vi "VR Controler 9.1.vi"() -> ()   [LabVIEW 2017]
uses:
  Sub VIs/Record enum.ctl
  Sub VIs/Socket enum.ctl
  Sub VIs/Main program enum2.ctl
  <vilib>/vision/Image Controls.llb/IMAQ Image.ctl
  e2139745-3a2d-4eca-8046-712b838de117.vi
  b426bb1a-86ec-4bb9-bfac-d02472307ceb.vi
  58126b9d-de85-4f5f-a9a7-01a9de38026e.vi
  c1239b79-c935-4849-aa75-a73d195e7430.vi
  674a1914-568f-4f25-b0a8-01d8120e0c5f.vi
  5779e0b0-41b7-4506-a67f-138f79383ca8.vi
  75927e18-e53a-4ccd-922e-dca7ab16e00a.vi
  6c211394-beff-4d45-9cac-85fa7b8fa806.vi
  1da1cb31-40b1-4a67-a7e6-56ad72bdf787.vi
  <vilib>/DAQmx/write.llb/DAQmx Write (Digital Bool 1Line 1Point).vi
  eb595f88-4225-414f-83f1-01d5d940fc66.vi
  fb6b5c9d-106e-453b-a883-cc93056fac18.vi
  6235507b-2202-4f21-86ca-b7b41428e472.vi
  835dcb76-40d0-41c5-8fe3-3989c1fd9891.vi
  4796a129-a1f4-4c2b-9c8a-39875efc01cf.vi
  bf4008ee-ae26-4c0a-87de-22156137ce73.vi
  cfabecd4-7210-4e1d-87ea-acbfc879dca4.vi
  ec3ac053-eb45-4274-a63b-aef392164dd0.vi
  b14711bf-09ac-44ea-973e-d3b9cd6138c5.vi
  839eb35e-605d-4d61-b8d1-8b601b76a39a.vi
  4b664865-0372-4337-9de9-faa9f3913aab.vi
  63df5311-9246-4ffc-851f-b70ac2e65be5.vi
  <vilib>/DAQmx/read.llb/DAQmx Read (Analog 2D DBL NChan NSamp).vi
  <vilib>/DAQmx/read.llb/DAQmx Read (Digital 2D U8 NChan NSamp).vi
  <vilib>/DAQmx/read.llb/DAQmx Read (Counter 1D DBL 1Chan NSamp).vi
  <vilib>/DAQmx/create/channels.llb/DAQmx Create Channel (DO-Digital Output).vi
  <vilib>/Utility/file.llb/Read Delimited Spreadsheet (string).vi
  <vilib>/DAQmx/create/channels.llb/DAQmx Create Channel (CO-Pulse Generation-Frequency).vi
  <vilib>/DAQmx/configure/timing.llb/DAQmx Timing (Implicit).vi
  <vilib>/DAQmx/miscellaneous.llb/DAQmx Fill In Error Info.vi
  <vilib>/DAQmx/create/channels.llb/DAQmx Create Channel (AI-Voltage-Basic).vi
  <vilib>/DAQmx/create/channels.llb/DAQmx Create Channel (DI-Digital Input).vi
  <vilib>/DAQmx/configure/timing.llb/DAQmx Timing (Sample Clock).vi
  <vilib>/Utility/file.llb/Write Delimited Spreadsheet (string).vi
  6f1d6b9c-7e66-4bfa-a54a-0bf9111e914d.vi
  <resource>/objmgr/daqmx.rc
  f0a6b648-ccd6-4e98-b62c-d3930b5e7adb.vi
  <vilib>/vision/driver/NI_Vision_Acquisition_Software.lvlib
  fa866b4b-dc6c-4481-bc67-f1512cbbaaf9.vi
  <vilib>/DAQmx/configure/task.llb/DAQmx Configure Logging (TDMS).vi
panel:
  out "Write loop stopped":bool
  out "Read loop stopped":bool
  in  "VR Controller":enum32{"Main panel", "Settings"}(tab)
  out "Frame signal indicator 2":bool
  in  "Timed reward (s)":u32
  in  "Various GUI elements":enum32{"Misc", "Eye tracker", "Security camera"}(tab)
  in  "Stimulus cut off (s)":u32=15
  in  "VR start pos":T1(ring)
  out "Opt stim command":dbl[](graph)
  out "Current stim. protocol":string
  out "Random start pos":bool=TRUE
  out "Next trial stim. protocol":string
  in  "start with ramp":bool
  out "stim loop rate":dbl
  out "Pupille image saved":bool
  in  "Record Button 2":bool
  in  "Black Level":dbl(slide)=0.9896907216494839 min=-32.0 max=31.75 step=1.0 scale=-32.0..32.0
  in  "Gain":dbl(slide)=8.879999999999999 min=0.0 max=24.0 step=1.0 scale=0.0..24.0
  in  "Exposure Time (ms)":dbl(slide)=15144.329896907217 min=1.0 max=15.0 scale=0.0..15.0
  in  "Target frame rate":dbl=60.0 min=1.0 max=144.0 step=1.0
  out "Pupille image":T2(plugin-control)
  out "Frame rate":dbl
  in  "Image Format Control::Offset X":i64(slide) min=0 max=450 step=2 scale=0.0..450.0
  in  "Image Format Control::Offset Y":i64(slide) min=0 max=350 step=2 scale=0.0..350.0
  out "Lost Image Count":u32
  out "Total Images Transferred":u32
  out "Security cam image":T2(plugin-control)
  in  "Cam ON /OFF":bool
  out "Stim. count":i32
  in  "Random reward":bool
  out "Frame signal indicator":bool
  in  "Hybrid licking":bool
  in  "Boolean":bool
  in  "SciScan":bool
  in  "Comment":string
  out "Photodiode":bool
  out "Trial type ettings":enum32{"Page 1", "Page 2"}(tab)
  in  "Auto stop recording":bool
  in  "Shuffle stim trials":bool
  out "Session length":u16 max=100
  in  "Block num. 5":u16
  in  "Block 5":u16(ring) items=["Context A", "Context B", "Context C", "Context D", "Context E", "Context F"]
  in  "Block num. 4":u16
  in  "Block 4":u16(ring) items=["Context A", "Context B", "Context C", "Context D", "Context E", "Context F"]
  in  "Block num. 3":u16
  in  "Block 3":u16(ring) items=["Context A", "Context B", "Context C", "Context D", "Context E", "Context F"]
  in  "Block num. 2":u16
  in  "Block 2":u16(ring) items=["Context A", "Context B", "Context C", "Context D", "Context E", "Context F"]
  in  "Block num. 1":u16=1 min=1
  in  "Block 1":u16(ring) items=["Context A", "Context B", "Context C", "Context D", "Context E", "Context F"]
  in  "stim. num. 5":u16
  in  "Stim. prot 5":u16(ring) items=["none", "none", "continuous from 6 to 180 int. 100 % duty cycle 0 %", "continuous from 10 to 200 int. 100 % duty cycle 0 %", "20 Hz sinus from 10 to 20 int. 100 % duty cycle 0 %", "20 Hz sinus from 10 to 70 int. 100 % duty cycle 0 %", "20 Hz sinus from 10 to 0 int. 100 % duty cycle 0 %", "20 Hz sinus from 0 to 70 int. 100 % duty cycle 0 %", "20 Hz sinus from 0 to 70 int. 50 % duty cycle 0 %", "continuous from 10 to 70 int. 100 % duty cycle 0 %"]
  in  "stim. num. 4":u16
  in  "Stim. prot 4":u16(ring) items=["none", "none", "continuous from 6 to 180 int. 100 % duty cycle 0 %", "continuous from 10 to 200 int. 100 % duty cycle 0 %", "20 Hz sinus from 10 to 20 int. 100 % duty cycle 0 %", "20 Hz sinus from 10 to 70 int. 100 % duty cycle 0 %", "20 Hz sinus from 10 to 0 int. 100 % duty cycle 0 %", "20 Hz sinus from 0 to 70 int. 100 % duty cycle 0 %", "20 Hz sinus from 0 to 70 int. 50 % duty cycle 0 %", "continuous from 10 to 70 int. 100 % duty cycle 0 %"]
  in  "stim. num. 3":u16
  in  "Stim. prot 3":u16(ring) items=["none", "none", "continuous from 6 to 180 int. 100 % duty cycle 0 %", "continuous from 10 to 200 int. 100 % duty cycle 0 %", "20 Hz sinus from 10 to 20 int. 100 % duty cycle 0 %", "20 Hz sinus from 10 to 70 int. 100 % duty cycle 0 %", "20 Hz sinus from 10 to 0 int. 100 % duty cycle 0 %", "20 Hz sinus from 0 to 70 int. 100 % duty cycle 0 %", "20 Hz sinus from 0 to 70 int. 50 % duty cycle 0 %", "continuous from 10 to 70 int. 100 % duty cycle 0 %"]
  in  "stim. num. 2":u16
  in  "Stim. prot 2":u16(ring) items=["none", "none", "continuous from 6 to 180 int. 100 % duty cycle 0 %", "continuous from 10 to 200 int. 100 % duty cycle 0 %", "20 Hz sinus from 10 to 20 int. 100 % duty cycle 0 %", "20 Hz sinus from 10 to 70 int. 100 % duty cycle 0 %", "20 Hz sinus from 10 to 0 int. 100 % duty cycle 0 %", "20 Hz sinus from 0 to 70 int. 100 % duty cycle 0 %", "20 Hz sinus from 0 to 70 int. 50 % duty cycle 0 %", "continuous from 10 to 70 int. 100 % duty cycle 0 %"]
  out "stim. num. 1":u16
  out "Stim. prot 1":u16(ring) items=["none", "none", "continuous from 6 to 180 int. 100 % duty cycle 0 %", "continuous from 10 to 200 int. 100 % duty cycle 0 %", "20 Hz sinus from 10 to 20 int. 100 % duty cycle 0 %", "20 Hz sinus from 10 to 70 int. 100 % duty cycle 0 %", "20 Hz sinus from 10 to 0 int. 100 % duty cycle 0 %", "20 Hz sinus from 0 to 70 int. 100 % duty cycle 0 %", "20 Hz sinus from 0 to 70 int. 50 % duty cycle 0 %", "continuous from 10 to 70 int. 100 % duty cycle 0 %"]
  in  "Trial block":u16 max=100
  in  "Primary masking light":T3(ring)
  in  "Enable stim.":bool
  out "GUI version":enum32{"Page 1", "Page 2"}(tab)
  in  "plot selector 1":u16(ring) items=["Context A", "Context B", "Context C", "Context D", "Context E", "Context F"]
  out "?":dbl(slide) scale=0.0..250.0
  in  "Reset top plot":bool=TRUE caption="Reset"
  in  "Reset bottom plot":bool=TRUE caption="Reset"
  out "P stim. Hit":dbl(slide) scale=0.0..1.0
  out "P ctrl. Hit":dbl(slide) scale=0.0..1.0
  out "Control hit trials %":dbl
  out "Stim. hit trials %":dbl
  out "Next":bool
  out "Top Graph":cluster{"Y":dbl[], "Y":dbl[]}[](graph) caption="XY Graph"
  out "Bottom Graph":cluster{"Y":dbl[], "Y":dbl[]}[](graph) caption="XY Graph"
  in  "plot selector bool 1":bool
  in  "plot selector 2":u16(ring) items=["Context A", "Context B", "Context C", "Context D", "Context E", "Context F"]
  in  "plot selector bool 2":bool
  out "Hit trials %":dbl format="%#.1g"
  out "Hit trials":i32
  out "Wheel position graph":cluster{"Y":dbl[], "Y":dbl[]}[](graph) caption="XY Graph"
  in  "Reset wheel pos. graph":bool=TRUE caption="Reset"
  out "P hit trials":dbl(slide) scale=0.0..1.0
  out "Lick and reward chart 2":cluster{dbl, i16}(graph)
  out "%":dbl format="%#_3g"
  in  "Weight":dbl
  in  "Lab book notes":string
  in  "Open valve":bool
  in  "Reward freq. (cm)":u32
  in  "Reward zone":bool
  out "Distance (m)":dbl format="%#.2g"
  in  "Record Button":bool
  in  "Reset water count":bool
  out "Water received (ul)":dbl
  out "All trials":i32
  out "Ctrl. count":i32
  out "Unique ID":i8 format="%2d"
  in  "Stop recording":bool
  in  "Start recording":bool
  out "Laps":i32
  in  "Exit program":bool
  in  "counter reset (F)":bool caption="stop (F)"
  out "Position on the wheel":dbl(knob) scale=0.0..157.0
  in  "Give reward":bool
  in  "Repetition":i32
  out "Date":string
  out "Run experiment":bool
  out "Velocity chart":dbl(graph)
  out "Lick and reward chart":cluster{dbl, i16}(graph)
  out "Record":bool
  out "Time (min)":dbl format="%#.2g"
  in  "Active licking":bool
  out "Mouse name":string
  in  "Scrollbar":i32(c297)
  out "Velocity chart 2":dbl(graph)
  out "Laser ON":bool
  in  "Extra stop triggers":bool
  out "Tab Control hidden Variables":enum32{"Test charts", "Variables"}(tab)
  in  "Gain  2":dbl
  out "Frame signal 2":i8[](array[numeric])
  out "corridor lengths":i32[](array[numeric])
  out "zeward zones":i16[][](array[numeric])
  out "teleports":i16[](array[numeric])
  out "Stim prot command":u16
  out "Context command":u16
  out "ML signal":sgl[](array[numeric])
  out "Pupil Exp day folder":path
  out "settings folder":path
  out "Eyecam states":T4(ring)
  in  "Eable security cam":bool
  out "Eye cam frame signal":i8[](array[numeric])
  out "prev. max stim. V":dbl
  out "prev. stim. type":string
  out "protocol array":string[][](array[string])
  out "analog lick":sgl[](array[numeric])
  out "Encoder signal":sgl[](array[numeric])
  out "Photo stimulus signal":sgl[](array[numeric])
  out "SciScan start":refnum<k21>
  out "Valve signal":i8[](array[numeric])
  out "Trials in session array":u16[][](array[numeric])
  out "Photodiode signal":sgl[](array[numeric])
  out "Frame signal":i8[](array[numeric])
  out "Filename":string
  out "Lab book file":path
  out "Lick indicator":dbl
  out "Encoder count":dbl
  out "Last saved reward size":dbl
  out "Stim types":u16[](array[numeric])
  out "shuffled array":i16[](array[numeric])
  out "Record loop state":T5
  in  "Record enum":T5
  out "Wheel circumference":dbl
  in  "Recording folder":path
  in  "command line":string
  in  "working directory":path=path ""
  out "Start time":u32
  out "Experiment time (ms)":u32
  out "delta time (s)":dbl format="%#.8g"
  out "reward zone end":dbl
  out "Sample rate":dbl
  out "Loop rate":dbl
  out "No. of smpl. per ch.":i32
  out "Original weight":dbl
  out "Laser stimulus calibration":string
  out "Stimulus protocol":string
  out "prev. diode position":dbl
  out "encoder ticks per rev":dbl
  out "Prev. rew. pos.":dbl
  out "Distance (cm)":dbl
  out "miss trial":bool
  out "Session start:":string
  out "hit trial":bool
  out "2P imaging":string
  out "Security camera":string
  out "velocity (cm/s)":dbl
  out "Masking light prot":string
  out "offset tag":string
  out "random rew":dbl
  out "Track position":sgl
  out "start of stim":bool
  in  "Eable eye cam":bool
  out "stim started":bool
  out "Context types":u16[](array[numeric])
  out "Reward given":u32
  out "current VR context":u16
  out "RZ available":bool
  out "User profile":string
  out "Stop Unity":bool
  out "Exit":bool
  out "Stim trial":bool
  out "Trial counted":bool
  in  "select trial":bool
  in  "VR Mode":bool
  out "delta distance cm":dbl[](array[numeric])
  in  "index":i32
  out "lick signal":i8[](array[numeric])
  out "msg tag":string
  out "Header":string
  out "Unity connected":bool
  out "Masking light":bool
  out "Lick":bool
  out "Valve open":bool
  in  "sound cue presented":bool
  out "read":bool
  out "Write":bool
  out "My tdms file":refnum<k34>
  out "Water cnt. reset":i32
  out "Store prev encoder count":dbl
  out "Start mask stim":bool
  out "Start light stim":bool
  out "Stop light stim":bool
  out "Light ON":bool
  out "Stop mask stim":bool
  out "Hit trials stim.":i32
  out "Hit trials ctrl.":i32
  in  "Software version":string
  out "total distance cm":sgl[](array[numeric])
  out "Experiment time (s)":dbl
  out "Analog 3":sgl[](array[numeric])
  out "Waveform Graph":dynamicdata(graph)
  in  "Duty cycle (%)":u8=50 max=100 step=1
  out "Last calibration":string
  in  "Edit mouse list":bool
  out "Socket read loop rate":u32(graph)
  out "Delta time (ms)":u32(graph)
  in  "Sound duration (ms)":u32=25
  in  "Valve open dur. (ms)":u32=25
  in  "Reward size (ul)":dbl min=0.0 step=inf format="%#.2g"
  in  "working directory 2":path=path ""
  out "Reward read loop rate":u32(graph)
  in  "Current mice":string[][](array[string])
  out "Water count":i32
  in  "Stim protocols":u16(ring) items=["none", "none", "continuous from 6 to 180 int. 100 % duty cycle 0 %", "continuous from 10 to 200 int. 100 % duty cycle 0 %", "20 Hz sinus from 10 to 20 int. 100 % duty cycle 0 %", "20 Hz sinus from 10 to 70 int. 100 % duty cycle 0 %", "20 Hz sinus from 10 to 0 int. 100 % duty cycle 0 %", "20 Hz sinus from 0 to 70 int. 100 % duty cycle 0 %", "20 Hz sinus from 0 to 70 int. 50 % duty cycle 0 %", "continuous from 10 to 70 int. 100 % duty cycle 0 %"]
  in  "Stim type":u16(ring) items=["none", "10 Hz sinus", "20 Hz sinus", "40 Hz sinus", "continuous", "10 Hz square", "20 Hz square", "40 Hz square"]
  in  "Intensity (%)":u8=100 max=100 step=1
  in  "stop (cm)":i32
  in  "start (cm)":i32
  out "Waveform Chart":dbl(graph)
  # "All"
  # "This session"
  # "Reward conditions"
  # "Trial type settings"
  # "Hit trials:"
  # "%"
  # "Hit trials:"
  # "%"
  # "%"
  # "Edit stimulus protocols for photo stimulation and/or \na secondary masking light. Chose a protocol from the \nlist and define parameters."
  # "Reward settings"
  # "Mouse name               Headbar           Original weight"
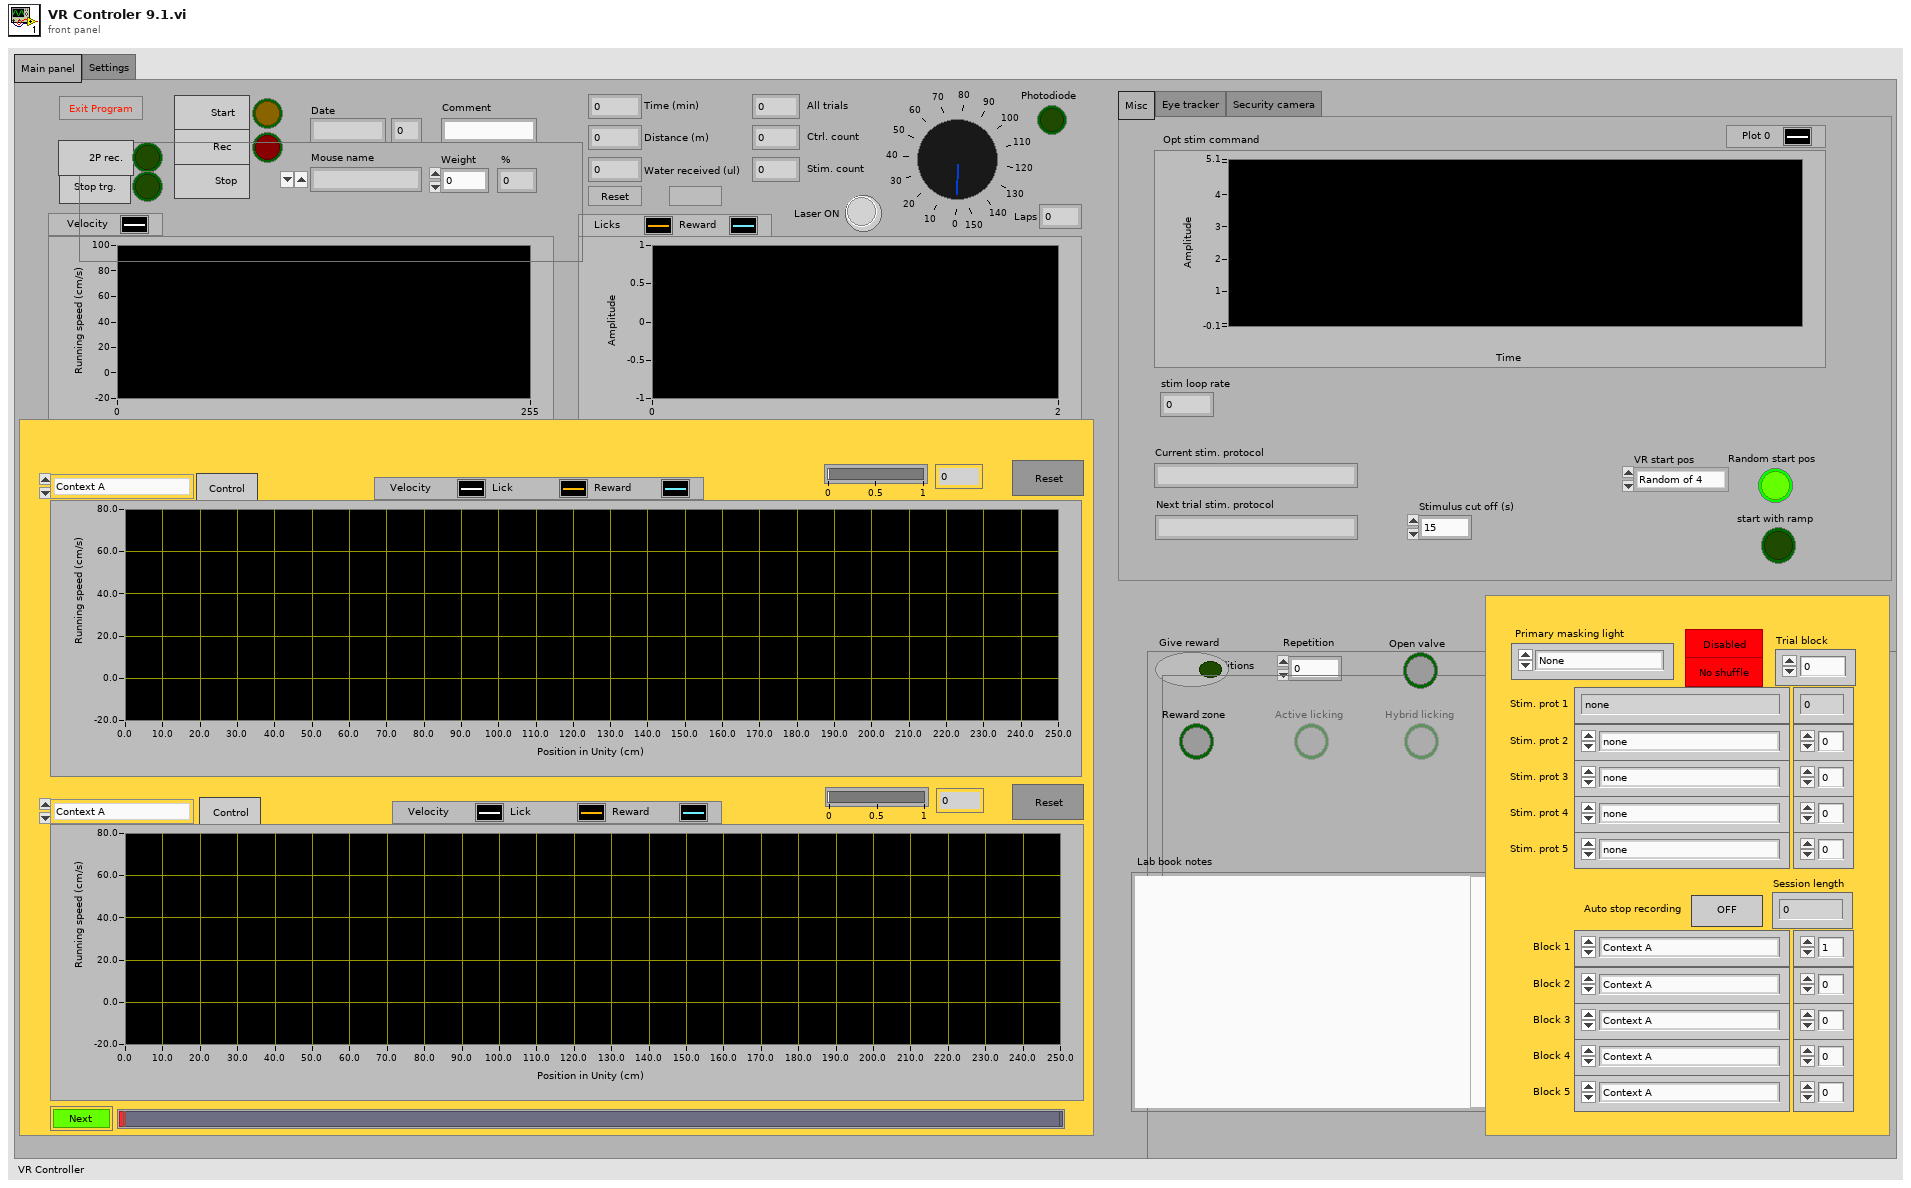
[diagram p1: front panel]
types:
  T1 = enum16{"Random of 4", "Random of 2", "Non-random"}
  T2 = typedef "IMAQ Image.ctl" = refnum<image>
  T3 = enum16{"None", "20 Hz until reward ", "Continuous specified light off trials", "Continuous specified all trials", "20 Hz specified light off trials", "20 Hz specified all trials", "20 Hz full trial", "Continuous full trial"}
  T4 = enum16{"Idle", "Set params", "Start recording", "Record pupille", "Stop recording"}
  T5 = typedef "Record enum.ctl" = enum16{"Idle", "Init recording", "Init data acquisition", "Record VR", "Record", "Stop data acquision"}
  T6 = enum8{"Enabled", "Disabled", "Disabled and Grayed Out"}
  T7 = typedef "Main program enum2.ctl" = enum16{"Init program", "Idle", "Init recording ", "Record", "Record VR", "Stop Recording", "Exit program"}
  T8 = typedef "Socket enum.ctl" = enum16{"Socket not connected", "Init socket", "Socket connected", "Close socket"}
  T9 = cluster{"Type":u32, "Version":u32, "Flags":u32, "SerialNumberHigh":u32, "SerialNumberLow":u32, "BusType":u32, "InterfaceName":string, "VendorName":string, "ModelName":string, "CameraFileName":string, "CameraAttributeURL":string}[]
  T10 = enum16{"open", "replace", "create", "open or create", "replace or create", "replace or create with confirmation"}
  T11 = enum16{"Init program", "Idle", "Init recording ", "Record", "Record VR", "Stop Recording", "Exit program"}
  T12 = enum16{"None", "Full trial 40 Hz sinus ", "Full trial 20 Hz sinus", "Continuous light ON", "Until reward 40 Hz sinus"}
  T13 = enum16{"None", "20 Hz until reward ", "Continuous specified light off trials", "Continuous specified all trials", "20 Hz specified light off trials", "20 Hz specified all trials"}
  T14 = typedef "LVStringsAndValuesArrayTypeDef_U16.ctl" = cluster{"String":string, "Value":u16}[]
  T15 = enum16{"open", "open or create", "create or replace", "create", "open (read-only)"}
  T16 = enum16{"Standard", "Buffered", "CRLF", "Immediate"}
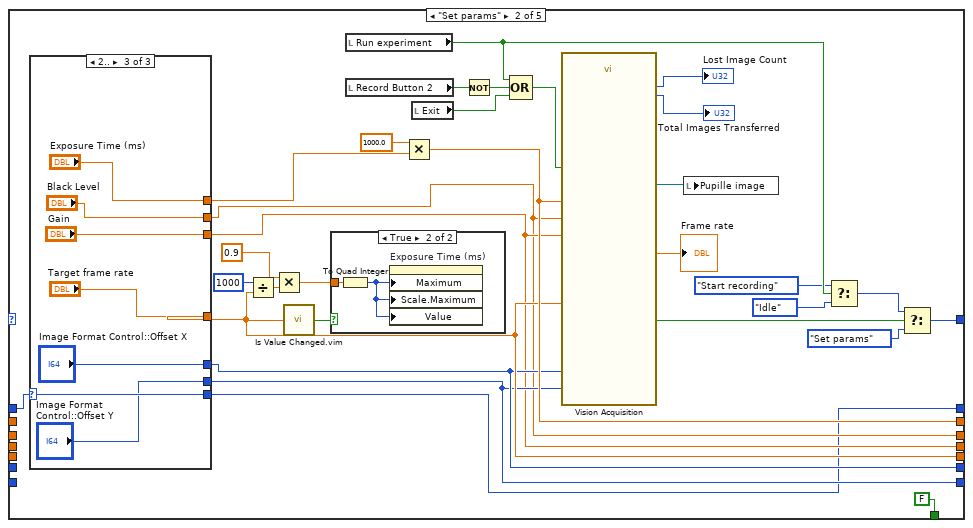
[diagram p3: hidden frame]
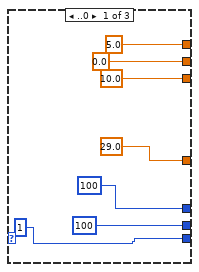
[diagram p4: hidden frame]
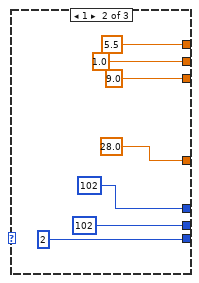
[diagram p5: hidden frame]
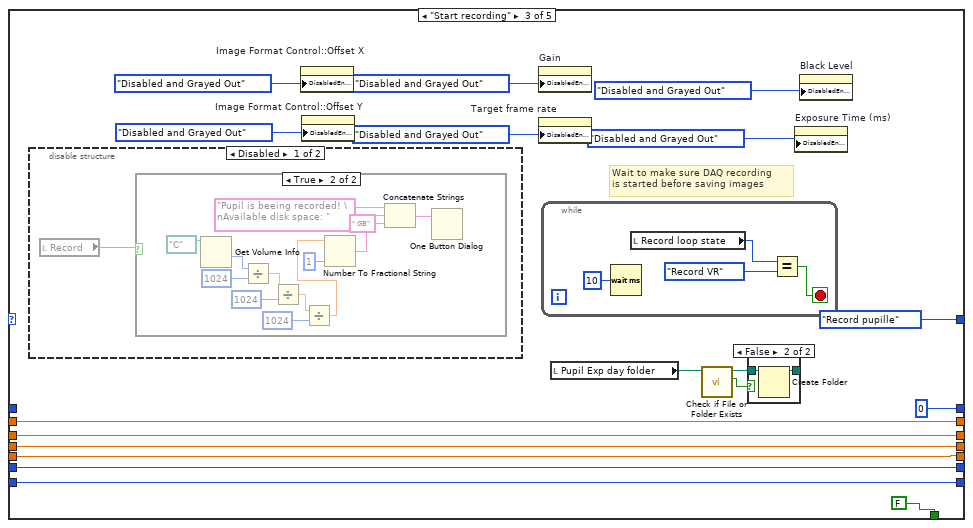
[diagram p7: hidden frame]
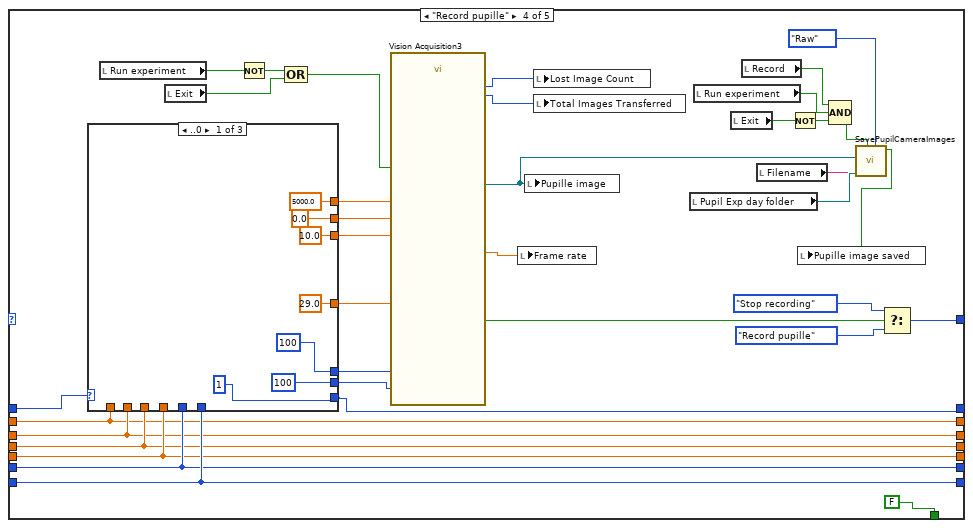
[diagram p11: hidden frame]
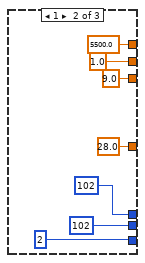
[diagram p12: hidden frame]
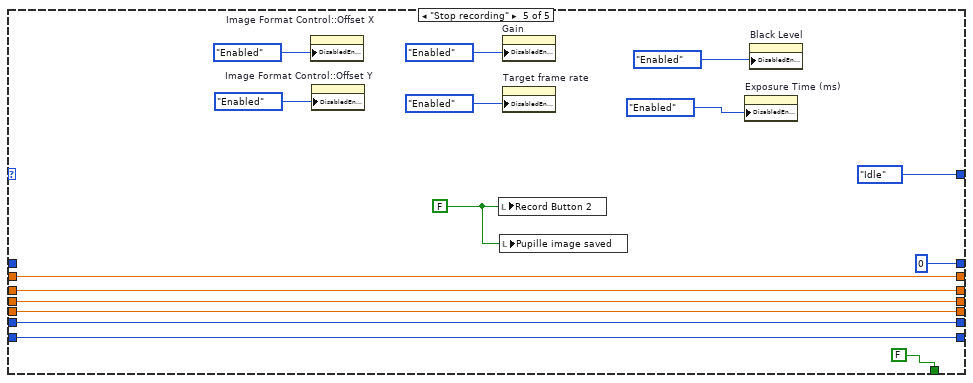
[diagram p14: hidden frame]
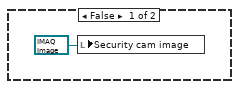
[diagram p15: hidden frame]
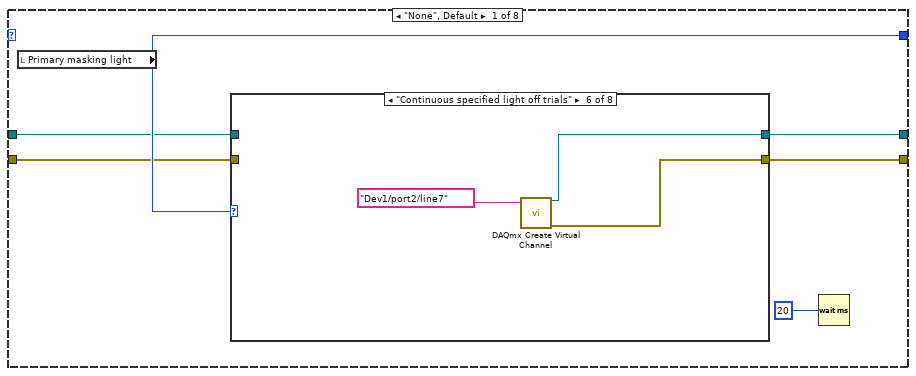
[diagram p19: hidden frame]
diagram:
  w5 = T6."Enabled" ("Disabled")
  w15 = FALSE ("Eable eye cam")
  w16 = FALSE ("Record Button 2")
  w17 = 60 ("y")
  w43 = "rew" ("regular expression")
  w41 = "rew" ("regular expression")
  w35 = "continuous" ("regular expression")
  w37 = "none" ("regular expression")
  w55 = "rew" ("regular expression")
  w57 = "rew" ("regular expression")
  w63 = "continuous" ("regular expression")
  w61 = "none" ("regular expression")
  (unwired) string[] ["Photo-diode", "Time (s)", "Delta Time (ms)", "Distance (cm)", "Valve open", "Frame signal", "Lick signal", "Photo stimulus signal", "Laser ON", "Position in Unity", "Corridor indicator"] ("channel name(s) in (Untitled)")
  w80 = FALSE ("Reset")
  # "Defaults"
  # "Keep order of default variables:\nUser:\tMate\nLoop rate:\t100\nSampling rate:\t3000\nEncoder tisks:\t4000\nRecording folder:\tC:\\Users\\vrsetup\\Desktop\nEnable VR more(Y/N):\tY\n..."
  # "File versions:\n-8.5 User profile selector\n\n-8.3 Camera control added> Pupil imaging and security camera\nTimed reward\n\n-8.2 with 8.4 unity version: \nNew task without cue\nImportant bugfixes in photo-stimulation, start stimulus with ramp option is added\nSafety switch shuts off stimulus after 10s \n\n-8.0 - 8.2\nNew task wersionm new optogenetic prorocol solutions\n\n-7.5 - 2019.07.10\nRandom reward option\n\n-7.5\nNew Unity version: coupling error is corrected! (interpolation factor discarded), randomizeable starting point.\nTiki-taka task for Nora\nNew masking light functions : 20Hz specified in light off or all trials\n\n\n-7.3\nMasking light options are added\nMasking light protocol is saved now in labbook\n\n-7.2\nmade GitHub compatible: folder path and some default variables are red from txt file and txt data files are now in separate folder\ndate is formated with different method\n\n-7.1\nsaves Encoder signal and imaging/security camera YES NO indication is added to lab book\nsaves Analog lick signal\n\n-7.0 \nMasking light\n\n-6.9\nData typed are changed back to DBL\n\n-6.8\nDifferent data saving settings to reduce file size by specifying data types\nCorrect trial % corrected after 2018.12.05\nHybrid licking\nPhoto stimulus trials and counting of \"Hit trials \"for Nora\n\n-6.7 \nfor Mate Loop rate from 200 -> 100 Hz  (should not affect VR that is 60 Hz) \nrecorded sampling rate increased 200 -> 3000 Hz\nswitch to show water consumption in current session is added\n\n\n\n..."
  n1 = flat-sequence {
    tunnel: [w118] -> w11
    tunnel: w11 -> [w154]
    tunnel: [Socket_enum."Socket not connected" ("Enum")] -> w112
    tunnel: [Main_program_enum2."Init program" ("main program")] -> w111
    tunnel: [Record_enum."Idle" ("Record enum")] -> w108
    tunnel: [TRUE ("VR Mode")] -> w79
    frame #0 {
      # "Select user profile"
      n2 = call <vilib>:"Recursive File List.vi"("Folder Path"=path "C:/VR Controller/data" ("path")) -> ("All Folders"=w127:path[])  [unwired: 6 in, 4 out]
      n3 = Array Size(array=w127) -> (size(s)=w132:i32)
      n4 = for {
        N: w132 -> [_]
        tunnel: w127 -> [w143] mode=indexing
        shift-right: [w140] -> w129
        shift-left: string[] [] -> [w139]
        i -> [w141]
        n5 = Strip Path(path=w143) -> (name=w142:string)  [unwired: 1 out]
        n6 = Insert Into Array(array=w139, index=w141, new element=w142) -> (w140:string[])
      }
      n7 = Array Size(array=w129) -> (size(s)=w121:i32)
      n8 = Greater?(x=w121, y=1) -> (0:w119:bool)
      n9 = Array Subset(array=w129, index=1, length=w121) -> (w128:string[])
      n10 = case shown="True" w119 {
        tunnel: w128 -> [_ w138]
        tunnel: w127 -> [_ w137]
        tunnel: [path "" ("path") w134] -> w123
        frame False {
        }
        frame True {
          n11 = call "Get User Input.vi"("Strings []"=w138) -> ("user"=w136:u16)  [unwired: 1 in, 9 out]
          n12 = Increment(x=w136) -> (x+1=w135:u16)
          n13 = Index Array(array=w137, index=w135) -> (element=w134:path)
        }
      }
      n14 = Equal?(x=w123, y=path "" ("path")) -> (x = y?=w125:bool)
      n15 = Select(t=path "C:/VR Controller/data", s=w125, f=w123) -> (s? t:f=w118:path)
      "settings folder" <- w118
      n16 = Path To String(path=w118) -> (string=w117:string)
      n17 = Match Pattern(string=w117, regular expression="data\\") -> (after substring=→"User profile":string)  [unwired: 1 in, 3 out]
    }
    frame #1 {
      w159 = 1 ("length")
      w164 = 1 ("length")
      w177 = 1 ("length")
      w180 = 1 ("length")
      w183 = 1 ("length")
      w186 = 1 ("length")
      # "VI version"
      # "Enable VR mode"
      n18 = Build Path(base path=w154, name or relative path="Default variables.txt") -> (appended path=w152:path)
      n19 = call-poly <vilib>:"Read Delimited Spreadsheet.vi"("file path (dialog if empty)"=w152) -> ("all rows"=w155:string[][])  [unwired: 9 in, 5 out]
      n20 = Array Subset(array=w155, index (row)=0 ("index"), length (row)=w186, index (col)=w186, length (col)=w186) -> (w185:string[][])
      n21 = Array Subset(array=w155, index (row)=1 ("index"), length (row)=w183, index (col)=w183, length (col)=w183) -> (w184:string[][])
      n22 = Array Subset(array=w155, index (row)=2 ("index"), length (row)=w164, index (col)=w164, length (col)=w164) -> (w161:string[][])
      n23 = Array Subset(array=w155, index (row)=3 ("index"), length (row)=w180, index (col)=w180, length (col)=w180) -> (w179:string[][])
      n24 = Array Subset(array=w155, index (row)=4 ("index"), length (row)=w177, index (col)=w177, length (col)=w177) -> (w178:string[][])
      n25 = Array Subset(array=w155, index (row)=5 ("index"), length (row)=w159, index (col)=w159, length (col)=w159) -> (w158:string[][])
      n26 = Concatenate Strings(w185) -> (w171:string)
      n27 = Concatenate Strings(w184) -> (w173:string)
      n28 = Concatenate Strings(w161) -> (w165:string)
      n29 = Concatenate Strings(w179) -> (w174:string)
      n30 = Concatenate Strings(w178) -> (w175:string)
      n31 = Concatenate Strings(w158) -> (w157:string)
      n32 = String To Path(string=w175) -> (path=w148:path)
      n33 = Fract/Exp String To Number(string=w165) -> (number=w162:dbl)  [unwired: 3 in, 1 out]
      n34 = Fract/Exp String To Number(string=w174) -> (number=w169:dbl)  [unwired: 3 in, 1 out]
      n35 = Fract/Exp String To Number(string=w173) -> (number=w170:dbl)  [unwired: 3 in, 1 out]
      n36 = Equal?(x=w171, y=" ") -> (x = y?=w146:bool)
      n37 = Equal?(x=w157, y="Y") -> (x = y?=w145:bool)
      n38 = case shown="True" w145 {
        tunnel: w155 -> [_ w195]
        tunnel: [path "" w198] -> w147
        frame False {
          (unwired) FALSE ("T button?")
        }
        frame True {
          w196 = 1 ("length")
          w202 = 1 ("length")
          # "Default context"
          n39 = Array Subset(array=w195, index (row)=6 ("index"), length (row)=w202, index (col)=w202, length (col)=w202) -> (w200:string[][])
          n40 = Array Subset(array=w195, index (row)=7 ("index"), length (row)=w196, index (col)=w196, length (col)=w196) -> (w194:string[][])
          n41 = Concatenate Strings(w200) -> (w199:string)
          n42 = Concatenate Strings(w194) -> (w193:string)
          n43 = local write "command line"(w199) -> ()
          n44 = String To Path(string=w199) -> (path=w198:path)
          n45 = Decimal String To Number(string=w193) -> (number=w192:i32)  [unwired: 2 in, 1 out]
          n46 = local write "Block 1"(w192) -> ()
          n47 = local write "plot selector 1"(w192) -> ()
        }
      }
      n48 = local write "Loop rate"(w170) -> ()
      n49 = local write "Sample rate"(w162) -> ()
      n50 = local write "encoder ticks per rev"(w169) -> ()
      n51 = local write "Recording folder"(w148) -> ()
      n52 = case shown="True" w146 {
        frame False {
          n53 = local write "Sound duration (ms)"(u32 0 ("Sound duration (ms)")) -> ()
        }
        frame True {
          n54 = local write "Sound duration (ms)"(u32 0 ("Sound duration (ms)")) -> ()
        }
      }
      n55 = local write "VR Mode"(w145) -> ()
      n56 = Current VI's Path() -> (path=w151:path)
      n57 = case shown="True" TRUE {
        tunnel: [enum32{"Page 1", "Page 2"}."Page 2" ("GUI version") w233] -> w189
        tunnel: [enum32{"Page 1", "Page 2"}."Page 1" ("GUI version") w233] -> w188
        frame False {
          n58 = property on="Top Graph" class="XYGraph (strict)"("DisabledEnum"=T6."Disabled" ("Disabled")) -> ()  [unwired: 2 in, 2 out]
          n59 = property on="Bottom Graph" class="XYGraph (strict)"("DisabledEnum"=T6."Disabled" ("Disabled")) -> ()  [unwired: 2 in, 2 out]
          n60 = property on="Wheel position graph" class="XYGraph (strict)"("DisabledEnum"=T6."Enabled" ("Disabled")) -> ()  [unwired: 2 in, 2 out]
          n61 = property on="Lick and reward chart" class="WFChart (strict)"("Visible"=FALSE, "DisabledEnum"=T6."Disabled" ("Disabled")) -> ()  [unwired: 2 in, 2 out]
          n62 = property on="Velocity chart" class="WFChart (strict)"("Visible"=FALSE, "DisabledEnum"=T6."Disabled" ("Disabled")) -> ()  [unwired: 2 in, 2 out]
          n63 = property on="Reset top plot" class="Bool (strict)"("DisabledEnum"=T6."Disabled" ("Disabled")) -> ()  [unwired: 2 in, 2 out]
          n64 = property on="Reset wheel pos. graph" class="Bool (strict)"("DisabledEnum"=T6."Enabled" ("Disabled")) -> ()  [unwired: 2 in, 2 out]
          n65 = property on="Reset bottom plot" class="Bool (strict)"("DisabledEnum"=T6."Disabled" ("Disabled")) -> ()  [unwired: 2 in, 2 out]
          n66 = property on="Lick and reward chart 2" class="WFChart (strict)"("Visible"=TRUE, "DisabledEnum"=T6."Enabled" ("Disabled")) -> ()  [unwired: 2 in, 2 out]
          n67 = property on="Velocity chart 2" class="WFChart (strict)"("Visible"=TRUE, "DisabledEnum"=T6."Enabled" ("Disabled")) -> ()  [unwired: 2 in, 2 out]
        }
        frame True {
          w233 = enum32{"Page 1", "Page 2"}."Page 1" ("GUI version")
          n68 = property on="Lick and reward chart" class="WFChart (strict)"("Visible"=TRUE, "DisabledEnum"=T6."Enabled" ("Disabled")) -> ()  [unwired: 2 in, 2 out]
          n69 = property on="Velocity chart" class="WFChart (strict)"("Visible"=TRUE, "DisabledEnum"=T6."Enabled" ("Disabled")) -> ()  [unwired: 2 in, 2 out]
          n70 = property on="Top Graph" class="XYGraph (strict)"("DisabledEnum"=T6."Enabled" ("Disabled")) -> ()  [unwired: 2 in, 2 out]
          n71 = property on="Bottom Graph" class="XYGraph (strict)"("DisabledEnum"=T6."Enabled" ("Disabled")) -> ()  [unwired: 2 in, 2 out]
          n72 = property on="Wheel position graph" class="XYGraph (strict)"("DisabledEnum"=T6."Disabled" ("Disabled")) -> ()  [unwired: 2 in, 2 out]
          n73 = property on="Reset top plot" class="Bool (strict)"("DisabledEnum"=T6."Enabled" ("Disabled")) -> ()  [unwired: 2 in, 2 out]
          n74 = property on="Reset wheel pos. graph" class="Bool (strict)"("DisabledEnum"=T6."Disabled" ("Disabled")) -> ()  [unwired: 2 in, 2 out]
          n75 = property on="Reset bottom plot" class="Bool (strict)"("DisabledEnum"=T6."Enabled" ("Disabled")) -> ()  [unwired: 2 in, 2 out]
          n76 = property on="Lick and reward chart 2" class="WFChart (strict)"("Visible"=FALSE, "DisabledEnum"=T6."Disabled" ("Disabled")) -> ()  [unwired: 2 in, 2 out]
          n77 = property on="Velocity chart 2" class="WFChart (strict)"("Visible"=FALSE, "DisabledEnum"=T6."Disabled" ("Disabled")) -> ()  [unwired: 2 in, 2 out]
        }
      }
      "GUI version" <- w189
      "Trial type ettings" <- w188
      n78 = Strip Path(path=w147) -> (name=w149:string)  [unwired: 1 out]
      n79 = Strip Path(path=w151) -> (name=w150:string)  [unwired: 1 out]
      n80 = disable-structure shown="Disabled" {
        frame Disabled {
          n81 = local write "command line"("C:\\VR Controller\\corridor1\\LVcontrol_6.exe" ("command line")) -> ()
        }
        frame Enabled {
        }
      }
      n82 = case shown="True" w145 {
        tunnel: ["" ("string") w205] -> w167
        tunnel: w149 -> [_ w204]
        frame False {
        }
        frame True {
          n83 = Concatenate Strings(";    Unity VR version: " ("string"), w204) -> (w205:string)
        }
      }
      n84 = Concatenate Strings(w150, w167, "" ("string")) -> (w168:string)
      n85 = local write "Software version"(w168) -> ()
    }
    frame #2 {
      # "Has to be integer!"
      n86 = call <vilib>:"IMAQdx Enumerate Cameras.vi"() -> ("Camera Information Array"=w243:T9)  [unwired: 10 in, 1 out]
      n87 = local read "Sample rate"() -> (w242:dbl)
      n88 = for {
        tunnel: w243 -> [w255] mode=indexing
        # "Eye camera available"
        # "Security camera available"
        n89 = Unbundle By Name(w255) -> ("VendorName"=w252:string)
        n90 = Equal?(x="Microsoft® LifeCam Studio(TM)", y=w252) -> (x = y?=w250:bool)
        n91 = Equal?(x=w252, y="Basler") -> (x = y?=w251:bool)
        n92 = case shown="True" w250 {
          selector: w250 -> [_ w256]
          frame False {
          }
          frame True {
            n93 = local write "Eable security cam"(w256) -> ()
            n94 = property on="Cam ON /OFF" class="Bool (strict)"("DisabledEnum"=T6."Enabled" ("Disabled")) -> ()  [unwired: 2 in, 2 out]
          }
        }
        n95 = case shown="True" w251 {
          selector: w251 -> [_ w258]
          frame False {
          }
          frame True {
            n96 = local write "Eable eye cam"(w258) -> ()
            n97 = property on="Record Button 2" class="Bool (strict)"("DisabledEnum"=T6."Enabled" ("Disabled")) -> ()  [unwired: 2 in, 2 out]
          }
        }
      }
      n98 = local read "Loop rate"() -> (w246:dbl)
      n99 = Divide(x=w242, y=w246) -> (x/y=w247:dbl)
      n100 = Divide(x=1.0, y=w242) -> (x/y=w240:dbl)
      n101 = local write "No. of smpl. per ch."(w247) -> ()
      n102 = property on="Opt stim command" class="WFChart (strict)"("XScale.Multiplier"=w240) -> ()  [unwired: 2 in, 2 out]
    }
  }
  n103 = property on="Software version" class="Str"("Visible"=TRUE) -> ()  [unwired: 2 in, 2 out]
  n104 = disable-structure shown="Disabled" {
    frame Disabled {
      n105 = call-poly <vilib>:"DAQmx Configure Logging.vi"() -> ()  [unwired: 14 in, 2 out]
    }
    frame Enabled {
    }
  }
  n106 = disable-structure shown="Disabled" {
    frame Disabled {
      n107 = local read "Unity connected"() -> (w260:bool)
      n108 = case shown="False" w260 {
        frame False {
          n109 = case shown="True" {
            selector: _ -> [_ _]
            frame False {
            }
            frame True {
              n110 = call <vilib>:"System Exec.vi"("wait until completion? (T)"=FALSE, "working directory"="working directory", "command line"="command line") -> ()  [unwired: 5 in, 4 out]
              n111 = Wait (ms)(milliseconds to wait=u32 1000) -> ()  [unwired: 1 out]
            }
          }
        }
        frame True {
        }
      }
    }
    frame Enabled {
    }
  }
  n112 = local write "Eable security cam"(w15) -> ()
  n113 = local write "Eable eye cam"(w15) -> ()
  n114 = property on="Cam ON /OFF" class="Bool (strict)"("DisabledEnum"=T6."Disabled and Grayed Out" ("Disabled")) -> ()  [unwired: 2 in, 2 out]
  n115 = property on="Record Button 2" class="Bool (strict)"("DisabledEnum"=T6."Disabled and Grayed Out" ("Disabled")) -> ()  [unwired: 2 in, 2 out]
  n116 = local write "msg tag"("str," ("msg tag")) -> ()
  n117 = local write "Security camera"("Security camera: NO" ("Security camera")) -> ()
  n118 = Multiply(x=50.0, y=3.141592653589793) -> (x*y=→"Wheel circumference":dbl)
  n119 = Divide(x=1000, y=w17) -> (x/y=w19:dbl)
  n120 = property on="lick signal" class="Arr (strict)"("Visible"=TRUE) -> ()  [unwired: 2 in, 2 out]
  n121 = property on="Header" class="Str"("Visible"=TRUE) -> ()  [unwired: 2 in, 2 out]
  n122 = disable-structure shown="Disabled" {
    frame Disabled {
      n123 = Add Array Elements() -> (numeric array=w267:dbl[], sum=w266:dbl)
      n124 = Array Size(array=w267) -> (size(s)=w265:i32)
      n125 = Divide(x=w266, y=w265) -> ()  [unwired: 1 out]
    }
    frame Enabled {
    }
  }
  n126 = local write "Target frame rate"(w17) -> ()
  n127 = local write "Write loop stopped"(TRUE ("Read loop stopped")) -> ()
  n128 = local write "Read loop stopped"(TRUE ("Read loop stopped")) -> ()
  n129 = property on="Read loop stopped" class="Bool (strict)"("Visible"=FALSE) -> ()  [unwired: 2 in, 2 out]
  n130 = property on="Write loop stopped" class="Bool (strict)"("Visible"=FALSE) -> ()  [unwired: 2 in, 2 out]
  n131 = Multiply(x=0.9, y=w19) -> (x*y=w21:dbl)
  n132 = local write "Recording folder"("Recording folder") -> ()
  n133 = To Quad Integer(1:w21) -> (0:w22:i64)
  n134 = Get Date/Time String(date format (0)=enum16{"short", "long", "abbreviated"}."short") -> ()  [unwired: 2 in, 2 out]
  n135 = property on="delta distance cm" class="DigNum (strict)"("Visible"=TRUE) -> ()  [unwired: 2 in, 2 out]
  n136 = local write "Encoder count"(0.0 ("Encoder count")) -> ()
  n137 = property on="Lab book file" class="Path"("Visible"=TRUE) -> ()  [unwired: 2 in, 2 out]
  n138 = local write "Record Button 2"(w16) -> ()
  n139 = local write "Pupille image saved"(w16) -> ()
  n140 = property on="index" class="DigNum (strict)"("Visible"=TRUE) -> ()  [unwired: 2 in, 2 out]
  n141 = property on="Exposure Time (ms)" class="Slide (strict)"("Maximum"=w22, "Scale.Maximum"=w22, "Value"=w22) -> ()  [unwired: 2 in, 2 out]
  n142 = while {
    shift-right: [w268] -> _
    shift-left: w111 -> [w270]
    stop <- w271 stop-if-true
    n143 = case shown="\"Init recording \"" w270 {
      tunnel: [T11."Idle" ("main program") w475 w766 T11."Idle" ("main program") T11."Idle" ("main program") w878 w973] -> w268
      frame "Init program", Default {
        w273 = 1 ("y")
        (unwired) path "C:/Users/Mate Neubrandt/Desktop/test/Task config" ("path")
        w319 = u16 0 items=["none"] ("Stim. prot 1")
        w320 = u16 0 ("stim. num. 2")
        n144 = local read "settings folder"() -> (w316:path)
        n145 = local write "Unique ID"(i8 0 ("Unique ID")) -> ()
        n146 = local write "Run experiment"(FALSE ("Record")) -> ()
        n147 = local write "SciScan"(FALSE ("SciScan")) -> ()
        n148 = local write "Edit mouse list"(FALSE ("Edit mouse list")) -> ()
        n149 = local write "Trial block"(u16 10 ("Denominator")) -> ()
        n150 = Build Path(base path=w316, name or relative path="List of mice.txt") -> (appended path=w315:path)
        n151 = property on="Stop recording" class="Bool (strict)"("DisabledEnum"=T6."Disabled" ("Disabled")) -> ()  [unwired: 2 in, 2 out]
        n152 = call-poly <vilib>:"DAQmx Create Virtual Channel.vi"("lines"=tag "Dev1/port0/line0") -> ("task out"=→"SciScan start":refnum<k21>)  [unwired: 13 in, 1 out]
        n153 = call-poly <vilib>:"Read Delimited Spreadsheet.vi"("file path (dialog if empty)"=w315) -> ("all rows"=w341:string[][])  [unwired: 9 in, 5 out]
        n154 = local write "stim. num. 2"(w320) -> ()
        n155 = local write "stim. num. 3"(w320) -> ()
        n156 = local write "stim. num. 4"(w320) -> ()
        n157 = local write "stim. num. 5"(w320) -> ()
        n158 = local write "Block num. 2"(w320) -> ()
        n159 = local write "Block num. 3"(w320) -> ()
        n160 = local write "Block num. 4"(w320) -> ()
        n161 = local write "Block num. 5"(w320) -> ()
        n162 = local write "Current mice"(w341) -> ()
        n163 = flat-sequence {
          frame #0 {
            n164 = property on="Stim protocols" class="Ring (strict)"("Strings []"=string[] []) -> ()  [unwired: 2 in, 2 out]
          }
          frame #1 {
            n165 = local read "settings folder"() -> (w346:path)
            n166 = Build Path(base path=w346, name or relative path="Stimprotocols.txt") -> (appended path=w344:path)
            n167 = call-poly <vilib>:"Read Delimited Spreadsheet.vi"("file path (dialog if empty)"=w344) -> ("all rows"=w349:string[][])  [unwired: 9 in, 5 out]
            "protocol array" <- w349
            n168 = Array Size(array=w349) -> (size(s)=w352:i32[])
            n169 = Index Array(array=w352, index=0) -> (element=w350:i32)
            n170 = for {
              N: w350 -> [_]
              tunnel: w349 -> [w363] mode=indexing
              shift-right: [w361] -> w347
              shift-left: string[] [] -> [w360]
              i -> [w362]
              n171 = Concatenate Strings(w363) -> (w357:string)
              n172 = Match Pattern(string=w357, regular expression="none") -> (before substring=w355:string, match substring=w354:string)  [unwired: 1 in, 2 out]
              n173 = Not Equal?(x=w354, y="none") -> (x != y?=w356:bool)
              n174 = Select(t=w355, s=w356, f=w354) -> (s? t:f=w353:string)
              n175 = Insert Into Array(array=w360, index=w362, new element=w353) -> (w361:string[])
            }
            n176 = property on="Stim protocols" class="Ring (strict)"("Strings []"=w347) -> ()  [unwired: 2 in, 2 out]
          }
        }
        n177 = local write "Enable stim."(TRUE ("Enable stim.")) -> ()
        n178 = local write "Stim. prot 2"(w319) -> ()
        n179 = local write "Stim. prot 3"(w319) -> ()
        n180 = local write "Stim. prot 4"(w319) -> ()
        n181 = local write "Stim. prot 5"(w319) -> ()
        n182 = local write "Block 2"(w319) -> ()
        n183 = local write "Block 3"(w319) -> ()
        n184 = local write "Block 4"(w319) -> ()
        n185 = local write "Block 5"(w319) -> ()
        n186 = local read "command line"() -> (w303:string)
        n187 = local read "settings folder"() -> (w279:path)
        n188 = local read "settings folder"() -> (w314:path)
        n189 = Build Path(base path=w279, name or relative path="Task configuration.txt") -> (appended path=w278:path)
        n190 = Match Pattern(string=w303, regular expression=".exe") -> (before substring=w301:string)  [unwired: 1 in, 3 out]
        n191 = call-poly <vilib>:"Read Delimited Spreadsheet.vi"("file path (dialog if empty)"=w278) -> ("all rows"=w310:string[][])  [unwired: 9 in, 5 out]
        n192 = Concatenate Strings(w301, "_config" ("string")) -> (w299:string)
        n193 = Build Path(base path=w314, name or relative path="Last calibration.txt") -> (appended path=w312:path)
        n194 = Build Path(name or relative path=w299) -> ()  [unwired: 1 in, 1 out]
        n195 = Delete From Array(array=w310, length=1, index (col)=0 ("disabled index (col)")) -> (deleted portion=w307:string[][], array with subset deleted=w296:string[][])  [unwired: 1 in]
        n196 = Decimal String To Number(string=w296) -> (number=w293:i32[][])  [unwired: 2 in, 1 out]
        n197 = Array Size(array=w307) -> (size(s)=w306:i32[])
        n198 = Open/Create/Replace File(file path (use dialog)=w312, operation (0:open)=T10."open", access (0:read/write)=enum16{"read/write", "read-only", "write-only"}."read-only") -> (refnum out=w331:refnum<file>)  [unwired: 3 in, 2 out]
        n199 = Index Array(array=w306, index=0) -> (element=w304:i32)
        n200 = Delete From Array(array=w293, length=1, index (col)=0 ("disabled index (col)")) -> (deleted portion=w288:i32[][], array with subset deleted=w292:i32[][])  [unwired: 1 in]
        n201 = Read from Text File(file (use dialog)=w331) -> (refnum out=w332:refnum<file>, text=w333:string)  [unwired: 3 in, 2 out]
        n202 = Reshape Array(w307, w304) -> (w277:string[])
        n203 = local write "Last calibration"(w333) -> ()
        n204 = Match Pattern(string=w333, regular expression=" ul") -> (before substring=w335:string)  [unwired: 1 in, 3 out]
        n205 = Match Pattern(string=w333, regular expression="ul / ") -> (after substring=w334:string)  [unwired: 1 in, 3 out]
        n206 = property on="Block 1" class="Ring (strict)"("Strings []"=w277) -> ()  [unwired: 2 in, 2 out]
        n207 = property on="Block 2" class="Ring (strict)"("Strings []"=w277) -> ()  [unwired: 2 in, 2 out]
        n208 = property on="Block 3" class="Ring (strict)"("Strings []"=w277) -> ()  [unwired: 2 in, 2 out]
        n209 = property on="Block 4" class="Ring (strict)"("Strings []"=w277) -> ()  [unwired: 2 in, 2 out]
        n210 = property on="Block 5" class="Ring (strict)"("Strings []"=w277) -> ()  [unwired: 2 in, 2 out]
        n211 = Delete From Array(array=w292, length=1, index (col)=0 ("disabled index (col)")) -> (deleted portion=w282:i32[][], array with subset deleted=→"zeward zones":i32[][])  [unwired: 1 in]
        n212 = Close File(refnum=w332) -> ()  [unwired: 1 in, 2 out]
        n213 = Fract/Exp String To Number(string=w335) -> (number=w336:dbl)  [unwired: 3 in, 1 out]
        "Last saved reward size" <- w336
        n214 = Match Pattern(string=w334, regular expression=" ms ") -> (before substring=w337:string)  [unwired: 1 in, 3 out]
        n215 = Array Size(array=w288) -> (size(s)=w289:i32[])
        n216 = Array Size(array=w282) -> (size(s)=w284:i32[])
        n217 = local write "Reward size (ul)"(w336) -> ()
        n218 = property on="plot selector 1" class="Ring (strict)"("Strings []"=w277) -> ()  [unwired: 2 in, 2 out]
        n219 = Decimal String To Number(string=w337) -> (number=w338:i32)  [unwired: 2 in, 1 out]
        n220 = property on="plot selector 2" class="Ring (strict)"("Strings []"=w277) -> ()  [unwired: 2 in, 2 out]
        n221 = Index Array(array=w289, index=0) -> (element=w287:i32)
        n222 = Index Array(array=w284, index=0) -> (element=w285:i32)
        n223 = local write "Valve open dur. (ms)"(w338) -> ()
        n224 = Reshape Array(w288, w287) -> (→"corridor lengths":i32[])
        n225 = Reshape Array(w282, w285) -> (→"teleports":i32[])
        n226 = Array Size(array=w277) -> (size(s)=w276:i32)
        n227 = Greater?(x=w276, y=w273) -> (0:w274:bool)
        n228 = Select(t=w273, s=w274, f=2) -> (s? t:f=w275:i32)
        n229 = property on="plot selector 2" class="Ring (strict)"("Value"=w275) -> ()  [unwired: 2 in, 2 out]
      }
      frame "Idle" {
        w397 = string[] []
        w422 = u16[] []
        w403 = u16 0 items=["none"] ("Stim. prot 1")
        w423 = u16[] []
        w461 = 1 ("length")
        # "Save reward calibration data"
        # "Select mouse from the current list of mice"
        n230 = local read "stim. num. 2"() -> (w429:u16)
        n231 = local read "stim. num. 3"() -> (w428:u16)
        n232 = local read "stim. num. 4"() -> (w427:u16)
        n233 = local read "stim. num. 5"() -> (w426:u16)
        n234 = stacked-sequence {
          seq-local: ["Stim protocols" _] -> [_ w533]
          seq-local: [w480 _] -> [_ w555]
          tunnel: [_ w531] -> w439
          frame #0 {
            n235 = call "Is Value Changed.vim"("value"="Stim protocols") -> ("changed or first call?"=w482:bool)
            n236 = local read "protocol array"() -> (w480:string[][])
            n237 = case shown="True" w482 {
              tunnel: w480 -> [_ w488]
              tunnel: "Stim protocols" -> [_ w486]
              frame False {
              }
              frame True {
                n238 = Index Array(array=w488, index (row)=w486, index (col)=2 ("disabled index (col)")) -> (element=w494:string)
                n239 = property on="Stim type" class="Ring (strict)"() -> ("StringsAndValues[]"=w497:T14)  [unwired: 2 in, 2 out]
                n240 = Index Array(array=w488, index (row)=w486, index (col)=0 ("disabled index (col)")) -> (element=w499:string)
                n241 = Index Array(array=w488, index (row)=w486, index (col)=1 ("disabled index (col)")) -> (element=w496:string)
                n242 = Index Array(array=w488, index (row)=w486, index (col)=4 ("disabled index (col)")) -> (element=w487:string)
                n243 = Index Array(array=w488, index (row)=w486, index (col)=3 ("disabled index (col)")) -> (element=w503:string)
                n244 = Match Pattern(string=w494, regular expression="to ") -> (after substring=w495:string)  [unwired: 1 in, 3 out]
                n245 = Match Pattern(string=w496, regular expression="from ") -> (after substring=w508:string)  [unwired: 1 in, 3 out]
                n246 = Not Equal?(x=w495, y="rew") -> ()  [unwired: 1 out]
                n247 = Match Pattern(string=w503, regular expression=" int. ") -> (after substring=w502:string)  [unwired: 1 in, 3 out]
                n248 = Not Equal?(x=w508, y="rew") -> ()  [unwired: 1 out]
                n249 = Match Pattern(string=w487, regular expression=" duty cycle. ") -> (after substring=w492:string)  [unwired: 1 in, 3 out]
                n250 = Match Pattern(string=w502, regular expression=" %  ") -> (before substring=w501:string)  [unwired: 1 in, 3 out]
                n251 = Match Pattern(string=w492, regular expression=" %  ") -> (before substring=w493:string)  [unwired: 1 in, 3 out]
                n252 = Decimal String To Number(string=w508) -> (number=w484:i32)  [unwired: 2 in, 1 out]
                n253 = Decimal String To Number(string=w495) -> (number=w483:i32)  [unwired: 2 in, 1 out]
                n254 = Array Size(array=w497) -> (size(s)=w500:i32)
                n255 = for {
                  N: w500 -> [_]
                  tunnel: w499 -> [w517]
                  tunnel: w497 -> [w516] mode=indexing
                  n256 = Unbundle(w516) -> ("String"=w515:string, "Value"=w519:u16)
                  n257 = Equal?(x=w517, y=w515) -> (x = y?=w518:bool)
                  n258 = case shown="True" w518 {
                    tunnel: w519 -> [_ w520]
                    frame False {
                    }
                    frame True {
                      n259 = local write "Stim type"(w520) -> ()
                    }
                  }
                }
                n260 = Decimal String To Number(string=w493) -> (number=w485:i32)  [unwired: 2 in, 1 out]
                n261 = Decimal String To Number(string=w501) -> (number=w498:i32)  [unwired: 2 in, 1 out]
                n262 = local write "Intensity (%)"(w498) -> ()
                n263 = local write "Duty cycle (%)"(w485) -> ()
                n264 = local write "start (cm)"(w484) -> ()
                n265 = local write "stop (cm)"(w483) -> ()
              }
            }
          }
          frame #1 {
            w528 = "" ("new element/subarray")
            w530 = 0 ("index (row)")
            n266 = Number To Decimal String(number="stop (cm)") -> (decimal integer string=w526:string)  [unwired: 1 in]
            n267 = Number To Decimal String(number="Duty cycle (%)") -> (decimal integer string=w539:string)  [unwired: 1 in]
            n268 = Number To Decimal String(number="Intensity (%)") -> (decimal integer string=w560:string)  [unwired: 1 in]
            n269 = Concatenate Strings(" to " ("string"), w526) -> (w569:string)
            n270 = property on="Stim type" class="Ring (strict)"() -> ("RingText.Text"=w542:string)  [unwired: 2 in, 2 out]
            n271 = Number To Decimal String(number="start (cm)") -> (decimal integer string=w522:string)  [unwired: 1 in]
            n272 = property on="stop (cm)" class="DigNum (strict)"("DisabledEnum"=T6."Enabled" ("Disabled")) -> ()  [unwired: 2 in, 2 out]
            n273 = property on="start (cm)" class="DigNum (strict)"("DisabledEnum"=T6."Enabled" ("Disabled")) -> ()  [unwired: 2 in, 2 out]
            n274 = Concatenate Strings(" from " ("string"), w522) -> (w568:string)
            n275 = Concatenate Strings(" int. " ("string"), w560, " %" ("string")) -> (w570:string)
            n276 = Concatenate Strings(" duty cycle " ("string"), w539, " %" ("string")) -> (w535:string)
            n277 = Not Equal?(x=w542, y="none") -> (x != y?=w543:bool)
            n278 = case shown="True" w543 {
              tunnel: w570 -> [w576 _]
              tunnel: w569 -> [w575 _]
              tunnel: w568 -> [w574 _]
              tunnel: [w573 w579] -> w564
              tunnel: w542 -> [w572 w578]
              tunnel: w535 -> [w571 _]
              frame True {
                n279 = Build Array(w572, w574, w575, w576, w571) -> (w573:string[])
              }
              frame False {
                w577 = "" ("element")
                n280 = Build Array(w578, w577, w577, w577, w577) -> (w579:string[])
              }
            }
            n281 = Replace Array Subset(array=w555, new element=w542, index (row)=w533, index (col)=0 ("disabled index (col)")) -> (w565:string[][])
            n282 = Replace Array Subset(array=w565, new element=w568, index (row)=w533, index (col)=1 ("disabled index (col)")) -> (w566:string[][])
            n283 = Replace Array Subset(array=w566, new element=w569, index (row)=w533, index (col)=2 ("disabled index (col)")) -> (w567:string[][])
            n284 = Replace Array Subset(array=w567, new element=w570, index (row)=w533, index (col)=3 ("disabled index (col)")) -> (w534:string[][])
            n285 = Replace Array Subset(array=w534, new element=w535, index (row)=w533, index (col)=4 ("disabled index (col)")) -> (w536:string[][])
            n286 = Replace Array Subset(array=w536, new element="none" ("new element/subarray"), index (row)=w530, index (col)=0 ("disabled index (col)")) -> (w549:string[][])
            n287 = Replace Array Subset(array=w549, new element=w528, index (row)=w530, index (col)=1 ("disabled index (col)")) -> (w548:string[][])
            n288 = Replace Array Subset(array=w548, new element=w528, index (row)=w530, index (col)=2 ("disabled index (col)")) -> (w547:string[][])
            n289 = Replace Array Subset(array=w547, new element=w528, index (row)=w530, index (col)=3 ("disabled index (col)")) -> (w532:string[][])
            n290 = Replace Array Subset(array=w532, new element=w528, index (row)=w530, index (col)=4 ("disabled index (col)")) -> (w531:string[][])
            n291 = local write "protocol array"(w531) -> ()
            n292 = Concatenate Strings(w564) -> (w563:string)
            n293 = property on="Stim protocols" class="Ring (strict)"("RingText.Text"=w563) -> ()  [unwired: 2 in, 2 out]
          }
        }
        n294 = for {
          N: "Trial block" -> [_]
          shift-right: [w676] -> w441
          shift-left: i32[] [] -> [w675]
          i -> [w677]
          n295 = Insert Into Array(array=w675, index=w677, new element=w677) -> (w676:i32[])
        }
        n296 = Compound Arithmetic op=ADD(w429, w428, w427, w426) -> (w425:u16)
        n297 = Build Array(w403, "Stim. prot 2", "Stim. prot 3", "Stim. prot 4", "Stim. prot 5") -> (w398:u16[])
        n298 = for {
          N: "stim. num. 2" -> [_]
          tunnel: "Stim. prot 2" -> [w665]
          shift-right: [w664] -> w437
          shift-left: w423 -> [w663]
          i -> [w666]
          n299 = Insert Into Array(array=w663, index=w666, new element=w665) -> (w664:u16[])
        }
        n300 = for {
          N: "stim. num. 3" -> [_]
          tunnel: "Stim. prot 3" -> [w661]
          shift-right: [w660] -> w438
          shift-left: w423 -> [w659]
          i -> [w662]
          n301 = Insert Into Array(array=w659, index=w662, new element=w661) -> (w660:u16[])
        }
        n302 = for {
          N: "stim. num. 4" -> [_]
          tunnel: "Stim. prot 4" -> [w657]
          shift-right: [w656] -> w435
          shift-left: w423 -> [w655]
          i -> [w658]
          n303 = Insert Into Array(array=w655, index=w658, new element=w657) -> (w656:u16[])
        }
        n304 = for {
          N: "stim. num. 5" -> [_]
          tunnel: "Stim. prot 5" -> [w653]
          shift-right: [w652] -> w434
          shift-left: w423 -> [w651]
          i -> [w654]
          n305 = Insert Into Array(array=w651, index=w654, new element=w653) -> (w652:u16[])
        }
        n306 = Subtract(x="Trial block", y=w425) -> (x-y=w424:u16)
        "stim. num. 1" <- w424
        n307 = for {
          N: w424 -> [_]
          tunnel: w403 -> [w669]
          shift-right: [w668] -> w436
          shift-left: w423 -> [w667]
          i -> [w670]
          n308 = Insert Into Array(array=w667, index=w670, new element=w669) -> (w668:u16[])
        }
        n309 = local write "shuffled array"(w441) -> ()
        n310 = Build Array (concatenate)(w436, w437, w438, w435, w434) -> (→"Stim types":u16[])
        n311 = Build Array("Block 1", "Block 2", "Block 3", "Block 4", "Block 5") -> (w385:u16[])
        n312 = local read "Block num. 1"() -> (w370:u16)
        n313 = local read "Block num. 2"() -> (w371:u16)
        n314 = local read "Block num. 3"() -> (w372:u16)
        n315 = local read "Block num. 4"() -> (w373:u16)
        n316 = local read "Block num. 5"() -> (w369:u16)
        n317 = for {
          N: "Block num. 1" -> [_]
          tunnel: "Block 1" -> [w649]
          shift-right: [w648] -> w416
          shift-left: w422 -> [w647]
          i -> [w650]
          n318 = Insert Into Array(array=w647, index=w650, new element=w649) -> (w648:u16[])
        }
        n319 = for {
          N: "Block num. 2" -> [_]
          tunnel: "Block 2" -> [w645]
          shift-right: [w644] -> w415
          shift-left: w422 -> [w643]
          i -> [w646]
          n320 = Insert Into Array(array=w643, index=w646, new element=w645) -> (w644:u16[])
        }
        n321 = for {
          N: "Block num. 3" -> [_]
          tunnel: "Block 3" -> [w641]
          shift-right: [w640] -> w414
          shift-left: w422 -> [w639]
          i -> [w642]
          n322 = Insert Into Array(array=w639, index=w642, new element=w641) -> (w640:u16[])
        }
        n323 = for {
          N: "Block num. 4" -> [_]
          tunnel: "Block 4" -> [w637]
          shift-right: [w636] -> w413
          shift-left: w422 -> [w635]
          i -> [w638]
          n324 = Insert Into Array(array=w635, index=w638, new element=w637) -> (w636:u16[])
        }
        n325 = for {
          N: "Block num. 5" -> [_]
          tunnel: "Block 5" -> [w633]
          shift-right: [w632] -> w412
          shift-left: w422 -> [w631]
          i -> [w634]
          n326 = Insert Into Array(array=w631, index=w634, new element=w633) -> (w632:u16[])
        }
        n327 = call "Is Value Changed.vim"("value"=w439) -> ("changed or first call?"=w440:bool)
        n328 = case shown="True" w440 {
          tunnel: w439 -> [_ w674]
          frame False {
          }
          frame True {
            n329 = local read "settings folder"() -> (w673:path)
            n330 = Build Path(base path=w673, name or relative path="Stimprotocols.txt") -> (appended path=w671:path)
            n331 = call-poly <vilib>:"Write Delimited Spreadsheet.vi"("file path (dialog if empty)"=w671, "2D data"=w674) -> ()  [unwired: 12 in, 2 out]
          }
        }
        n332 = Compound Arithmetic op=ADD(w370, w371, w372, w373, w369) -> (→"Session length":u16)
        n333 = Build Array (concatenate)(w416, w415, w414, w413, w412) -> (→"Context types":u16[])
        n334 = property on="Stim protocols" class="Ring (strict)"() -> ("Strings []"=w411:string[])  [unwired: 2 in, 2 out]
        n335 = property on="Stim. prot 1" class="Ring (strict)"("Strings []"=w411) -> ()  [unwired: 2 in, 2 out]
        n336 = property on="Stim. prot 2" class="Ring (strict)"("Strings []"=w411) -> ()  [unwired: 2 in, 2 out]
        n337 = property on="Stim. prot 3" class="Ring (strict)"("Strings []"=w411) -> ()  [unwired: 2 in, 2 out]
        n338 = property on="Stim. prot 4" class="Ring (strict)"("Strings []"=w411) -> ()  [unwired: 2 in, 2 out]
        n339 = property on="Stim. prot 5" class="Ring (strict)"("Strings []"=w411) -> ()  [unwired: 2 in, 2 out]
        n340 = local read "stim. num. 1"() -> (w408:u16)
        n341 = local read "stim. num. 2"() -> (w407:u16)
        n342 = local read "stim. num. 3"() -> (w406:u16)
        n343 = local read "stim. num. 4"() -> (w405:u16)
        n344 = local read "stim. num. 5"() -> (w404:u16)
        n345 = local read "Block num. 1"() -> (w395:u16)
        n346 = local read "Block num. 2"() -> (w394:u16)
        n347 = local read "Block num. 3"() -> (w393:u16)
        n348 = local read "Block num. 4"() -> (w392:u16)
        n349 = local read "Block num. 5"() -> (w391:u16)
        n350 = local read "Last saved reward size"() -> (w450:dbl)
        n351 = Build Array(w408, w407, w406, w405, w404) -> (w396:u16[])
        n352 = Build Array(w395, w394, w393, w392, w391) -> (w390:u16[])
        n353 = Array Size(array=w396) -> (size(s)=w410:i32)
        n354 = Not Equal?(x="Reward size (ul)", y=w450) -> (x != y?=w466:bool)
        n355 = for {
          N: w410 -> [_]
          tunnel: w385 -> [w594] mode=indexing
          shift-right: [w590] -> w382
          shift-left: w397 -> [w589]
          tunnel: w390 -> [w588] mode=indexing
          tunnel: w398 -> [w582] mode=indexing
          shift-right: [w586] -> w384
          shift-left: w397 -> [w581]
          tunnel: w396 -> [w587] mode=indexing
          i -> [w580]
          n356 = Greater?(x=w588, y=u16 0) -> (0:w593:bool)
          n357 = Greater?(x=w587, y=u16 0) -> (0:w583:bool)
          n358 = case shown="True" w593 {
            tunnel: w594 -> [_ w630]
            tunnel: w588 -> [_ w629]
            tunnel: ["" w618] -> w591
            frame False {
            }
            frame True {
              n359 = property on="Block 1" class="Ring (strict)"() -> ("StringsAndValues[]"=w613:T14)  [unwired: 2 in, 2 out]
              n360 = local read "Session length"() -> (w614:u16)
              n361 = Number To Decimal String(number=w629) -> (decimal integer string=w624:string)  [unwired: 1 in]
              n362 = Index Array(array=w613, index=w630) -> (element=w628:cluster{"String":string, "Value":u16})
              n363 = Number To Decimal String(number=w614) -> (decimal integer string=w622:string)  [unwired: 1 in]
              n364 = Concatenate Strings(w624, "/" ("string"), w622) -> (w621:string)
              n365 = Unbundle(w628) -> ("String"=w617:string, "Value"=w627:u16)
              n366 = Number To Decimal String(number=w627) -> (decimal integer string=w626:string)  [unwired: 1 in]
              n367 = Match Pattern(string=w617, regular expression="int. ") -> (before substring=w615:string)  [unwired: 1 in, 3 out]
              n368 = Concatenate Strings(w626, ": " ("string"), w621, " " ("string"), w615, "\n" ("string")) -> (w618:string)
            }
          }
          n369 = case shown="True" w583 {
            tunnel: w582 -> [_ w610]
            tunnel: w587 -> [_ w609]
            tunnel: ["" w596] -> w585
            frame False {
            }
            frame True {
              n370 = property on="Stim protocols" class="Ring (strict)"() -> ("StringsAndValues[]"=w611:T14)  [unwired: 2 in, 2 out]
              n371 = local read "Trial block"() -> (w602:u16)
              n372 = Number To Decimal String(number=w609) -> (decimal integer string=w604:string)  [unwired: 1 in]
              n373 = Index Array(array=w611, index=w610) -> (element=w608:cluster{"String":string, "Value":u16})
              n374 = Number To Decimal String(number=w602) -> (decimal integer string=w601:string)  [unwired: 1 in]
              n375 = Unbundle(w608) -> ("String"=w598:string, "Value"=w607:u16)
              n376 = Concatenate Strings(w604, "/" ("string"), w601) -> (w600:string)
              n377 = Number To Decimal String(number=w607) -> (decimal integer string=w606:string)  [unwired: 1 in]
              n378 = Concatenate Strings(w606, ": " ("string"), w600, " " ("string"), w598, "\n" ("string")) -> (w596:string)
            }
          }
          n379 = Insert Into Array(array=w589, index=w580, new element=w591) -> (w590:string[])
          n380 = Insert Into Array(array=w581, index=w580, new element=w585) -> (w586:string[])
        }
        n381 = case shown="True" w466 {
          tunnel: "Reward size (ul)" -> [_ w685]
          frame False {
          }
          frame True {
            n382 = local write "Last saved reward size"(w685) -> ()
            n383 = local read "settings folder"() -> (w684:path)
            n384 = local read "Valve open dur. (ms)"() -> (w693:u32)
            n385 = local read "Date"() -> (w688:string)
            n386 = Build Path(base path=w684, name or relative path="Last calibration.txt") -> (appended path=w682:path)
            n387 = Number To Decimal String(number=w693) -> (decimal integer string=w694:string)  [unwired: 1 in]
            n388 = Number To Fractional String(number=w685, precision (6)=i16 2) -> (F-format string=w696:string)  [unwired: 2 in]
            n389 = Concatenate Strings(w696, " ul / " ("string"), w694, " ms " ("string"), " (" ("string"), w688, ")" ("string")) -> (w690:string)
            "Last calibration" <- w690
            n390 = Open/Create/Replace File(file path (use dialog)=w682, operation (0:open)=T10."open") -> (refnum out=w697:refnum<file>)  [unwired: 4 in, 2 out]
            n391 = Write to Text File(file (use dialog)=w697, text=w690) -> (refnum out=w698:refnum<file>)  [unwired: 2 in, 2 out]
            n392 = Close File(refnum=w698) -> ()  [unwired: 1 in, 2 out]
          }
        }
        n393 = local write "Primary masking light"("Primary masking light") -> ()
        n394 = local read "Current mice"() -> (w464:string[][])
        n395 = local write "Run experiment"(FALSE ("Record")) -> ()
        n396 = Array Subset(array=w464, index (row)="Scrollbar", length (row)=w461, index (col)=0 ("index 2"), length (col)=w461) -> (w471:string[][])
        n397 = Array Subset(array=w464, index (row)="Scrollbar", length (row)=w461, index (col)=1 ("index 2"), length (col)=w461) -> (w468:string[][])
        n398 = Array Subset(array=w464, index (row)="Scrollbar", length (row)=w461, index (col)=2 ("index"), length (col)=w461) -> (w460:string[][])
        n399 = Concatenate Strings(w460) -> (w458:string)
        n400 = Format Date/Time String(time format string (%c)="%Y.%m.%d") -> (date/time string=→"Date":string)  [unwired: 2 in]
        n401 = Fract/Exp String To Number(string=w458) -> (number=w457:dbl)  [unwired: 3 in, 1 out]
        "Original weight" <- w457
        n402 = local read "Stim types"() -> (w367:u16[])
        n403 = Concatenate Strings(w471, string[][] [["-"]] ("string"), w468) -> (w448:string)
        "Mouse name" <- w448
        n404 = Divide(x="Weight", y=w457) -> (x/y=w455:dbl)
        n405 = case shown="True" "Edit mouse list" {
          frame False {
            n406 = property on="Current mice" class="Arr (strict)"("DisabledEnum"=T6."Disabled and Grayed Out" ("Disabled")) -> ()  [unwired: 2 in, 2 out]
          }
          frame True {
            n407 = local read "settings folder"() -> (w702:path)
            n408 = property on="Current mice" class="Arr (strict)"("DisabledEnum"=T6."Enabled" ("Disabled")) -> ()  [unwired: 2 in, 2 out]
            n409 = Build Path(base path=w702, name or relative path="List of mice.txt") -> (appended path=w700:path)
            n410 = call-poly <vilib>:"Write Delimited Spreadsheet.vi"("file path (dialog if empty)"=w700, "2D data"="Current mice") -> ()  [unwired: 12 in, 2 out]
          }
        }
        n411 = Add Array Elements(numeric array=w367) -> (sum=w366:u16)
        n412 = Concatenate Strings("\nOptical stimulation protocol:\n", w384, "\nVR context:\n", w382) -> (→"Stimulus protocol":string)
        n413 = Multiply(x=100.0, y=w455) -> (x*y=→"%":dbl)
        n414 = local read "Exit program"() -> (w478:bool)
        n415 = property on="Primary masking light" class="Enum (strict)"() -> ("RingText.Text"=w378:string)  [unwired: 2 in, 2 out]
        n416 = Greater?(x=w366, y=u16 0) -> (0:w364:bool)
        n417 = call "Is Value Changed.vim"("value"=w448) -> ("changed or first call?"=w447:bool)
        n418 = property on="plot selector bool 2" class="Bool (strict)"("Value"=w364) -> ()  [unwired: 2 in, 2 out]
        n419 = local write "Record"("Record Button") -> ()
        n420 = case shown="True" "Record Button" {
          frame False {
          }
          frame True {
            n421 = local read "Unique ID"() -> (w678:i8)
            n422 = Increment(x=w678) -> (x+1=w679:i8)
            n423 = local write "Unique ID"(w679) -> ()
          }
        }
        n424 = Or(x="Start recording", y="Record Button") -> (x .or. y?=w476:bool)
        n425 = case shown="True" w447 {
          frame False {
          }
          frame True {
            n426 = local write "Reset water count"(TRUE ("Reset water count")) -> ()
            n427 = local write "Unique ID"(i8 0 ("Unique ID")) -> ()
          }
        }
        n428 = case shown="False" w478 {
          frame False {
            n429 = flat-sequence {
              frame #0 {
                n430 = Wait (ms)(milliseconds to wait=u32 50) -> ()  [unwired: 1 out]
              }
              frame #1 {
                n431 = local write "Write"(TRUE ("Write")) -> ()
              }
            }
            n432 = local write "read"(FALSE ("read")) -> ()
          }
          frame True {
            n433 = stacked-sequence {
              frame #0 {
                n434 = local write "Encoder count"(100.0 ("Encoder count")) -> ()
                n435 = Wait (ms)(milliseconds to wait=u32 10) -> ()  [unwired: 1 out]
              }
              frame #1 {
                n436 = local write "Encoder count"(110.0 ("Encoder count")) -> ()
                n437 = Wait (ms)(milliseconds to wait=u32 10) -> ()  [unwired: 1 out]
              }
              frame #2 {
                n438 = local write "read"(FALSE ("read")) -> ()
                n439 = local write "Stop Unity"(TRUE ("Exit")) -> ()
              }
            }
            n440 = local read "Write loop stopped"() -> (w708:bool)
            n441 = case shown="True" w708 {
              frame False {
              }
              frame True {
                n442 = local write "Exit program"(FALSE ("Exit program")) -> ()
                n443 = local write "Exit"(TRUE ("Exit")) -> ()
              }
            }
          }
        }
        n444 = local write "Valve open dur. (ms)"("Valve open dur. (ms)") -> ()
        n445 = Concatenate Strings("Primary masking light: ", w378) -> (→"Masking light prot":string)
        n446 = local write "Comment"("Comment") -> ()
        n447 = local write "2P imaging"("2P imaging: NO" ("2P imaging")) -> ()
        n448 = local write "msg tag"("str," ("msg tag")) -> ()
        n449 = Select(t=T11."Init recording " ("main program"), s=w476, f=T11."Idle" ("main program")) -> (s? t:f=w475:T11)
        "Stim. prot 1" <- w403
      }
      frame "Init recording " {
        w749 = T6."Disabled" ("Disabled")
        w751 = 0 ("All trials")
        # "Reward zone available?"
        n450 = local read "teleports"() -> (w746:i16[])
        n451 = Index Array(array=w746, index=0) -> (element=w744:i16)
        n452 = local write "Edit mouse list"(FALSE ("Edit mouse list")) -> ()
        n453 = Decrement(x=w744) -> (x-1=w743:i16)
        n454 = local write "Run experiment"(TRUE ("record")) -> ()
        n455 = local write "Write"(TRUE ("Write")) -> ()
        n456 = local write "read"(TRUE ("read")) -> ()
        n457 = local write "Random reward"(FALSE ("Random reward")) -> ()
        n458 = local write "select trial"(FALSE ("Randomize")) -> ()
        n459 = local read "current VR context"() -> (w726:u16)
        n460 = local read "zeward zones"() -> (w727:i16[][])
        n461 = local write "Track position"(w743) -> ()
        n462 = Delete From Array(array=w727, index (row)=w726) -> (deleted portion=w728:i16[])  [unwired: 2 in, 1 out]
        n463 = Decimate 1D Array(w728) -> (w725:i16[], w724:i16[])
        n464 = disable-structure shown="Enabled" {
          disable-tunnel: [w775 -1 ("All trials")] -> w747
          frame Disabled {
            n465 = local read "VR Mode"() -> (w776:bool)
            n466 = Select(t=-1 ("All trials"), s=w776, f=0 ("All trials")) -> (s? t:f=w775:i32)
          }
          frame Enabled {
          }
        }
        n467 = Add Array Elements(numeric array=w725) -> (sum=w723:i16)
        n468 = Add Array Elements(numeric array=w724) -> (sum=w722:i16)
        n469 = Less?(x=w723, y=w722) -> (x < y?=w718:bool)
        n470 = local read "Context types"() -> (w741:u16[])
        n471 = Select(t=TRUE ("Hybrid licking"), s=w718, f=FALSE ("Active licking")) -> (s? t:f=w719:bool)
        n472 = local write "Stim prot command"(u16 0 ("Mask prot command")) -> ()
        n473 = local write "Trials in session array"(u16[][] [] ("Trials in session array")) -> ()
        n474 = local write "Prev. rew. pos."(0.0 ("Prev. rew. pos.")) -> ()
        n475 = local write "miss trial"(FALSE ("miss trial")) -> ()
        n476 = local write "Water count"(0 ("Water count")) -> ()
        n477 = local write "Active licking"(w719) -> ()
        n478 = local write "Start light stim"(FALSE ("Start light stim")) -> ()
        n479 = local write "Reward given"(u32 10 ("Reward given")) -> ()
        n480 = local write "Hybrid licking"(w719) -> ()
        n481 = local write "Reward zone"(TRUE ("Reward zone")) -> ()
        n482 = local write "Hit trials ctrl."(w751) -> ()
        n483 = local write "Hit trials"(w751) -> ()
        n484 = local write "Hit trials stim."(w751) -> ()
        n485 = local write "Ctrl. count"(w751) -> ()
        n486 = local write "Stim. count"(w751) -> ()
        n487 = Index Array(array=w741, index=0) -> (element=w735:u16)
        n488 = local write "All trials"(w747) -> ()
        n489 = local write "Context command"(w735) -> ()
        n490 = Increment(x=w735) -> (x+1=w740:u16)
        n491 = local read "corridor lengths"() -> (w733:i32[])
        n492 = Number To Decimal String(number=w740) -> (decimal integer string=w738:string)  [unwired: 1 in]
        n493 = local read "teleports"() -> (w734:i16[])
        n494 = Concatenate Strings("c" ("string"), w738) -> (w739:string)
        n495 = local write "Trial counted"(FALSE ("Trial counted")) -> ()
        n496 = local write "msg tag"(w739) -> ()
        n497 = disable-structure shown="Disabled" {
          frame Disabled {
            n498 = local read "Stim types"() -> (w786:u16[])
            n499 = local read item#-1() -> ()  [unwired: 1 out]
            n500 = Index Array(array=w786, index=1 ("index (row)")) -> (element=w788:u16)
            n501 = Add Array Elements(numeric array=w788) -> (sum=w787:dbl)
            n502 = Greater?(x=w787, y=i16 0) -> (0:w780:bool)
            n503 = Equal?(y=T12."None" ("Stimulus protocol")) -> (x = y?=w781:bool)  [unwired: 1 in]
            n504 = And(x=w780, y=w781) -> (x .and. y?=w782:bool)
            n505 = case shown="True" w782 {
              frame False {
              }
              frame True {
                n506 = One Button Dialog(message="No stimulus protocol has been selected!") -> ()  [unwired: 1 in, 1 out]
              }
            }
          }
          frame Enabled {
          }
        }
        n507 = Index Array(array=w734, index=w735) -> (element=w732:i16)
        n508 = Index Array(array=w733, index=w735) -> (element=w731:i32)
        n509 = Subtract(x=w732, y=w731) -> (x-y=w730:i32)
        n510 = local read "SciScan start"() -> (w760:refnum<k21>)
        n511 = property on="Top Graph" class="XYGraph (strict)"("XScale.Maximum"=w732, "XScale.Minimum"=w730) -> ()  [unwired: 2 in, 2 out]
        n512 = property on="Bottom Graph" class="XYGraph (strict)"("XScale.Maximum"=w732, "XScale.Minimum"=w730) -> ()  [unwired: 2 in, 2 out]
        n513 = property on="Position bar" class="Slide (strict)"("Scale.Maximum"=w732, "Scale.Minimum"=w730) -> ()  [unwired: 2 in, 2 out]
        n514 = call <vilib>:"DAQmx Start Task.vi"("task/channels in"=w760) -> ("task out"=w761:refnum<k21>, "error out"=w758:errorcluster)  [unwired: 13 in]
        n515 = local write "offset tag"("0," ("offset tag")) -> ()
        n516 = call-poly <vilib>:"DAQmx Write.vi"("task/channels in"=w761, "data"=FALSE, "error in"=w758) -> ("task out"=w757:refnum<k21>)  [unwired: 10 in, 2 out]
        n517 = disable-structure shown="Disabled" {
          frame Disabled {
            n518 = call <vilib>:"DAQmx Stop Task.vi"() -> ()  [unwired: 14 in, 2 out]
          }
          frame Enabled {
          }
        }
        n519 = property on="Record Button" class="Bool (strict)"("DisabledEnum"=w749) -> ()  [unwired: 2 in, 2 out]
        n520 = property on="Stop recording" class="Bool (strict)"("DisabledEnum"=T6."Enabled" ("Disabled")) -> ()  [unwired: 2 in, 2 out]
        n521 = local write "SciScan start"(w757) -> ()
        n522 = property on="Start recording" class="Bool (strict)"("DisabledEnum"=w749) -> ()  [unwired: 2 in, 2 out]
        n523 = disable-structure shown="Enabled" {
          disable-tunnel: [w778 TRUE ("VR Mode")] -> w764
          frame Disabled {
            n524 = local read "VR Mode"() -> (w778:bool)
          }
          frame Enabled {
          }
        }
        n525 = Select(t=T11."Record VR" ("main program"), s=w764, f=T11."Record" ("main program")) -> (s? t:f=w766:T11)
      }
      frame "Stop Recording" {
        w796 = T6."Enabled" ("Disabled")
        n526 = local read "VR Mode"() -> (w801:bool)
        n527 = local write "Run experiment"(FALSE ("Record")) -> ()
        n528 = local write "Start light stim"(FALSE ("Start light stim")) -> ()
        n529 = local write "Timed reward (s)"(u32 0 ("Timed reward (s)")) -> ()
        n530 = local write "Start recording"(FALSE ("Start recording")) -> ()
        n531 = local write "Record Button"(FALSE ("Record Button")) -> ()
        n532 = local write "Repetition"(1 ("Repetition")) -> ()
        n533 = case shown="True" w801 {
          frame False {
          }
          frame True {
            # "Wait for writing stimulus protocol, etc. to in lab book file"
            n534 = flat-sequence {
              frame #0 {
                n535 = Wait (ms)(milliseconds to wait=u32 100) -> ()  [unwired: 1 out]
              }
              frame #1 {
                n536 = local write "Primary masking light"(T13."None" ("Masking light")) -> ()
              }
            }
          }
        }
        n537 = local read "Extra stop triggers"() -> (w790:bool)
        n538 = local read "SciScan start"() -> (w792:refnum<k21>)
        n539 = case shown="True" w790 {
          tunnel: w792 -> [w808 w815]
          tunnel: [w807 w810] -> w793
          frame False {
            n540 = call-poly <vilib>:"DAQmx Write.vi"("task/channels in"=w808, "data"=FALSE) -> ("task out"=w807:refnum<k21>)  [unwired: 11 in, 2 out]
          }
          frame True {
            n541 = flat-sequence {
              tunnel: w815 -> [w817]
              tunnel: [w816] -> w814
              tunnel: w814 -> [w821]
              tunnel: [w820] -> w813
              tunnel: w813 -> [w825]
              tunnel: [w824] -> w812
              tunnel: w812 -> [w829]
              tunnel: [w828] -> w811
              tunnel: w811 -> [w834]
              tunnel: [w833] -> w810
              frame #0 {
                n542 = call-poly <vilib>:"DAQmx Write.vi"("task/channels in"=w817, "data"=FALSE) -> ("task out"=w816:refnum<k21>)  [unwired: 11 in, 2 out]
                n543 = Wait (ms)(milliseconds to wait=u32 20) -> ()  [unwired: 1 out]
              }
              frame #1 {
                n544 = call-poly <vilib>:"DAQmx Write.vi"("task/channels in"=w821, "data"=TRUE) -> ("task out"=w820:refnum<k21>)  [unwired: 11 in, 2 out]
                n545 = Wait (ms)(milliseconds to wait=u32 20) -> ()  [unwired: 1 out]
              }
              frame #2 {
                n546 = call-poly <vilib>:"DAQmx Write.vi"("task/channels in"=w825, "data"=FALSE) -> ("task out"=w824:refnum<k21>)  [unwired: 11 in, 2 out]
                n547 = Wait (ms)(milliseconds to wait=u32 50) -> ()  [unwired: 1 out]
              }
              frame #3 {
                n548 = call-poly <vilib>:"DAQmx Write.vi"("task/channels in"=w829, "data"=TRUE) -> ("task out"=w828:refnum<k21>)  [unwired: 11 in, 2 out]
                n549 = Wait (ms)(milliseconds to wait=u32 50) -> ()  [unwired: 1 out]
              }
              frame #4 {
                n550 = call-poly <vilib>:"DAQmx Write.vi"("task/channels in"=w834, "data"=FALSE) -> ("task out"=w833:refnum<k21>)  [unwired: 11 in, 2 out]
                n551 = Wait (ms)(milliseconds to wait=u32 10) -> ()  [unwired: 1 out]
              }
            }
          }
        }
        n552 = local write "Frame signal indicator"(FALSE ("Frame signal")) -> ()
        n553 = local write "SciScan"(FALSE ("SciScan")) -> ()
        n554 = Wait (ms)(milliseconds to wait=u32 100) -> ()  [unwired: 1 out]
        n555 = call <vilib>:"DAQmx Stop Task.vi"("task/channels in"=w793) -> ("task out"=w791:refnum<k21>)  [unwired: 13 in, 1 out]
        n556 = local write "SciScan start"(w791) -> ()
        n557 = property on="Stop recording" class="Bool (strict)"("DisabledEnum"=T6."Disabled" ("Disabled")) -> ()  [unwired: 2 in, 2 out]
        n558 = property on="Record Button" class="Bool (strict)"("DisabledEnum"=w796) -> ()  [unwired: 2 in, 2 out]
        n559 = property on="Start recording" class="Bool (strict)"("DisabledEnum"=w796) -> ()  [unwired: 2 in, 2 out]
      }
      frame "Exit program" {
      }
      frame "Record" {
        # "only true if prev. diode pos. <15 cm and reward given changes"
        # "These events happen only once in a trial at the beginning: 10 cm after the diode signal \nand  min ~ 5cm after revard given"
        # "Calculate \"Hit trials\""
        # "These events happen only once in a trial at the second half: 100 cm after diode signal"
        n560 = local read "Reward given"() -> (w840:u32)
        n561 = local read "VR Mode"() -> (w853:bool)
        n562 = local read "prev. diode position"() -> (w845:dbl)
        n563 = case shown="False" w853 {
          tunnel: [w883 w884] -> w852
          frame True {
            n564 = local read "Prev. rew. pos."() -> (w883:dbl)
          }
          frame False {
            n565 = local read "prev. diode position"() -> (w884:dbl)
          }
        }
        n566 = local read "prev. diode position"() -> (w860:dbl)
        n567 = Not Equal?(x=w840, y=u32 0) -> (x != y?=w839:bool)
        n568 = local read "total distance cm"() -> (w863:sgl[])
        n569 = local read "Trial counted"() -> (w851:bool)
        n570 = First Call?() -> (First Call?: T/F=w846:bool)
        n571 = local read "hit trial"() -> (w850:bool)
        n572 = Not(x=w846) -> (.not. x?=w843:bool)
        n573 = Greater?(x=w845, y=0.0) -> (0:w842:bool)
        n574 = Not(x=w851) -> (.not. x?=w848:bool)
        n575 = Array Max & Min(array=w863) -> (max value=w864:sgl)  [unwired: 3 out]
        n576 = call "Is Value Changed.vim"("value"=w852) -> ("changed or first call?"=w847:bool)
        n577 = call "Is Value Changed.vim"("value"=w839) -> ("changed or first call?"=w858:bool)
        n578 = Subtract(x=w864, y=w860) -> (x-y=w861:dbl)
        n579 = Compound Arithmetic op=AND(w847, w848, w843, w842) -> (w849:bool)
        n580 = Less?(x=w861, y=15.0) -> (x < y?=w859:bool)
        n581 = case shown="True" w849 {
          frame False {
          }
          frame True {
            n582 = stacked-sequence {
              frame #0 {
                n583 = local read "Reward given"() -> (w887:u32)
                n584 = Not Equal?(x=w887, y=u32 0) -> (x != y?=w885:bool)
                n585 = local read "Stim trial"() -> (w888:bool)
                n586 = local read "Stim trial"() -> (w890:bool)
                n587 = local read "Stim trial"() -> (w893:bool)
                n588 = local read "hit trial"() -> (w895:bool)
                n589 = local read "hit trial"() -> (w891:bool)
                n590 = case shown="True" w888 {
                  frame False {
                    n591 = local read "Ctrl. count"() -> (w898:i32)
                    n592 = Increment(x=w898) -> (x+1=w899:i32)
                    n593 = local write "Ctrl. count"(w899) -> ()
                  }
                  frame True {
                    n594 = local read "Stim. count"() -> (w901:i32)
                    n595 = Increment(x=w901) -> (x+1=w900:i32)
                    n596 = local write "Stim. count"(w900) -> ()
                  }
                }
                n597 = local read "All trials"() -> (w897:i32)
                n598 = Not(x=w890) -> (.not. x?=w889:bool)
                n599 = Compound Arithmetic op=AND(w885, w895, w889) -> (w894:bool)
                n600 = Compound Arithmetic op=AND(w885, w891, w893) -> (w892:bool)
                n601 = Increment(x=w897) -> (x+1=w896:i32)
                n602 = case shown="True" w894 {
                  frame False {
                  }
                  frame True {
                    n603 = local read "Hit trials ctrl."() -> (w904:i32)
                    n604 = Increment(x=w904) -> (x+1=w905:i32)
                    n605 = local write "Hit trials ctrl."(w905) -> ()
                  }
                }
                n606 = case shown="True" w892 {
                  frame False {
                  }
                  frame True {
                    n607 = local read "Hit trials stim."() -> (w902:i32)
                    n608 = Increment(x=w902) -> (x+1=w903:i32)
                    n609 = local write "Hit trials stim."(w903) -> ()
                  }
                }
                n610 = local write "All trials"(w896) -> ()
              }
              frame #1 {
                w936 = TRUE ("Trial counted")
                # "Build trial type array counting trials \nat the beginning"
                n611 = local read "Trial block"() -> (w906:u16)
                n612 = local read "All trials"() -> (w910:i32)
                n613 = local read "shuffled array"() -> (w913:i16[])
                n614 = local read "Trial block"() -> (w918:u16)
                n615 = local read "Stim types"() -> (w926:u16[])
                n616 = local read "All trials"() -> (w907:i32)
                n617 = local write "Trial counted"(w936) -> ()
                n618 = local write "select trial"(w936) -> ()
                n619 = Quotient & Remainder(x=w910, y=w918) -> (x-y*floor(x/y)=w915:i32)  [unwired: 1 out]
                n620 = Decrement(x=w918) -> (x-1=w914:u16)
                n621 = Increment(x=w907) -> (x+1=w911:i32)
                n622 = Quotient & Remainder(x=w907, y=w906) -> (x-y*floor(x/y)=w909:i32)  [unwired: 1 out]
                n623 = Quotient & Remainder(x=w911, y=w906) -> (x-y*floor(x/y)=w908:i32)  [unwired: 1 out]
                n624 = Equal?(x=w915, y=w914) -> (x = y?=w916:bool)
                n625 = Index Array(array=w913, index=w909) -> (element=w921:i16)
                n626 = call "Shuffle 1D Array.vim"("array"=w913) -> ("shuffled array"=w917:i16[])  [unwired: 4 in]
                n627 = Select(t=w917, s=w916, f=w913) -> (s? t:f=w912:i16[])
                n628 = Index Array(array=w912, index=w908) -> (element=w920:i16)
                n629 = Index Array(array=w926, index=w921) -> (element=w919:u16)
                n630 = Index Array(array=w926, index=w920) -> (element=w925:u16)
                n631 = local write "shuffled array"(w912) -> ()
                n632 = local write "Stim prot command"(w919) -> ()
                n633 = Build Array(w919, w919) -> (w933:u16[])
                n634 = property on="Stim protocols" class="Ring (strict)"() -> ("Strings []"=w932:string[])  [unwired: 2 in, 2 out]
                n635 = local read "Trials in session array"() -> (w934:u16[][])
                n636 = Greater?(x=w919, y=i8 0) -> (0:w929:bool)
                n637 = Select(t=TRUE, s=w929, f=FALSE) -> (s? t:f=w928:bool)
                n638 = local read "All trials"() -> (w927:i32)
                n639 = Index Array(array=w932, index=w919) -> (element=w931:string)
                n640 = Index Array(array=w932, index=w925) -> (element=w930:string)
                n641 = local write "Stim trial"(w928) -> ()
                n642 = local write "Current stim. protocol"(w931) -> ()
                n643 = local write "Next trial stim. protocol"(w930) -> ()
                n644 = Insert Into Array(array=w934, index (row)=w927, new element=w933) -> (w935:u16[][])  [unwired: 1 in]
                n645 = local write "Trials in session array"(w935) -> ()
              }
            }
          }
        }
        n646 = Compound Arithmetic op=AND(w858, w850, w859) -> (w857:bool)
        n647 = case shown="True" w857 {
          frame False {
          }
          frame True {
            n648 = local read "Hit trials"() -> (w944:i32)
            n649 = Increment(x=w944) -> (x+1=w943:i32)
            n650 = local write "Hit trials"(w943) -> ()
          }
        }
        n651 = local read "VR Mode"() -> (w856:bool)
        n652 = local read "total distance cm"() -> (w866:sgl[])
        n653 = case shown="False" w856 {
          tunnel: [140.0 ("y") w940] -> w855
          tunnel: [w937 w939] -> w854
          frame False {
            n654 = local read "prev. diode position"() -> (w937:dbl)
          }
          frame True {
            n655 = local read "Prev. rew. pos."() -> (w939:dbl)
            n656 = local read "Reward freq. (cm)"() -> (w942:u32)
            n657 = Subtract(x=w942, y=15.0) -> (x-y=w940:dbl)
          }
        }
        n658 = local read "Trial counted"() -> (w874:bool)
        n659 = Array Max & Min(array=w866) -> (max value=w865:sgl)  [unwired: 3 out]
        n660 = Subtract(x=w865, y=w854) -> (x-y=w875:dbl)
        n661 = Greater?(x=w875, y=w855) -> (0:w873:bool)
        n662 = And(x=w873, y=w874) -> (x .and. y?=w872:bool)
        n663 = case shown="True" w872 {
          frame False {
          }
          frame True {
            n664 = local write "Trial counted"(FALSE ("Trial counted")) -> ()
          }
        }
        n665 = local read "SciScan"() -> (w876:bool)
        n666 = local read "Stop recording"() -> (w879:bool)
        n667 = case shown="True" w876 {
          frame False {
          }
          frame True {
            n668 = local read "SciScan start"() -> (w947:refnum<k21>)
            n669 = local write "2P imaging"("2P imaging: YES" ("2P imaging")) -> ()
            n670 = call-poly <vilib>:"DAQmx Write.vi"("task/channels in"=w947, "data"=TRUE) -> ()  [unwired: 11 in, 3 out]
          }
        }
        n671 = local read "Exit program"() -> (w880:bool)
        n672 = local read "Hit trials"() -> (w871:i32)
        n673 = local read "All trials"() -> (w870:i32)
        n674 = Divide(x=w871, y=w870) -> (x/y=w868:dbl)
        "P hit trials" <- w868
        n675 = Or(x=w879, y=w880) -> (x .or. y?=w877:bool)
        n676 = Multiply(x=w868, y=100.0) -> (x*y=→"Hit trials %":dbl)
        n677 = Select(t=T11."Stop Recording" ("main program"), s=w877, f=T11."Record" ("main program")) -> (s? t:f=w878:T11)
      }
      frame "Record VR" {
        # "These computations run only once in a trial at the very beginning"
        n678 = disable-structure shown="Disabled" {
          frame Disabled {
            n679 = local read "Trial block"() -> (w1030:u16)
            n680 = local read "All trials"() -> (w1032:i32)
            n681 = local read item#-1() -> (w1037)
            n682 = Quotient & Remainder(x=w1032, y=w1030) -> (x-y*floor(x/y)=w1033:i32)  [unwired: 1 out]
            n683 = Decrement(x=w1030) -> (x-1=w1031:u16)
            n684 = Equal?(x=w1033, y=w1031) -> (x = y?=w1034:bool)
            n685 = Equal?(x=w1033, y=0.0) -> (x = y?=w1036:bool)
            n686 = Compound Arithmetic op=AND(w1036, w1037) -> (w1035:bool)
            n687 = case shown="True" w1034 {
              frame False {
              }
              frame True {
              }
            }
            n688 = case shown="True" w1035 {
              frame False {
              }
              frame True {
                n689 = local read "shuffled array"() -> (w1040:i16[])
                n690 = call "Shuffle 1D Array.vim"("array"=w1040) -> ("shuffled array"=w1039:i16[])  [unwired: 4 in]
                n691 = local write "shuffled array"(w1039) -> ()
                n692 = local write item#-1(FALSE ("Shuffle")) -> ()
              }
            }
          }
          frame Enabled {
          }
        }
        n693 = local read "Context command"() -> (w963:u16)
        n694 = local read "corridor lengths"() -> (w965:i32[])
        n695 = local read "teleports"() -> (w966:i16[])
        n696 = Index Array(array=w966, index=w963) -> (element=w964:i16)
        n697 = Index Array(array=w965, index=w963) -> (element=w962:i32)
        n698 = Divide(x=w962, y=2) -> (x/y=w960:dbl)
        n699 = Subtract(x=w964, y=w960) -> (x-y=w959:dbl)
        n700 = disable-structure shown="Enabled" {
          disable-tunnel: [w979 w982] -> w967
          disable-tunnel: w959 -> [w975 _]
          frame Disabled {
            n701 = local read "Track position"() -> (w974:sgl)
            n702 = local read "Trial counted"() -> (w980:bool)
            n703 = Equal?(x=w980, y=FALSE) -> (x = y?=w977:bool)
            n704 = Less?(x=w974, y=w975) -> (x < y?=w978:bool)
            n705 = Compound Arithmetic op=AND(w977, w978) -> (w979:bool)
          }
          frame Enabled {
            n706 = local read "Track position"() -> (w981:sgl)
            n707 = call "Is New Trial - trial counting.vi"("Position data"=w981) -> ("Boolean"=w982:bool)  [unwired: 1 in]
          }
        }
        n708 = case shown="True" w967 {
          frame False {
          }
          frame True {
            n709 = stacked-sequence {
              frame #0 {
                # "Build Trials in session array counting trials \nat the beginning"
                n710 = local read "All trials"() -> (w1060:i32)
                n711 = local read "shuffled array"() -> (w1045:i16[])
                n712 = local read "Trial block"() -> (w1048:u16)
                n713 = local read "Stim types"() -> (w1071:u16[])
                n714 = local read "Trial block"() -> (w1051:u16)
                n715 = local read "Context types"() -> (w1058:u16[])
                n716 = local read "Session length"() -> (w1057:u16)
                n717 = local read "Shuffle stim trials"() -> (w1043:bool)
                n718 = Increment(x=w1060) -> (x+1=w1047:i32)
                n719 = Quotient & Remainder(x=w1047, y=w1048) -> (x-y*floor(x/y)=w1050:i32)  [unwired: 1 out]
                n720 = local write "All trials"(w1047) -> ()
                n721 = Decrement(x=w1048) -> (x-1=w1049:u16)
                n722 = Increment(x=w1047) -> (x+1=w1052:i32)
                n723 = Quotient & Remainder(x=w1047, y=w1051) -> (x-y*floor(x/y)=w1073:i32)  [unwired: 1 out]
                n724 = Increment(x=w1047) -> (x+1=w1059:i32)
                n725 = Quotient & Remainder(x=w1052, y=w1051) -> (x-y*floor(x/y)=w1053:i32)  [unwired: 1 out]
                n726 = Equal?(x=w1050, y=w1049) -> (x = y?=w1044:bool)
                n727 = Quotient & Remainder(x=w1059, y=w1057) -> (x-y*floor(x/y)=w1066:i32)  [unwired: 1 out]
                n728 = Quotient & Remainder(x=w1047, y=w1057) -> (x-y*floor(x/y)=w1056:i32)  [unwired: 1 out]
                n729 = And(x=w1044, y=w1043) -> (x .and. y?=w1042:bool)
                n730 = Index Array(array=w1045, index=w1073) -> (element=w1070:i16)
                n731 = case shown="True" w1042 {
                  tunnel: [w1083 w1085] -> w1046
                  tunnel: w1045 -> [w1083 w1084]
                  frame False {
                  }
                  frame True {
                    n732 = call "Shuffle 1D Array.vim"("array"=w1084) -> ("shuffled array"=w1085:i16[])  [unwired: 4 in]
                  }
                }
                n733 = Index Array(array=w1046, index=w1053) -> (element=w1069:i16)
                n734 = Index Array(array=w1071, index=w1070) -> (element=w1067:u16)
                n735 = Index Array(array=w1071, index=w1069) -> (element=w1072:u16)
                n736 = Index Array(array=w1058, index=w1066) -> (element=w1055:u16)
                n737 = Index Array(array=w1058, index=w1056) -> (element=w1054:u16)
                n738 = local read "Trials in session array"() -> (w1082:u16[][])
                n739 = Build Array(w1067, w1054) -> (w1068:u16[])
                n740 = local write "current VR context"(w1054) -> ()
                n741 = local write "shuffled array"(w1046) -> ()
                n742 = property on="Stim protocols" class="Ring (strict)"() -> ("Strings []"=w1081:string[])  [unwired: 2 in, 2 out]
                n743 = Increment(x=w1055) -> (x+1=w1062:u16)
                n744 = Greater?(x=w1067, y=u16 0) -> (0:w1078:bool)
                n745 = local write "Context command"(w1055) -> ()
                n746 = Number To Decimal String(number=w1062) -> (decimal integer string=w1065:string)  [unwired: 1 in]
                n747 = Index Array(array=w1081, index=w1067) -> (element=w1080:string)
                n748 = Index Array(array=w1081, index=w1072) -> (element=w1079:string)
                n749 = Select(t=TRUE, s=w1078, f=FALSE) -> (s? t:f=w1077:bool)
                n750 = local write "Stim prot command"(w1067) -> ()
                n751 = local write "Current stim. protocol"(w1080) -> ()
                n752 = local write "Next trial stim. protocol"(w1079) -> ()
                n753 = local write "Stim trial"(w1077) -> ()
                n754 = Concatenate Strings("c" ("string"), w1065) -> (w1064:string)
                n755 = Insert Into Array(array=w1082, index (row)=w1047, new element=w1068) -> (w1061:u16[][])  [unwired: 1 in]
                n756 = local write "msg tag"(w1064) -> ()
                n757 = local write "Trials in session array"(w1061) -> ()
              }
              frame #1 {
                w1089 = TRUE ("Trial counted")
                n758 = local read "Reward given"() -> (w1088:u32)
                n759 = local write "Trial counted"(w1089) -> ()
                n760 = local write "select trial"(w1089) -> ()
                n761 = Not Equal?(x=w1088, y=u32 0) -> (x != y?=w1086:bool)
                n762 = local read "Stim trial"() -> (w1090:bool)
                n763 = local read "Stim trial"() -> (w1092:bool)
                n764 = local read "Stim trial"() -> (w1095:bool)
                n765 = local read "hit trial"() -> (w1097:bool)
                n766 = local read "hit trial"() -> (w1093:bool)
                n767 = case shown="True" w1090 {
                  frame False {
                    n768 = local read "Ctrl. count"() -> (w1098:i32)
                    n769 = Increment(x=w1098) -> (x+1=w1099:i32)
                    n770 = local write "Ctrl. count"(w1099) -> ()
                  }
                  frame True {
                    n771 = local read "Stim. count"() -> (w1101:i32)
                    n772 = Increment(x=w1101) -> (x+1=w1100:i32)
                    n773 = local write "Stim. count"(w1100) -> ()
                  }
                }
                n774 = Not(x=w1092) -> (.not. x?=w1091:bool)
                n775 = Compound Arithmetic op=AND(w1086, w1097, w1091) -> (w1096:bool)
                n776 = Compound Arithmetic op=AND(w1086, w1093, w1095) -> (w1094:bool)
                n777 = case shown="True" w1096 {
                  frame False {
                  }
                  frame True {
                    n778 = local read "Hit trials ctrl."() -> (w1104:i32)
                    n779 = Increment(x=w1104) -> (x+1=w1105:i32)
                    n780 = local write "Hit trials ctrl."(w1105) -> ()
                  }
                }
                n781 = case shown="True" w1094 {
                  frame False {
                  }
                  frame True {
                    n782 = local read "Hit trials stim."() -> (w1102:i32)
                    n783 = Increment(x=w1102) -> (x+1=w1103:i32)
                    n784 = local write "Hit trials stim."(w1103) -> ()
                  }
                }
              }
            }
          }
        }
        n785 = disable-structure shown="Disabled" {
          disable-tunnel: w959 -> [w984 _]
          frame Disabled {
            # "These computations run only once in a trial when the mouse enters to the RZ"
            n786 = local read "Track position"() -> (w983:sgl)
            n787 = local read "select trial"() -> (w985:bool)
            n788 = Greater?(x=w983, y=w984) -> (0:w986:bool)
            n789 = Compound Arithmetic op=AND(w986, w985) -> (w987:bool)
            n790 = case shown="True" w987 {
              frame True {
                w988 = FALSE ("Randomize")
                n791 = disable-structure shown="Disabled" {
                  frame Disabled {
                    n792 = local read "shuffled array"() -> (w1024:i16[])
                    n793 = local read "Trial block"() -> (w1018:u16)
                    n794 = local read "Stim types"() -> (w1020:u16[])
                    n795 = local read "All trials"() -> (w1025:i32)
                    n796 = Quotient & Remainder(x=w1025, y=w1018) -> (x-y*floor(x/y)=w1023:i32)  [unwired: 1 out]
                    n797 = Index Array(array=w1024, index=w1023) -> (element=w1019:i16)
                    n798 = Index Array(array=w1020, index (row)=1, index (col)=w1019) -> (element=w1017:u16)
                    n799 = Index Array(array=w1020, index (row)=0, index (col)=w1019) -> (element=w1015:u16)
                    n800 = Greater?(x=w1015, y=u16 0) -> (0:w1016:bool)
                    n801 = local write "Stim prot command"(w1015) -> ()
                    n802 = Select(t=TRUE ("Beaconed"), s=w1016, f=FALSE) -> (s? t:f=w1011:bool)
                    n803 = local write item#-1(w1017) -> ()
                    n804 = local write "Stim trial"(w1011) -> ()
                  }
                  frame Enabled {
                  }
                }
                n805 = disable-structure shown="Disabled" {
                  frame Disabled {
                    n806 = local read "VR start pos"() -> (w989:T1)
                    n807 = case shown="\"Random of 2\"" w989 {
                      tunnel: [w992 "0," w1003] -> w990
                      frame "Random of 4", Default {
                        n808 = local write "Random start pos"(TRUE ("Random start pos")) -> ()
                        n809 = Build Array("0,", "2,", "4,", "6,") -> (w998:string[])
                        n810 = call "Shuffle 1D Array.vim"("array"=w998) -> ("shuffled array"=w999:string[])  [unwired: 4 in]
                        n811 = Index Array(array=w999, index=0) -> (element=w992:string)
                      }
                      frame "Non-random" {
                        n812 = local write "Random start pos"(TRUE ("Random start pos")) -> ()
                      }
                      frame "Random of 2" {
                        n813 = local write "Random start pos"(TRUE ("Random start pos")) -> ()
                        n814 = Build Array("0,", "6,", "0,", "6,") -> (w1006:string[])
                        n815 = call "Shuffle 1D Array.vim"("array"=w1006) -> ("shuffled array"=w1004:string[])  [unwired: 4 in]
                        n816 = Index Array(array=w1004, index=0) -> (element=w1003:string)
                      }
                    }
                    n817 = local write "offset tag"(w990) -> ()
                  }
                  frame Enabled {
                  }
                }
                n818 = local write "Trial counted"(w988) -> ()
                n819 = local write "select trial"(w988) -> ()
              }
              frame False {
              }
            }
          }
          frame Enabled {
          }
        }
        n820 = disable-structure shown="Disabled" {
          frame Disabled {
            # "Wait to make sure DAQ recording \nis started before saving images"
            n821 = while {
              stop <- w1027 stop-if-true
              n822 = Wait (ms)(milliseconds to wait=u32 10) -> ()  [unwired: 1 out]
              n823 = local read "Record loop state"() -> (w1029:T5)
              n824 = Equal?(x=w1029, y=Record_enum."Record VR" ("Record loop state")) -> (x = y?=w1027:bool)
            }
          }
          frame Enabled {
          }
        }
        n825 = local read "Record loop state"() -> (w957:T5)
        n826 = local read "SciScan"() -> (w955:bool)
        n827 = local read "Session length"() -> (w952:u16)
        n828 = Equal?(x=w957, y=Record_enum."Record VR" ("Record loop state")) -> (x = y?=w956:bool)
        n829 = local read "Auto stop recording"() -> (w951:bool)
        n830 = local read "All trials"() -> (w953:i32)
        n831 = And(x=w955, y=w956) -> (x .and. y?=w954:bool)
        n832 = case shown="True" w954 {
          frame False {
          }
          frame True {
            n833 = local read "SciScan start"() -> (w1107:refnum<k21>)
            n834 = local write "2P imaging"("2P imaging: YES" ("2P imaging")) -> ()
            n835 = call-poly <vilib>:"DAQmx Write.vi"("task/channels in"=w1107, "data"=TRUE) -> ()  [unwired: 11 in, 3 out]
          }
        }
        n836 = Equal?(x=w953, y=w952) -> (x = y?=w950:bool)
        n837 = local read "Stop recording"() -> (w968:bool)
        n838 = local read "Exit program"() -> (w969:bool)
        n839 = And(x=w951, y=w950) -> (x .and. y?=w949:bool)
        n840 = Compound Arithmetic op=OR(w949, w968, w969) -> (w972:bool)
        n841 = Select(t=T11."Stop Recording" ("main program"), s=w972, f=T11."Record VR" ("main program")) -> (s? t:f=w973:T11)
      }
    }
    n842 = Wait (ms)(milliseconds to wait=u32 3) -> ()  [unwired: 1 out]
    n843 = local read "Exit"() -> (w271:bool)
  }
  n844 = while {
    shift-right: [w1136] -> _
    shift-left: w108 -> [w1135]
    shift-right: [w1132] -> _
    shift-left: _ -> [w1129]
    shift-right: [w1123] -> _
    shift-left: _ -> [w1128]
    shift-right: [w1131] -> _
    shift-left: _ -> [w1125]
    shift-right: [w1130] -> _
    shift-left: _ -> [w1124]
    shift-right: [w1127] -> _
    shift-left: _ -> [w1126]
    shift-right: [w1122] -> _
    shift-left: _ -> [w1121]
    shift-right: [w1118] -> _
    shift-left: _ -> [w1120]
    shift-right: [w1117] -> _
    shift-left: _ -> [w1119]
    shift-right: [w1116] -> _
    shift-left: 0.0 -> [w1115]
    shift-right: [w1114] -> _
    shift-left: _ -> [w1112]
    shift-right: [w1113] -> _
    shift-left: _ -> [w1111]
    shift-right: [w1110] -> _
    shift-left: _ -> [w1109]
    stop <- w1133 stop-if-true
    n845 = case shown="\"Record VR\"" w1135 {
      selector: w1135 -> [w1229 _ w1312 w1343 w1590 w1667]
      tunnel: [w1225 w1275 w1313 Record_enum."Idle" ("Record enum") w1591 w1668] -> w1136
      tunnel: [FALSE ("Exit") FALSE ("Exit") w1311 FALSE ("Exit") FALSE ("Exit") FALSE ("Exit")] -> w1133
      tunnel: [w1176 w1284 w1310 refnum<k21> refnum ("task out") w1572 w1664] -> w1132
      tunnel: [w1174 w1283 w1309 w1332 w1571 w1663] -> w1123
      tunnel: [w1170 w1282 w1306 refnum<k21> refnum ("task out") w1565 w1660] -> w1131
      tunnel: [w1172 w1281 w1305 w1331 w1564 w1659] -> w1130
      tunnel: w1129 -> [w1177 _ w1310 w1335 w1579 w1664]
      tunnel: w1128 -> [w1175 _ w1309 w1336 w1578 w1663]
      tunnel: [w1223 dbl[] [] w1308 w1341 w1503 w1662] -> w1127
      tunnel: w1126 -> [w1223 _ w1308 w1341 w1514 w1662]
      tunnel: w1125 -> [w1171 _ w1306 w1338 w1574 w1660]
      tunnel: w1124 -> [w1173 _ w1305 w1337 w1573 w1659]
      tunnel: [w1222 w1280 w1307 w1340 w1525 w1661] -> w1122
      tunnel: w1121 -> [w1222 _ w1307 w1340 w1561 w1661]
      tunnel: w1120 -> [_ _ _ _ w1550 _]
      tunnel: w1119 -> [_ _ _ _ w1546 _]
      tunnel: [0.0 0.0 0.0 0.0 w1552 0.0] -> w1118
      tunnel: [0.0 0.0 0.0 0.0 w1551 0.0] -> w1117
      tunnel: [w1219 w1270 w1301 w1327 w1529 w1656] -> w1116
      tunnel: w1115 -> [w1219 w1270 w1301 w1327 _ w1656]
      tunnel: [w1168 w1260 w1300 refnum<k21> refnum ("task out") w1521 w1655] -> w1114
      tunnel: [w1166 w1259 w1299 w1322 w1526 w1654] -> w1113
      tunnel: w1112 -> [w1169 _ w1300 w1325 w1524 w1655]
      tunnel: w1111 -> [w1167 _ w1299 w1324 w1527 w1654]
      tunnel: [w1194 dbl[] [] ("data") w1298 w1317 w1479 w1653] -> w1110
      tunnel: w1109 -> [w1194 _ w1298 w1317 _ w1653]
      frame "Init recording" {
        w1153 = " Hz" ("string")
        w1156 = "\n" ("string")
        w1139 = "   " ("string")
        w1188 = "-" ("string")
        # "Create a \"header\" for the lab book file from those variables that do not change during the recording"
        n846 = local write "Record loop state"(w1229) -> ()
        n847 = local read "Weight"() -> (w1207:dbl)
        n848 = local read "%"() -> (w1205:dbl)
        n849 = local read "Original weight"() -> (w1209:dbl)
        n850 = Number To Fractional String(number=w1205, precision (6)=i16 2) -> (F-format string=w1206:string)  [unwired: 2 in]
        n851 = Number To Fractional String(number=w1207, precision (6)=i16 1) -> (F-format string=w1208:string)  [unwired: 2 in]
        n852 = local read "Last calibration"() -> (w1212:string)
        n853 = Number To Fractional String(number=w1209, precision (6)=i16 1) -> (F-format string=w1210:string)  [unwired: 2 in]
        n854 = Concatenate Strings("Weight: " ("string"), w1206, " %   ( " ("string"), w1208, " g ; weight before water restriction: " ("string"), w1210, " g)" ("string")) -> (w1197:string)
        n855 = local read "Sample rate"() -> (w1162:dbl)
        n856 = case shown="True" FALSE {
          tunnel: ["" w1234] -> w1189
          frame False {
          }
          frame True {
            n857 = disable-structure shown="Disabled" {
              disable-tunnel: [w1238 _] -> w1234
              frame Disabled {
                n858 = local read "VR Mode"() -> ()  [unwired: 1 out]
                n859 = local read "zeward zones"() -> ()  [unwired: 1 out]
                n860 = Number To Decimal String() -> (decimal integer string=w1237:string)  [unwired: 2 in]
                n861 = Concatenate Strings("-" ("string"), w1237, "cm" ("string")) -> (w1238:string)
              }
              frame Enabled {
              }
            }
          }
        }
        n862 = local read "Loop rate"() -> (w1161:dbl)
        n863 = Concatenate Strings("Last calibration of water valve: " ("string"), w1212) -> (w1195:string)
        n864 = Number To Decimal String(number=w1162) -> (decimal integer string=w1159:string)  [unwired: 1 in]
        n865 = Number To Decimal String(number=w1161) -> (decimal integer string=w1155:string)  [unwired: 1 in]
        n866 = local read "Software version"() -> (w1196:string)
        n867 = local read "Mouse name"() -> (w1138:string)
        n868 = local read "User profile"() -> (w1137:string)
        n869 = call <vilib>:"DAQmx Stop Task.vi"("task/channels in"=w1177, "error in"=w1175) -> ("task out"=w1183:refnum<k21>, "error out"=w1182:errorcluster)  [unwired: 12 in]
        n870 = Concatenate Strings("Sampling rate: " ("string"), w1159, w1153, " Loop rate: " ("string"), w1155, w1153) -> (w1158:string)
        n871 = Format Date/Time String(time format string (%c)="%Y%m%d") -> (date/time string=w1151:string)  [unwired: 2 in]
        n872 = Format Date/Time String(time format string (%c)="%Y.%m.%d %H:%M:%S") -> (date/time string=w1140:string)  [unwired: 2 in]
        n873 = call <vilib>:"DAQmx Start Task.vi"("task/channels in"=w1183, "error in"=w1182) -> ("task out"=w1176:refnum<k21>, "error out"=w1174:errorcluster)  [unwired: 12 in]
        n874 = Concatenate Strings(w1140, w1139, w1138, w1139, w1137, w1156, w1156, w1197, w1156, w1195, w1156, w1196, w1156, w1158, w1156, "\n******************************" ("string"), w1156, w1156) -> (w1214:string)
        n875 = local read "Mouse name"() -> (w1193:string)
        n876 = local read "Recording folder"() -> (w1147:path)
        n877 = local read "Unique ID"() -> (w1184:i8)
        n878 = call <vilib>:"DAQmx Stop Task.vi"("task/channels in"=w1171, "error in"=w1173) -> ("task out"=w1180:refnum<k21>, "error out"=w1181:errorcluster)  [unwired: 12 in]
        n879 = local write "Header"(w1214) -> ()
        n880 = local write "Lab book notes"(w1214) -> ()
        n881 = Format Date/Time String(time format string (%c)="%Y.%m.%d") -> (date/time string=w1143:string)  [unwired: 2 in]
        n882 = Format Into String(format string="%02d", w1184) -> (resulting string=w1185:string)  [unwired: 2 in, 1 out]
        n883 = call <vilib>:"DAQmx Start Task.vi"("task/channels in"=w1180, "error in"=w1181) -> ("task out"=w1170:refnum<k21>, "error out"=w1172:errorcluster)  [unwired: 12 in]
        n884 = local read "Comment"() -> (w1187:string)
        n885 = Match Pattern(string=w1193, regular expression="-") -> (before substring=w1191:string, after substring=w1190:string)  [unwired: 1 in, 2 out]
        n886 = Strip Path(path=w1147) -> (stripped path=w1146:path)  [unwired: 1 out]
        n887 = Build Path(base path=w1146, name or relative path="PupilData") -> (appended path=w1144:path)
        n888 = call <vilib>:"DAQmx Stop Task.vi"("task/channels in"=w1169, "error in"=w1167) -> ("task out"=w1179:refnum<k21>, "error out"=w1178:errorcluster)  [unwired: 12 in]
        n889 = Build Path(base path=w1147, name or relative path=w1143) -> (appended path=w1232:path)
        n890 = Build Path(base path=w1144, name or relative path=w1143) -> (appended path=w1142:path)
        n891 = Concatenate Strings(w1191, w1188, w1151, w1188, w1185, w1188, w1190, w1189, w1188, w1187) -> (w1149:string)
        n892 = call <vilib>:"DAQmx Start Task.vi"("task/channels in"=w1179, "error in"=w1178) -> ("task out"=w1168:refnum<k21>, "error out"=w1166:errorcluster)  [unwired: 12 in]
        n893 = call <vilib>:"Check if File or Folder Exists.vi"("path"=w1232) -> ("file or folder exists?"=w1231:bool, "dup path"=w1230:path)  [unwired: 8 in, 1 out]
        n894 = Format Date/Time String(time format string (%c)="Session start: %H:%M:%S\n") -> (date/time string=→"Session start:":string)  [unwired: 2 in]
        n895 = case shown="False" w1231 {
          tunnel: [w1247 w1249] -> w1148
          tunnel: w1230 -> [w1247 w1248]
          frame True {
          }
          frame False {
            n896 = Create Folder(path (use dialog)=w1248) -> (created path=w1249:path)  [unwired: 2 in, 2 out]
          }
        }
        n897 = local write "Pupil Exp day folder"(w1142) -> ()
        n898 = Concatenate Strings(w1149, ".tdms") -> (w1213:string)
        n899 = Concatenate Strings(w1149, ".txt" ("string")) -> (w1217:string)
        n900 = Build Path(base path=w1148, name or relative path=w1217) -> (appended path=w1215:path)
        n901 = Build Path(base path=w1148, name or relative path=w1213) -> (appended path=w1228:path)
        n902 = local write "Filename"(w1149) -> ()
        n903 = local write "Lab book file"(w1215) -> ()
        n904 = call <vilib>:"Check if File or Folder Exists.vi"("path"=w1228) -> ("file or folder exists?"=w1226:bool, "dup path"=w1227:path)  [unwired: 8 in, 1 out]
        n905 = Format Date/Time String() -> ()  [unwired: 3 in, 1 out]
        n906 = case shown="True" w1226 {
          tunnel: w1227 -> [w1243 _]
          tunnel: [Record_enum."Record VR" ("Record enum") Record_enum."Init recording" ("Record enum")] -> w1225
          frame False {
            n907 = TDMS Open(5:FALSE ("create index file? (T)"), 10:T15."create" ("operation (0:open)"), 11:w1243) -> (3:w1240:refnum<k34>)  [unwired: 4 in, 1 out]
            n908 = local write "My tdms file"(w1240) -> ()
          }
          frame True {
            n909 = local read "Unique ID"() -> (w1246:i8)
            n910 = Increment(x=w1246) -> (x+1=w1245:i8)
            n911 = local write "Unique ID"(w1245) -> ()
          }
        }
      }
      frame "Init data acquisition" {
        w1250 = 0 items=["one channel for each line", "one channel for all lines"] ("line grouping")
        w1256 = 10083 items=["Default"=-1, "RSE"=10083, "NRSE"=10078, "Differential"=10106, "Pseudodifferential"=12529] ("input terminal configuration")
        (unwired) tag "Dev1/ai2" ("physical channels")
        w1264 = 10123 items=["Finite Samples"=10178, "Continuous Samples"=10123, "Hardware Timed Single Point"=12522] ("sample mode")
        w1286 = 10123 items=["Finite Samples"=10178, "Continuous Samples"=10123, "Hardware Timed Single Point"=12522] ("sample mode")
        w1292 = 10123 items=["Finite Samples"=10178, "Continuous Samples"=10123, "Hardware Timed Single Point"=12522] ("sample mode")
        (unwired) tag "Dev1/port0/line6" ("lines")
        # "Extra Analog Input"
        # "Frame signal 2"
        # "Valve open"
        # "Frame signal"
        # "Encoder"
        # "Lickport"
        n912 = call "Encoder read task.vi"() -> ("error out"=w1291:errorcluster, "task out"=w1290:refnum<k21>)  [unwired: 10 in]
        n913 = local read "Sample rate"() -> (w1287:dbl)
        n914 = call <vilib>:"DAQmx Flatten Channel String.vi"("names in"=string[] ["Dev1/port0/line4", "Dev1/port0/line5", "Dev1/port0/line6", "Dev1/port0/line3"]) -> ("names out"=w1252:string)  [unwired: 13 in, 1 out]
        n915 = call <vilib>:"DAQmx Flatten Channel String.vi"("names in"=string[] ["Dev1/ai0", "Dev1/ai4", "Dev1/ai6", "Dev1/ai1", "Dev1/ai2", "Dev1/ai3"]) -> ("names out"=w1262:string)  [unwired: 13 in, 1 out]
        n916 = local read "Sample rate"() -> (w1294:dbl)
        n917 = local read "Sample rate"() -> (w1266:dbl)
        n918 = call-poly <vilib>:"DAQmx Create Virtual Channel.vi"("lines"=w1252, "line grouping"=w1250) -> ("task out"=w1293:refnum<k21>, "error out"=w1295:errorcluster)  [unwired: 12 in]
        n919 = call-poly <vilib>:"DAQmx Create Virtual Channel.vi"("maximum value"=10.0, "minimum value"=-10.0, "input terminal configuration"=w1256, "physical channels"=w1262) -> ("task out"=w1265:refnum<k21>, "error out"=w1267:errorcluster)  [unwired: 10 in]
        n920 = call-poly <vilib>:"DAQmx Timing.vi"("task/channels in"=w1290, "sample mode"=w1286, "rate"=w1287, "source"=tag "/Dev1/di/SampleClock", "error in"=w1291) -> ("task out"=w1288:refnum<k21>, "error out"=w1289:errorcluster)  [unwired: 9 in]
        n921 = call-poly <vilib>:"DAQmx Timing.vi"("task/channels in"=w1293, "sample mode"=w1292, "rate"=w1294, "source"=tag "OnboardClock", "error in"=w1295) -> ("task out"=w1296:refnum<k21>, "error out"=w1297:errorcluster)  [unwired: 9 in]
        n922 = call-poly <vilib>:"DAQmx Timing.vi"("task/channels in"=w1265, "sample mode"=w1264, "rate"=w1266, "source"=tag "/Dev1/di/SampleClock", "error in"=w1267) -> ("task out"=w1268:refnum<k21>, "error out"=w1269:errorcluster)  [unwired: 9 in]
        n923 = call <vilib>:"DAQmx Start Task.vi"("task/channels in"=w1288, "error in"=w1289) -> ("task out"=w1284:refnum<k21>, "error out"=w1283:errorcluster)  [unwired: 12 in]
        n924 = call <vilib>:"DAQmx Start Task.vi"("task/channels in"=w1296, "error in"=w1297) -> ("task out"=w1282:refnum<k21>, "error out"=w1281:errorcluster)  [unwired: 12 in]
        n925 = call <vilib>:"DAQmx Start Task.vi"("task/channels in"=w1268, "error in"=w1269) -> ("task out"=w1260:refnum<k21>, "error out"=w1259:errorcluster)  [unwired: 12 in]
        n926 = local write "prev. diode position"(-157.0 ("prev. diode position")) -> ()
        n927 = local write "Store prev encoder count"(w1270) -> ()
        n928 = local read "Record"() -> (w1278:bool)
        n929 = Tick Count (ms)() -> (millisecond timer value=w1280:u32)
        "Start time" <- w1280
        n930 = local write "index"(0 ("index")) -> ()
        n931 = Select(t=Record_enum."Init recording" ("Record enum"), s=w1278, f=Record_enum."Record VR" ("Record enum")) -> (s? t:f=w1275:T5)
      }
      frame "Idle" {
        n932 = local write "Record loop state"(w1312) -> ()
        n933 = Wait (ms)(milliseconds to wait=u32 20) -> ()  [unwired: 1 out]
        n934 = local read "Run experiment"() -> (w1316:bool)
        n935 = Select(t=Record_enum."Init data acquisition" ("Record enum"), s=w1316, f=Record_enum."Idle" ("Record enum")) -> (s? t:f=w1313:T5)
        n936 = local read "Exit"() -> (w1311:bool)
      }
      frame "Stop data acquision" {
        n937 = local write "Record loop state"(w1343) -> ()
        n938 = local read "Record"() -> (w1330:bool)
        n939 = call <vilib>:"DAQmx Stop Task.vi"("task/channels in"=w1338, "error in"=w1337) -> ("task out"=w1333:refnum<k21>, "error out"=w1339:errorcluster)  [unwired: 12 in]
        n940 = call <vilib>:"DAQmx Stop Task.vi"("task/channels in"=w1325, "error in"=w1324) -> ("task out"=w1323:refnum<k21>, "error out"=w1326:errorcluster)  [unwired: 12 in]
        n941 = call <vilib>:"DAQmx Stop Task.vi"("task/channels in"=w1335, "error in"=w1336) -> ("task out"=w1334:refnum<k21>, "error out"=w1321:errorcluster)  [unwired: 12 in]
        n942 = call <vilib>:"DAQmx Clear Task.vi"("task in"=w1333, "error in"=w1339) -> ("error out"=w1331:errorcluster)  [unwired: 13 in]
        n943 = call <vilib>:"DAQmx Clear Task.vi"("task in"=w1323, "error in"=w1326) -> ("error out"=w1322:errorcluster)  [unwired: 13 in]
        n944 = call <vilib>:"DAQmx Clear Task.vi"("task in"=w1334, "error in"=w1321) -> ("error out"=w1332:errorcluster)  [unwired: 13 in]
        n945 = case shown="True" w1330 {
          frame False {
            n946 = local write "Start recording"(FALSE ("Start recording")) -> ()
          }
          frame True {
            w1349 = "\n"
            # "Write labbook data"
            n947 = local read "VR Mode"() -> (w1347:bool)
            n948 = local write "VR Mode"(w1347) -> ()
            n949 = local read "My tdms file"() -> (w1390:refnum<k34>)
            n950 = local write "Record Button"(FALSE ("Record Button")) -> ()
            n951 = local read "Security camera"() -> (w1351:string)
            n952 = local write "Record"(FALSE ("Logg data")) -> ()
            n953 = local read "2P imaging"() -> (w1350:string)
            n954 = case shown="True" TRUE {
              tunnel: [w1418 w1460] -> w1357
              frame True {
                w1395 = "\n" ("string")
                w1409 = "\n" ("string")
                w1421 = " (" ("string")
                # "VR Variables"
                n955 = local read "Trials in session array"() -> (w1408:u16[][])
                n956 = local read "Stim types"() -> (w1398:u16[])
                n957 = Add Array Elements(numeric array=w1398) -> (sum=w1400:u16)
                n958 = Greater?(x=w1400, y=i16 0) -> (0:w1397:bool)
                n959 = Number To Decimal String(number=w1408) -> (decimal integer string=w1407:string[][])  [unwired: 1 in]
                n960 = case shown="True" w1397 {
                  tunnel: ["" ("Laser stimulus calibration") w1434] -> w1394
                  frame False {
                  }
                  frame True {
                    n961 = local read "Laser stimulus calibration"() -> (w1435:string)
                    n962 = Concatenate Strings("\n" ("string"), w1435) -> (w1434:string)
                  }
                }
                n963 = local read "Stimulus protocol"() -> (w1396:string)
                n964 = Index Array(array=w1407, index (col)=0 ("disabled index (col)")) -> (element=w1406:string[])  [unwired: 1 in]
                n965 = Index Array(array=w1407, index (col)=1 ("disabled index (col)")) -> (element=w1405:string[])  [unwired: 1 in]
                n966 = local read "Masking light prot"() -> (w1417:string)
                n967 = Concatenate Strings("Trial types (stimulus protocols):\n", w1406, "\nTrial types (VR contexts):\n", w1405) -> (w1393:string)
                n968 = Concatenate Strings(w1396, w1395, w1393, w1395) -> (w1392:string)
                n969 = Concatenate Strings(w1409, w1417, w1409, w1392, w1394) -> (w1416:string)
                n970 = local read "Control hit trials %"() -> (w1411:dbl)
                n971 = local read "Stim. hit trials %"() -> (w1410:dbl)
                n972 = local read "Ctrl. count"() -> (w1427:i32)
                n973 = local read "Stim. count"() -> (w1412:i32)
                n974 = local read "All trials"() -> (w1430:i32)
                n975 = Number To Decimal String(number=w1427) -> (decimal integer string=w1426:string)  [unwired: 1 in]
                n976 = Number To Decimal String(number=w1430) -> (decimal integer string=w1429:string)  [unwired: 1 in]
                n977 = Number To Fractional String(number=w1410, precision (6)=i16 2) -> (F-format string=w1420:string)  [unwired: 2 in]
                n978 = Number To Decimal String(number=w1412) -> (decimal integer string=w1422:string)  [unwired: 1 in]
                n979 = Number To Fractional String(number=w1411, precision (6)=i16 2) -> (F-format string=w1424:string)  [unwired: 2 in]
                n980 = Concatenate Strings("\nReward zone distance: " ("string"), "" ("string"), " cm " ("string"), "\nAll trials: " ("string"), w1429, "\nControl trials: " ("string"), w1426, w1421, w1424, " % hit)\nStimulated trials: " ("string"), w1422, w1421, w1420, " % hit)\n" ("string"), w1416) -> (w1418:string)
              }
              frame False {
                w1436 = "\n" ("string")
                n981 = local read "Stim types"() -> (w1440:u16[])
                n982 = Add Array Elements(numeric array=w1440) -> (sum=w1443:u16)
                n983 = Greater?(x=w1443, y=i16 0) -> (0:w1442:bool)
                n984 = case shown="True" w1442 {
                  tunnel: ["" ("Laser stimulus calibration") w1463] -> w1437
                  frame False {
                  }
                  frame True {
                    w1462 = "\n" ("string")
                    n985 = local read "Stimulus protocol"() -> (w1465:string)
                    n986 = local read "Laser stimulus calibration"() -> (w1464:string)
                    n987 = Concatenate Strings(w1465, w1462, w1464, w1462) -> (w1463:string)
                  }
                }
                n988 = local read "Reward zone"() -> (w1444:bool)
                n989 = local read "Masking light prot"() -> (w1441:string)
                n990 = case shown="True" w1444 {
                  tunnel: [w1467 w1470] -> w1445
                  frame True {
                    n991 = local read "VR Mode"() -> (w1466:bool)
                    n992 = case shown="False" w1466 {
                      tunnel: ["Reward zone starts at photo diode (0-6 cm)." ""] -> w1467
                      frame False {
                      }
                      frame True {
                      }
                    }
                  }
                  frame False {
                    n993 = local read "Reward freq. (cm)"() -> (w1473:u32)
                    n994 = Number To Fractional String(number=w1473, precision (6)=i16 0) -> (F-format string=w1471:string)  [unwired: 2 in]
                    n995 = Concatenate Strings("\nReward frequency (minimum): " ("string"), w1471) -> (w1470:string)
                  }
                }
                n996 = Concatenate Strings(w1436, w1441, w1436, w1437) -> (w1438:string)
                n997 = local read "Hit trials"() -> (w1455:i32)
                n998 = local read "All trials"() -> (w1454:i32)
                n999 = Divide(x=w1455, y=w1454) -> (x/y=w1453:dbl)
                n1000 = Number To Decimal String(number=w1454) -> (decimal integer string=w1458:string)  [unwired: 1 in]
                n1001 = Multiply(x=w1453, y=100.0) -> (x*y=w1450:dbl)
                n1002 = Number To Decimal String(number=w1455) -> (decimal integer string=w1456:string)  [unwired: 1 in]
                n1003 = Number To Fractional String(number=w1450, precision (6)=i16 2) -> (F-format string=w1448:string)  [unwired: 2 in]
                n1004 = Concatenate Strings(w1445, "\nAll trials: " ("string"), w1458, "\nHit trials: " ("string"), w1456, " (" ("string"), w1448, " % correct)" ("string")) -> (w1446:string)
                n1005 = Concatenate Strings(w1446, w1438) -> (w1460:string)
              }
            }
            n1006 = local read "Reward size (ul)"() -> (w1378:dbl)
            n1007 = TDMS Close(11:w1390) -> ()  [unwired: 1 in, 2 out]
            n1008 = local read "Water count"() -> (w1377:i32)
            n1009 = Concatenate Strings(w1349, w1351, w1349, w1350, w1349) -> (w1348:string)
            n1010 = Multiply(x=w1378, y=w1377) -> (x*y=w1376:dbl)
            n1011 = Number To Fractional String(number=w1376, precision (6)=i16 2) -> (F-format string=w1373:string)  [unwired: 2 in]
            n1012 = Concatenate Strings("\nWater received: " ("string"), w1373, " ul" ("string")) -> (w1358:string)
            n1013 = Format Date/Time String(time format string (%c)="Session stop: %H:%M:%S\n") -> (date/time string=w1353:string)  [unwired: 2 in]
            n1014 = local read "Distance (m)"() -> (w1364:dbl)
            n1015 = local read "Session start:"() -> (w1354:string)
            n1016 = local read "Time (min)"() -> (w1368:dbl)
            n1017 = Number To Fractional String(number=w1368, precision (6)=i16 2) -> (F-format string=w1369:string)  [unwired: 2 in]
            n1018 = local read "Laps"() -> (w1360:i32)
            n1019 = Number To Fractional String(number=w1364, precision (6)=i16 2) -> (F-format string=w1363:string)  [unwired: 2 in]
            n1020 = Number To Decimal String(number=w1360) -> (decimal integer string=w1359:string)  [unwired: 1 in]
            n1021 = Concatenate Strings(w1354, w1353, "Time: " ("string"), w1369, " minutes\n" ("string"), "Distance: " ("string"), w1363, " m\n" ("string"), "Laps completed: " ("string"), w1359, w1358, w1357, w1348, "******************************\n" ("string")) -> (w1356:string)
            n1022 = local read "Lab book notes"() -> (w1385:string)
            n1023 = local read "Lab book file"() -> (w1383:path)
            n1024 = local read "Header"() -> (w1386:string)
            n1025 = Match Pattern(string=w1385, regular expression="***\n") -> (after substring=w1387:string)  [unwired: 1 in, 3 out]
            n1026 = Open/Create/Replace File(file path (use dialog)=w1383, operation (0:open)=T10."create") -> (refnum out=w1384:refnum<file>)  [unwired: 4 in, 2 out]
            n1027 = Concatenate Strings(w1386, w1356, w1387) -> (w1388:string)
            n1028 = Write to Text File(file (use dialog)=w1384, text=w1388) -> (refnum out=w1382:refnum<file>)  [unwired: 2 in, 2 out]
            n1029 = Close File(refnum=w1382) -> ()  [unwired: 1 in, 2 out]
          }
        }
      }
      frame "Record VR" {
        # "Calculate Velocity (cm/s) with 50Hz sampling"
        n1030 = local read "VR Mode"() -> (w1497:bool)
        n1031 = local read "Record"() -> (w1563:bool)
        n1032 = case shown="True" w1563 {
          frame False {
          }
          frame True {
            n1033 = case shown="True" TRUE ("VR Mode") {
              frame True {
                n1034 = local read "Photodiode signal"() -> (w1631:sgl[])
                n1035 = local read "total distance cm"() -> (w1630:sgl[])
                n1036 = local read "Photo stimulus signal"() -> (w1629:sgl[])
                n1037 = local read "Track position"() -> (w1611:sgl)
                n1038 = local read "Valve signal"() -> (w1625:i8[])
                n1039 = local read "lick signal"() -> (w1624:i8[])
                n1040 = local read "Frame signal"() -> (w1623:i8[])
                n1041 = local read "Trials in session array"() -> (w1618:u16[][])
                n1042 = local read "All trials"() -> (w1610:i32)
                n1043 = local read "No. of smpl. per ch."() -> (w1619:i32)
                n1044 = local read "analog lick"() -> (w1614:sgl[])
                n1045 = local read "Eye cam frame signal"() -> (w1615:i8[])
                n1046 = local read "ML signal"() -> (w1616:sgl[])
                n1047 = local read "Frame signal 2"() -> (w1609:i8[])
                n1048 = local read "Analog 3"() -> (w1608:sgl[])
                n1049 = local read "Encoder signal"() -> (w1621:sgl[])
                n1050 = Index Array(array=w1618, index (row)=w1610, index (col)=1 ("disabled index (col)")) -> (element=w1612:u16)
                n1051 = Index Array(array=w1618, index (row)=w1610, index (col)=0 ("disabled index (col)")) -> (element=w1620:u16)
                n1052 = Initialize Array(w1612, w1619) -> (w1613:u16[])
                n1053 = Initialize Array(w1620, w1619) -> (w1622:u16[])
                n1054 = Initialize Array(w1611, w1619) -> (w1628:sgl[])
                n1055 = Build Array(w1621, w1631, w1630, w1629, w1628, w1625, w1624, w1623, w1622, w1613, w1614, w1615, w1616, w1609, w1608) -> (w1626:sgl[][])
                n1056 = local read "My tdms file"() -> (w1633:refnum<k34>)
                n1057 = TDMS Write(0:w1633, 1:enum16{"decimated", "interleaved"}."decimated" ("data layout (0:decimated)"), 7:string[] ["Encoder signal", "Photo-diode", "Distance (cm)", "Photo stimulus signal", "Position in Unity", "Valve open", "Lick signal", "Frame signal", "Stimulus protocol", "VR context", "Analog lick signal", "EyeCam frame signal", "Masking light signal", "Frame signal 2", "Analog input 3"] ("channel name(s) in (Untitled)"), 9:w1626) -> ()  [unwired: 2 in, 4 out]
              }
              frame False {
                n1058 = local read "Trials in session array"() -> (w1650:u16[][])
                n1059 = local read "Encoder signal"() -> (w1637:sgl[])
                n1060 = local read "Photodiode signal"() -> (w1648:sgl[])
                n1061 = local read "total distance cm"() -> (w1646:sgl[])
                n1062 = local read "Photo stimulus signal"() -> (w1645:sgl[])
                n1063 = local read "Valve signal"() -> (w1642:i8[])
                n1064 = local read "lick signal"() -> (w1641:i8[])
                n1065 = local read "Frame signal"() -> (w1640:i8[])
                n1066 = local read "All trials"() -> (w1636:i32)
                n1067 = local read "No. of smpl. per ch."() -> (w1647:i32)
                n1068 = local read "Eye cam frame signal"() -> (w1635:i8[])
                n1069 = Index Array(array=w1650, index (row)=w1636, index (col)=0 ("disabled index (col)")) -> (element=w1638:u16)
                n1070 = Initialize Array(w1638, w1647) -> (w1639:u16[])
                n1071 = Build Array(w1637, w1648, w1646, w1645, w1642, w1641, w1640, w1639, w1635) -> (w1643:sgl[][])
                n1072 = local read "My tdms file"() -> (w1651:refnum<k34>)
                n1073 = TDMS Write(0:w1651, 1:enum16{"decimated", "interleaved"}."decimated" ("data layout (0:decimated)"), 7:string[] ["Encoder signal", "Photo-diode", "Distance (cm)", "Photo stimulus signal", "Valve open", "Lick signal", "Frame signal", "Stimulus protocol", "EyeCam frame signal"] ("channel name(s) in (Untitled)"), 9:w1643) -> ()  [unwired: 2 in, 4 out]
              }
            }
            n1074 = local read "VR Mode"() -> (w1606:bool)
            n1075 = local write "VR Mode"(w1606) -> ()
          }
        }
        n1076 = case shown="False" w1497 {
          frame True {
          }
          frame False {
            n1077 = local read "prev. diode position"() -> (w1595:dbl)
            n1078 = local read "Distance (cm)"() -> (w1596:dbl)
            n1079 = Subtract(x=w1596, y=w1595) -> (x-y=w1594:dbl)
            n1080 = local write "Track position"(w1594) -> ()
          }
        }
        n1081 = local read "index"() -> (w1553:i32)
        n1082 = Increment(x=w1553) -> (x+1=w1555:i32)
        n1083 = local read "delta distance cm"() -> (w1535:dbl[])
        n1084 = local read "No. of smpl. per ch."() -> (w1582:i32)
        n1085 = local write "index"(w1555) -> ()
        n1086 = local read "Loop rate"() -> (w1541:dbl)
        n1087 = local read "No. of smpl. per ch."() -> (w1528:i32)
        n1088 = local read "delta time (s)"() -> (w1545:dbl)
        n1089 = local read "No. of smpl. per ch."() -> (w1566:i32)
        n1090 = local read "encoder ticks per rev"() -> (w1504:dbl)
        n1091 = Add Array Elements(numeric array=w1535) -> (sum=w1538:dbl)
        n1092 = Array Size(array=w1535) -> (size(s)=w1537:i32)
        n1093 = local read "Store prev encoder count"() -> (w1531:dbl)
        n1094 = local read "Start time"() -> (w1562:u32)
        n1095 = call-poly <vilib>:"DAQmx Read.vi"("task/channels in"=w1579, "number of samples per channel"=w1582, "error in"=w1578) -> ("task out"=w1572:refnum<k21>, "data"=w1569:dbl[], "error out"=w1571:errorcluster)  [unwired: 10 in]
        n1096 = local read "Wheel circumference"() -> (w1586:dbl)
        n1097 = Divide(x=w1538, y=w1537) -> (x/y=w1536:dbl)
        n1098 = Divide(x=w1541, y=50.0) -> (x/y=w1539:dbl)
        n1099 = Add(x=w1550, y=w1536) -> (x+y=w1544:dbl)
        n1100 = Add(x=w1546, y=w1545) -> (x+y=w1543:dbl)
        n1101 = Subtract(x=w1569, y=40000.0) -> (x-y=w1500:dbl[])
        "Encoder signal" <- w1500
        n1102 = call-poly <vilib>:"DAQmx Read.vi"("task/channels in"=w1524, "number of samples per channel"=w1528, "error in"=w1527) -> ("task out"=w1521:refnum<k21>, "data"=w1475:dbl[][], "error out"=w1526:errorcluster)  [unwired: 10 in]
        n1103 = Index Array(array=w1475, index (row)=2 ("index")) -> (element=→"analog lick":dbl[])  [unwired: 1 in]
        n1104 = Index Array(array=w1475, index (row)=4 ("index")) -> (element=→"ML signal":dbl[])  [unwired: 1 in]
        n1105 = Index Array(array=w1475, index (row)=5 ("index")) -> (element=→"Analog 3":dbl[])  [unwired: 1 in]
        n1106 = call-poly <vilib>:"DAQmx Read.vi"("task/channels in"=w1574, "number of samples per channel"=w1566, "error in"=w1573) -> ("task out"=w1565:refnum<k21>, "data"=w1481:u8[][], "error out"=w1564:errorcluster)  [unwired: 10 in]
        n1107 = local read "index"() -> (w1554:i32)
        n1108 = Tick Count (ms)() -> (millisecond timer value=w1568:u32)
        n1109 = Index Array(array=w1500, index=0) -> (element=w1530:dbl)
        n1110 = Subtract(x=w1568, y=w1562) -> (x-y=w1525:u32)
        "Experiment time (ms)" <- w1525
        n1111 = Divide(x=w1500, y=w1504) -> (x/y=w1588:dbl[])
        n1112 = Greater Or Equal?(x=w1554, y=w1539) -> (x >= y?=w1542:bool)
        n1113 = Add(x=w1531, y=w1530) -> (x+y=w1529:dbl)
        "Encoder count" <- w1529
        n1114 = Multiply(x=w1588, y=w1586) -> (x*y=w1503:dbl[])
        "total distance cm" <- w1503
        n1115 = Index Array(array=w1475, index (row)=0 ("index")) -> (element=w1485:dbl[])  [unwired: 1 in]
        "Opt stim command" <- w1485
        n1116 = Index Array(array=w1475, index (row)=1 ("index")) -> (element=w1479:dbl[])  [unwired: 1 in]
        "Photodiode signal" <- w1479
        n1117 = Index Array(array=w1475, index (row)=3 ("index")) -> (element=w1490:dbl[])  [unwired: 1 in]
        n1118 = Index Array(array=w1481, index (row)=3) -> (element=w1480:u8[])  [unwired: 1 in]
        n1119 = Index Array(array=w1481, index (row)=1) -> (element=w1577:u8[])  [unwired: 1 in]
        n1120 = Index Array(array=w1481, index (row)=0) -> (element=w1515:u8[])  [unwired: 1 in]
        n1121 = Subtract(x=w1525, y=w1561) -> (x-y=w1548:u32)
        "Delta time (ms)" <- w1548
        n1122 = case shown="True" w1542 {
          tunnel: [w1598 0.0] -> w1551
          tunnel: [w1599 0.0] -> w1552
          tunnel: w1544 -> [w1599 w1603]
          tunnel: w1543 -> [w1598 w1602]
          frame False {
          }
          frame True {
            n1123 = Divide(x=w1603, y=w1602) -> (x/y=w1600:dbl)
            "Velocity chart" <- w1600
            "Velocity chart 2" <- w1600
            n1124 = local write "index"(0 ("index")) -> ()
            n1125 = local write "velocity (cm/s)"(w1600) -> ()
          }
        }
        n1126 = local write "Photo stimulus signal"(w1485) -> ()
        n1127 = Index Array(array=w1503, index=0) -> (element=w1583:dbl)
        n1128 = Divide(x=w1577, y=32.0) -> (x/y=w1506:dbl[])
        "lick signal" <- w1506
        n1129 = Divide(x=w1480, y=8.0) -> (x/y=→"Frame signal 2":dbl[])
        n1130 = Divide(x=w1515, y=16.0) -> (x/y=→"Frame signal":dbl[])
        n1131 = Divide(x=w1490, y=3.3) -> (x/y=w1491:dbl[])
        n1132 = Array Max & Min(array=w1479) -> (max value=w1478:dbl)  [unwired: 3 out]
        "Waveform Chart" <- w1478
        n1133 = Quotient & Remainder(x=w1583, y=w1586) -> (x-y*floor(x/y)=→"Position on the wheel":dbl, floor(x/y)=→"Laps":dbl)
        n1134 = Round To Nearest(number=w1491) -> (nearest integer value=→"Eye cam frame signal":dbl[])
        n1135 = Divide(x=w1525, y=1000.0) -> (x/y=w1533:dbl)
        "Experiment time (s)" <- w1533
        n1136 = Divide(x=w1548, y=1000.0) -> (x/y=→"delta time (s)":dbl)
        n1137 = local read "Valve open"() -> (w1559:bool)
        n1138 = Greater?(x=w1478, y=1.5) -> (0:w1513:bool)
        "Photodiode" <- w1513
        n1139 = Add Array Elements(numeric array=w1506) -> (sum=w1508:dbl)
        n1140 = Array Size(array=w1506) -> (size(s)=w1507:i32)
        n1141 = Index Array(array=w1506, index=0) -> (element=w1556:dbl)
        n1142 = Array Max & Min(array=w1503) -> (max value=w1502:dbl)  [unwired: 3 out]
        "Distance (cm)" <- w1502
        n1143 = Subtract(x=w1503, y=w1514) -> (x-y=→"delta distance cm":dbl[])
        n1144 = Index Array(array=w1481, index (row)=2) -> (element=w1512:u8[])  [unwired: 1 in]
        n1145 = Divide(x=w1508, y=w1507) -> (x/y=w1505:dbl)
        n1146 = Boolean To (0,1)(Boolean=w1559) -> (0, 1=w1557:i16)
        n1147 = case shown="True" w1513 {
          tunnel: w1502 -> [_ w1597]
          frame False {
          }
          frame True {
            n1148 = local write "prev. diode position"(w1597) -> ()
          }
        }
        n1149 = Array Max & Min(array=w1485) -> (max value=w1496:dbl)  [unwired: 3 out]
        n1150 = local read "Run experiment"() -> (w1593:bool)
        n1151 = Divide(x=w1502, y=100.0) -> (x/y=→"Distance (m)":dbl)
        n1152 = Divide(x=w1533, y=60.0) -> (x/y=→"Time (min)":dbl)
        n1153 = Bundle(w1556, w1557) -> (→"Lick and reward chart" →"Lick and reward chart 2":cluster{dbl, i16})  [unwired: 1 in]
        n1154 = local write "Lick indicator"(w1505) -> ()
        n1155 = Divide(x=w1512, y=64.0) -> (x/y=→"Valve signal":dbl[])
        n1156 = Greater?(x=w1496, y=0.5) -> (0:w1494:bool)
        n1157 = local write "Laser ON"(w1494) -> ()
        n1158 = Select(t=Record_enum."Record VR" ("Record enum"), s=w1593, f=Record_enum."Stop data acquision" ("Record enum")) -> (s? t:f=w1591:T5)
        "Record loop state" <- w1590
      }
      frame "Record" {
        n1159 = local write "Record loop state"(w1667) -> ()
        n1160 = local read "Run experiment"() -> (w1670:bool)
        n1161 = Select(t=Record_enum."Record" ("Record enum"), s=w1670, f=Record_enum."Stop data acquision" ("Record enum")) -> (s? t:f=w1668:T5)
      }
    }
    n1162 = local write "Exit program"("Exit program") -> ()
  }
  n1163 = while {
    shift-right: [w1685] -> _
    shift-left: T4."Idle" ("Eyecam states") -> [w1687]
    shift-right: [w1684] -> _
    shift-left: _ -> [w1678]
    shift-right: [w1683] -> _
    shift-left: _ -> [w1677]
    shift-right: [w1682] -> _
    shift-left: _ -> [w1676]
    shift-right: [w1681] -> _
    shift-left: _ -> [w1675]
    shift-right: [w1680] -> _
    shift-left: _ -> [w1674]
    shift-right: [w1679] -> _
    shift-left: _ -> [w1673]
    shift-right: [w1672] -> _
    shift-left: _ -> [w1671]
    stop <- w1686 stop-if-true
    n1164 = case shown="\"Idle\", Default" w1687 {
      tunnel: [w1703 w1742 T4."Record pupille" ("Eyecam states") w1844 T4."Idle" ("Eyecam states")] -> w1685
      tunnel: [w1697 FALSE FALSE ("Exit") FALSE ("Exit") FALSE ("Exit")] -> w1686
      tunnel: [w1690 w1725 w1777 w1812 w1873] -> w1684
      tunnel: [w1691 w1720 w1776 w1814 w1872] -> w1683
      tunnel: [w1692 w1721 w1775 w1816 w1871] -> w1682
      tunnel: [w1693 w1724 w1774 w1818 w1870] -> w1681
      tunnel: [w1694 w1723 w1773 w1820 w1869] -> w1680
      tunnel: [w1695 w1722 w1772 w1823 w1868] -> w1679
      tunnel: w1678 -> [w1690 _ w1777 w1812 w1873]
      tunnel: w1677 -> [w1691 _ w1776 w1814 w1872]
      tunnel: w1676 -> [w1692 _ w1775 w1816 w1871]
      tunnel: w1675 -> [w1693 _ w1774 w1818 w1870]
      tunnel: w1674 -> [w1694 _ w1773 w1820 w1869]
      tunnel: w1673 -> [w1695 _ w1772 w1823 w1868]
      tunnel: [0 w1718 0 w1811 0] -> w1672
      tunnel: w1671 -> [_ w1717 _ w1810 _]
      frame "Idle", Default {
        n1165 = local write "Pupille image"(T2 refnum ("Security cam image")) -> ()
        n1166 = local read "Record Button 2"() -> (w1688:bool)
        n1167 = Wait (ms)(milliseconds to wait=u32 10) -> ()  [unwired: 1 out]
        n1168 = case shown="True" w1688 {
          frame False {
          }
          frame True {
            n1169 = Get Volume Info(11:path "C:/" ("path")) -> (1:w1710:i64)  [unwired: 1 in, 5 out]
            n1170 = Divide(x=w1710, y=i64 1024) -> (x/y=w1714:dbl)
            n1171 = Divide(x=w1714, y=i64 1024) -> (x/y=w1715:dbl)
            n1172 = Divide(x=w1715, y=i64 1024) -> (x/y=w1706:dbl)
            n1173 = Number To Fractional String(number=w1706, precision (6)=i16 1) -> (F-format string=w1707:string)  [unwired: 2 in]
            n1174 = Concatenate Strings("Pupil wideo will be recorded! \nAvailable disk space: " ("string"), w1707, " GB" ("string")) -> (w1704:string)
            n1175 = One Button Dialog(message=w1704) -> ()  [unwired: 1 in, 1 out]
          }
        }
        n1176 = local read "Eable eye cam"() -> (w1702:bool)
        n1177 = And(x=w1688, y=w1702) -> (x .and. y?=w1701:bool)
        n1178 = local read "Exit"() -> (w1697:bool)
        n1179 = Select(t=T4."Set params" ("Eyecam states"), s=w1701, f=T4."Idle" ("Eyecam states")) -> (s? t:f=w1703:T4)
      }
      frame "Set params" {
        n1180 = case shown="2.." w1717 {
          tunnel: [i64 100 ("Image Format Control::Offset Y") i64 102 ("Image Format Control::Offset Y") "Image Format Control::Offset Y"] -> w1722
          tunnel: [i64 100 ("Image Format Control::Offset X") i64 102 ("Image Format Control::Offset X") "Image Format Control::Offset X"] -> w1723
          tunnel: [29.0 ("Target frame rate") 28.0 ("Target frame rate") "Target frame rate"] -> w1724
          tunnel: [10.0 ("Gain") 9.0 ("Gain") "Gain"] -> w1721
          tunnel: [0.0 ("Black Level") 1.0 ("Black Level") "Black Level"] -> w1720
          tunnel: [5.0 5.5 "Exposure Time (ms)"] -> w1719
          selector: w1717 -> [_ _ w1768]
          tunnel: [1 2 w1768] -> w1718
          frame ..0 {
          }
          frame 1 {
          }
          frame 2.. {
          }
        }
        n1181 = Divide(x=1000, y=w1724) -> (x/y=w1732:dbl)
        n1182 = Multiply(x=0.9, y=w1732) -> (x*y=w1730:dbl)
        n1183 = call "Is Value Changed.vim"("value"=w1724) -> ("changed or first call?"=w1728:bool)
        n1184 = case shown="True" w1728 {
          tunnel: w1730 -> [_ w1770]
          frame False {
          }
          frame True {
            n1185 = To Quad Integer(1:w1770) -> (0:w1769:i64)
            n1186 = property on="Exposure Time (ms)" class="Slide (strict)"("Maximum"=w1769, "Scale.Maximum"=w1769, "Value"=w1769) -> ()  [unwired: 2 in, 2 out]
          }
        }
        n1187 = local read "Run experiment"() -> (w1737:bool)
        n1188 = local read "Record Button 2"() -> (w1744:bool)
        n1189 = Multiply(x=1000.0, y=w1719) -> (x*y=w1725:dbl)
        n1190 = local read "Exit"() -> (w1740:bool)
        n1191 = Not(x=w1744) -> (.not. x?=w1739:bool)
        n1192 = Compound Arithmetic op=OR(w1737, w1739, w1740) -> (w1741:bool)
        n1193 = call "Vision Acquisition"("Analog Control::Gain"=w1721, "Analog Control::Black Level"=w1720, "Acquisition Control::Exposure Time"=w1725, "Acquisition Control::Acquisition Frame Rate"=w1724, "Image Format Control::Offset X"=w1723, "Stop (F)"=w1741, "Image Format Control::Offset Y"=w1722) -> ("Image Out"=w1746:T2, "Lost Image Count"=→"Lost Image Count":u32, "Total Images Transferred"=→"Total Images Transferred":u32, "Frame Rate"=→"Frame rate":dbl, "Stopped"=w1745:bool)  [unwired: 13 in, 3 out]
        n1194 = local write "Pupille image"(w1746) -> ()
        n1195 = Select(t=T4."Start recording" ("Eyecam states"), s=w1737, f=T4."Idle" ("Eyecam states")) -> (s? t:f=w1736:T4)
        n1196 = Select(t=w1736, s=w1745, f=T4."Set params" ("Eyecam states")) -> (s? t:f=w1742:T4)
      }
      frame "Start recording" {
        # "Wait to make sure DAQ recording \nis started before saving images"
        n1197 = disable-structure shown="Disabled" {
          frame Disabled {
            n1198 = local read "Record"() -> (w1789:bool)
            n1199 = case shown="True" w1789 {
              frame False {
              }
              frame True {
                n1200 = Get Volume Info(11:path "C:/" ("path")) -> (1:w1796:i64)  [unwired: 1 in, 5 out]
                n1201 = Divide(x=w1796, y=i64 1024) -> (x/y=w1800:dbl)
                n1202 = Divide(x=w1800, y=i64 1024) -> (x/y=w1801:dbl)
                n1203 = Divide(x=w1801, y=i64 1024) -> (x/y=w1792:dbl)
                n1204 = Number To Fractional String(number=w1792, precision (6)=i16 1) -> (F-format string=w1793:string)  [unwired: 2 in]
                n1205 = Concatenate Strings("Pupil is beeing recorded! \nAvailable disk space: " ("string"), w1793, " GB" ("string")) -> (w1790:string)
                n1206 = One Button Dialog(message=w1790) -> ()  [unwired: 1 in, 1 out]
              }
            }
          }
          frame Enabled {
          }
        }
        n1207 = property on="Image Format Control::Offset X" class="Slide (strict)"("DisabledEnum"=T6."Disabled and Grayed Out" ("Disabled")) -> ()  [unwired: 2 in, 2 out]
        n1208 = property on="Image Format Control::Offset Y" class="Slide (strict)"("DisabledEnum"=T6."Disabled and Grayed Out" ("Disabled")) -> ()  [unwired: 2 in, 2 out]
        n1209 = property on="Gain" class="Slide (strict)"("DisabledEnum"=T6."Disabled and Grayed Out" ("Disabled")) -> ()  [unwired: 2 in, 2 out]
        n1210 = property on="Target frame rate" class="DigNum (strict)"("DisabledEnum"=T6."Disabled and Grayed Out" ("Disabled")) -> ()  [unwired: 2 in, 2 out]
        n1211 = while {
          stop <- w1807 stop-if-true
          n1212 = Wait (ms)(milliseconds to wait=u32 10) -> ()  [unwired: 1 out]
          n1213 = local read "Record loop state"() -> (w1809:T5)
          n1214 = Equal?(x=w1809, y=Record_enum."Record VR" ("Record loop state")) -> (x = y?=w1807:bool)
        }
        n1215 = local read "Pupil Exp day folder"() -> (w1778:path)
        n1216 = call <vilib>:"Check if File or Folder Exists.vi"("path"=w1778) -> ("file or folder exists?"=w1780:bool, "dup path"=w1779:path)  [unwired: 8 in, 1 out]
        n1217 = case shown="False" w1780 {
          tunnel: [w1803 w1805] -> _
          tunnel: w1779 -> [w1803 w1804]
          frame True {
          }
          frame False {
            n1218 = Create Folder(path (use dialog)=w1804) -> (created path=w1805:path)  [unwired: 2 in, 2 out]
          }
        }
        n1219 = property on="Exposure Time (ms)" class="Slide (strict)"("DisabledEnum"=T6."Disabled and Grayed Out" ("Disabled")) -> ()  [unwired: 2 in, 2 out]
        n1220 = property on="Black Level" class="Slide (strict)"("DisabledEnum"=T6."Disabled and Grayed Out" ("Disabled")) -> ()  [unwired: 2 in, 2 out]
      }
      frame "Record pupille" {
        n1221 = case shown="..0" w1810 {
          tunnel: [i64 100 ("Image Format Control::Offset Y") i64 102 ("Image Format Control::Offset Y") w1861] -> w1822
          tunnel: [i64 100 ("Image Format Control::Offset X") i64 102 ("Image Format Control::Offset X") w1862] -> w1821
          tunnel: [29.0 ("Target frame rate") 28.0 ("Target frame rate") w1863] -> w1819
          tunnel: [10.0 ("Gain") 9.0 ("Gain") w1864] -> w1817
          tunnel: [0.0 ("Black Level") 1.0 ("Black Level") w1865] -> w1815
          tunnel: [5000.0 5500.0 w1866] -> w1813
          tunnel: w1812 -> [_ _ w1866]
          tunnel: w1814 -> [_ _ w1865]
          tunnel: w1816 -> [_ _ w1864]
          tunnel: w1818 -> [_ _ w1863]
          tunnel: w1820 -> [_ _ w1862]
          tunnel: w1823 -> [_ _ w1861]
          selector: w1810 -> [_ _ w1860]
          tunnel: [1 2 w1860] -> w1811
          frame ..0 {
          }
          frame 1 {
          }
          frame 2.. {
          }
        }
        n1222 = local read "Run experiment"() -> (w1842:bool)
        n1223 = local read "Exit"() -> (w1841:bool)
        n1224 = Not(x=w1842) -> (.not. x?=w1840:bool)
        n1225 = Compound Arithmetic op=OR(w1840, w1841) -> (w1839:bool)
        n1226 = call "Vision Acquisition3"("Analog Control::Gain"=w1817, "Analog Control::Black Level"=w1815, "Acquisition Control::Exposure Time"=w1813, "Acquisition Control::Acquisition Frame Rate"=w1819, "Image Format Control::Offset X"=w1821, "Stop (F)"=w1839, "Image Format Control::Offset Y"=w1822) -> ("Image Out"=w1838:T2, "Lost Image Count"=w1824:u32, "Total Images Transferred"=w1825:u32, "Frame Rate"=w1845:dbl, "Stopped"=w1837:bool)  [unwired: 13 in, 3 out]
        n1227 = local write "Frame rate"(w1845) -> ()
        n1228 = local write "Pupille image"(w1838) -> ()
        n1229 = local write "Lost Image Count"(w1824) -> ()
        n1230 = local write "Total Images Transferred"(w1825) -> ()
        n1231 = local read "Pupil Exp day folder"() -> (w1833:path)
        n1232 = local read "Run experiment"() -> (w1828:bool)
        n1233 = local read "Exit"() -> (w1830:bool)
        n1234 = local read "Record"() -> (w1827:bool)
        n1235 = local read "Filename"() -> (w1831:string)
        n1236 = Not(x=w1830) -> (.not. x?=w1829:bool)
        n1237 = Compound Arithmetic op=AND(w1827, w1828, w1829) -> (w1826:bool)
        n1238 = call "SavePupilCameraImages.vi"("Save Format"=enum16{"Png", "Raw"}."Raw", "Save Image?"=w1826, "Block Folder"=w1833, "Subfolder"=w1831, "Refnum in"=w1838) -> ("ImageSaved"=w1832:bool)  [unwired: 5 in, 1 out]
        n1239 = local write "Pupille image saved"(w1832) -> ()
        n1240 = Select(t=T4."Stop recording" ("Eyecam states"), s=w1837, f=T4."Record pupille" ("Eyecam states")) -> (s? t:f=w1844:T4)
      }
      frame "Stop recording" {
        w1874 = FALSE ("Record Button 2")
        n1241 = property on="Image Format Control::Offset X" class="Slide (strict)"("DisabledEnum"=T6."Enabled" ("Disabled")) -> ()  [unwired: 2 in, 2 out]
        n1242 = property on="Image Format Control::Offset Y" class="Slide (strict)"("DisabledEnum"=T6."Enabled" ("Disabled")) -> ()  [unwired: 2 in, 2 out]
        n1243 = local write "Record Button 2"(w1874) -> ()
        n1244 = local write "Pupille image saved"(w1874) -> ()
        n1245 = property on="Gain" class="Slide (strict)"("DisabledEnum"=T6."Enabled" ("Disabled")) -> ()  [unwired: 2 in, 2 out]
        n1246 = property on="Target frame rate" class="DigNum (strict)"("DisabledEnum"=T6."Enabled" ("Disabled")) -> ()  [unwired: 2 in, 2 out]
        n1247 = property on="Exposure Time (ms)" class="Slide (strict)"("DisabledEnum"=T6."Enabled" ("Disabled")) -> ()  [unwired: 2 in, 2 out]
        n1248 = property on="Black Level" class="Slide (strict)"("DisabledEnum"=T6."Enabled" ("Disabled")) -> ()  [unwired: 2 in, 2 out]
      }
    }
    "Eyecam states" <- w1685
  }
  n1249 = while {
    stop <- w1886 stop-if-true
    n1250 = local read "Eable security cam"() -> (w1884:bool)
    n1251 = local read "Cam ON /OFF"() -> (w1885:bool)
    n1252 = Wait (ms)(milliseconds to wait=u32 20) -> ()  [unwired: 1 out]
    n1253 = And(x=w1885, y=w1884) -> (x .and. y?=w1883:bool)
    n1254 = case shown="True" w1883 {
      frame False {
        n1255 = local write "Security cam image"(T2 refnum ("Security cam image")) -> ()
      }
      frame True {
        n1256 = while {
          stop <- w1890 stop-if-true
          n1257 = local read "Cam ON /OFF"() -> (w1896:bool)
          n1258 = Not(x=w1896) -> (.not. x?=w1895:bool)
          n1259 = call "Vision Acquisition2"("Stop (F)"=w1895) -> ("Image Out"=→"Security cam image":T2, "Stopped"=w1892:bool, "error out"=w1894:errorcluster)  [unwired: 24 in]
          n1260 = local read "Exit"() -> (w1889:bool)
          n1261 = call <vilib>:"Find First Error.vi"("error in (no error)"=w1894) -> ("error?"=w1891:bool)  [unwired: 3 in, 1 out]
          n1262 = Compound Arithmetic op=OR(w1891, w1892, w1889) -> (w1890:bool)
        }
      }
    }
    n1263 = local read "Exit"() -> (w1886:bool)
  }
  n1264 = while {
    shift-right: [w1902] -> _
    shift-left: _ -> [w1901]
    shift-right: [w1903] -> _
    shift-left: _ -> [w1900]
    shift-right: [w1898] -> _
    shift-left: w112 -> [w1899]
    stop <- w1897 stop-if-true
    n1265 = case shown="\"Socket connected\"" w1899 {
      tunnel: [w1911 w1947 w2021 w2032] -> w1903
      tunnel: [w1912 w1949 w2022 w2033] -> w1902
      tunnel: w1901 -> [_ w1949 w2024 w2033]
      tunnel: w1900 -> [_ w1947 w2023 w2032]
      tunnel: [w1908 w1946 Socket_enum."Socket not connected" ("Enum") w2031] -> w1898
      tunnel: [w1907 FALSE FALSE ("Exit") w2027] -> w1897
      frame "Init socket", Default {
        n1266 = local read "Unity connected"() -> (w1906:bool)
        n1267 = local write "Read loop stopped"(FALSE ("Read loop stopped")) -> ()
        n1268 = local write "Write loop stopped"(FALSE ("Read loop stopped")) -> ()
        n1269 = local write "Unity connected"(FALSE ("Unity connected")) -> ()
        n1270 = case shown="False" w1906 {
          frame False {
            n1271 = flat-sequence {
              frame #0 {
                n1272 = Wait (ms)(milliseconds to wait=u32 200) -> ()  [unwired: 1 out]
              }
              frame #1 {
                n1273 = local read "command line"() -> (w1919:string)
                n1274 = property on="working directory 2" class="Path"("Visible"=FALSE) -> ()  [unwired: 2 in, 2 out]
                n1275 = call <vilib>:"System Exec.vi"("run minimized? (F)"=FALSE, "wait until completion? (T)"=FALSE, "working directory"="working directory 2", "command line"=w1919) -> ()  [unwired: 4 in, 4 out]
              }
              frame #2 {
                n1276 = Wait (ms)(milliseconds to wait=u32 800) -> ()  [unwired: 1 out]
              }
            }
          }
          frame True {
          }
        }
        n1277 = call <vilib>:"TCP Listen.vi"("timeout ms (wait forever: -1)"=10000, "port"=u16 11000) -> ("error out"=w1909:errorcluster, "connection ID"=w1910:refnum<k5>)  [unwired: 5 in, 3 out]
        n1278 = case shown="No Error" w1909 {
          tunnel: [w1932 w1938] -> w1912
          tunnel: [w1931 w1937] -> w1911
          tunnel: w1910 -> [w1930 w1938]
          tunnel: w1909 -> [w1929 w1937]
          tunnel: [Socket_enum."Socket connected" ("Enum") w1935] -> w1908
          frame No Error {
            n1279 = TCP Write(connection ID=w1930, data in="Start", error in (no error)=w1929, 9:-1 ("timeout ms (25000)")) -> (connection ID out=w1926:refnum<k5>, error out=w1924:errorcluster)  [unwired: 1 out]
            n1280 = TCP Write(connection ID=w1926, data in="Start", error in (no error)=w1924) -> (connection ID out=w1932:refnum<k5>, error out=w1931:errorcluster)  [unwired: 1 in, 1 out]
          }
          frame Error {
            n1281 = local read "VR Mode"() -> (w1936:bool)
            n1282 = Select(t=Socket_enum."Init socket" ("Enum"), s=w1936, f=Socket_enum."Socket not connected" ("Enum")) -> (s? t:f=w1935:T8)
          }
        }
        n1283 = local read "Exit"() -> (w1907:bool)
      }
      frame "Socket connected" {
        n1284 = Tick Count (ms)() -> (millisecond timer value=w1939:u32)
        n1285 = while {
          tunnel: w1949 -> [w1983]
          tunnel: w1947 -> [w1982]
          stop <- w1980 stop-if-true
          n1286 = local read "Write"() -> (w1981:bool)
          n1287 = case shown="True" w1981 {
            tunnel: w1983 -> [_ w1999]
            tunnel: w1982 -> [_ w1996]
            tunnel: [w1984 w1997] -> w1980
            frame False {
              n1288 = local read "Exit"() -> (w1984:bool)
            }
            frame True {
              n1289 = local read "Gain  2"() -> (w1985:dbl)
              n1290 = call "Is Value Changed.vim"("value"=w1985) -> ("changed or first call?"=w1986:bool)
              n1291 = case shown="True" w1986 {
                tunnel: [w2000 w2001] -> w1992
                tunnel: w1985 -> [_ w2004]
                frame False {
                  n1292 = local read "Encoder count"() -> (w2000:dbl)
                }
                frame True {
                  n1293 = local read "Encoder count"() -> (w2003:dbl)
                  n1294 = Multiply(x=w2003, y=w2004) -> (x*y=w2001:dbl)
                  n1295 = To Quad Integer(1:w2001) -> (0:w2002:i64)
                  n1296 = local write "Encoder count"(w2002) -> ()
                }
              }
              n1297 = local read "encoder ticks per rev"() -> (w1991:dbl)
              n1298 = local read "Read loop stopped"() -> (w1993:bool)
              n1299 = local read "Stop Unity"() -> (w1995:bool)
              n1300 = Divide(x=4000.0 ("y"), y=w1991) -> (x/y=w1989:dbl)
              n1301 = Multiply(x=w1989, y=w1992) -> (x*y=w1988:dbl)
              n1302 = And(x=w1995, y=w1993) -> (x .and. y?=w1994:bool)
              n1303 = Multiply(x=w1985, y=w1988) -> (x*y=w1987:dbl)
              n1304 = case shown="False" w1994 {
                tunnel: ["ext,\r\n" w2017] -> w1998
                tunnel: w1987 -> [_ w2016]
                tunnel: [TRUE FALSE] -> w1997
                frame True {
                  n1305 = local write "Write loop stopped"(TRUE ("Read loop stopped")) -> ()
                  n1306 = local write "Write"(FALSE ("Write")) -> ()
                  n1307 = local write "Unity connected"(FALSE ("Unity connected")) -> ()
                  n1308 = Wait (ms)(milliseconds to wait=u32 20) -> ()  [unwired: 1 out]
                }
                frame False {
                  n1309 = local read "offset tag"() -> (w2011:string)
                  n1310 = local read "msg tag"() -> (w2012:string)
                  n1311 = Number To Decimal String(number=w2016) -> (decimal integer string=w2014:string)  [unwired: 1 in]
                  n1312 = Concatenate Strings(w2012, w2011, w2014, "\r\n" ("string")) -> (w2017:string)
                }
              }
              n1313 = TCP Write(connection ID=w1999, data in=w1998, error in (no error)=w1996) -> ()  [unwired: 1 in, 3 out]
            }
          }
          n1314 = Wait (ms)(milliseconds to wait=u32 5) -> ()  [unwired: 1 out]
        }
        n1315 = while {
          tunnel: w1949 -> [w1956]
          tunnel: w1947 -> [w1957]
          shift-right: [w1951] -> _
          shift-left: w1939 -> [w1952]
          stop <- w1955 stop-if-true
          n1316 = local read "read"() -> (w1954:bool)
          n1317 = case shown="True" w1954 {
            tunnel: w1956 -> [_ w1966]
            tunnel: w1957 -> [_ w1967]
            tunnel: [w1960 FALSE] -> w1955
            frame False {
              n1318 = local write "Read loop stopped"(TRUE ("Read loop stopped")) -> ()
              n1319 = local read "Exit"() -> (w1960:bool)
            }
            frame True {
              # "msg format: pos + CorridorIndicator + \",\" Position"
              n1320 = TCP Read(connection ID=w1966, bytes to read=20, error in (no error)=w1967, 7:T16."CRLF" ("mode (standard)"), 9:-1 ("timeout ms (25000)")) -> (data out=w1973:string)  [unwired: 2 out]
              n1321 = Match Pattern(string=w1973, regular expression=",", offset (0)=0) -> (after substring=w1977:string)  [unwired: 3 out]
              n1322 = Match Pattern(string=w1973, regular expression="pos") -> (after substring=w1970:string)  [unwired: 1 in, 3 out]
              n1323 = Match Pattern(string=w1970, regular expression="," ("after substring")) -> (before substring=w1969:string)  [unwired: 1 in, 3 out]
              n1324 = Match Pattern(string=w1977, regular expression="\\r\\n" ("after substring")) -> (before substring=w1975:string)  [unwired: 1 in, 3 out]
              n1325 = Decimal String To Number(string=w1969) -> ()  [unwired: 2 in, 2 out]
              n1326 = Fract/Exp String To Number(string=w1975) -> (number=w1961:dbl)  [unwired: 3 in, 1 out]
              n1327 = local write "Read loop stopped"(FALSE ("Read loop stopped")) -> ()
              n1328 = local write "Track position"(w1961) -> ()
            }
          }
          n1329 = local write "Unity connected"(TRUE ("Unity connected")) -> ()
          n1330 = Tick Count (ms)() -> (millisecond timer value=w1951:u32)
          n1331 = Subtract(x=w1951, y=w1952) -> (x-y=→"Socket read loop rate":u32)
          n1332 = Wait (ms)(milliseconds to wait=u32 1) -> ()  [unwired: 1 out]
        }
        n1333 = local read "Stop Unity"() -> (w1943:bool)
        n1334 = local read "Exit"() -> (w1942:bool)
        n1335 = Compound Arithmetic op=OR(w1942, w1943) -> (w1941:bool)
        n1336 = Wait (ms)(milliseconds to wait=u32 10) -> ()  [unwired: 1 out]
        n1337 = Select(t=Socket_enum."Close socket" ("Enum"), s=w1941, f=Socket_enum."Socket connected" ("Enum")) -> (s? t:f=w1946:T8)
      }
      frame "Close socket" {
        n1338 = TCP Close Connection(connection ID=w2024, error in (no error)=w2023) -> (connection ID out=w2022:refnum<k5>, error out=w2021:errorcluster)  [unwired: 1 in]
        n1339 = local write "Unity connected"(FALSE ("Unity connected")) -> ()
      }
      frame "Socket not connected" {
        n1340 = local write "Unity connected"(FALSE ("Unity connected")) -> ()
        n1341 = Wait (ms)(milliseconds to wait=u32 1000) -> ()  [unwired: 1 out]
        n1342 = local read "VR Mode"() -> (w2030:bool)
        n1343 = local read "Exit"() -> (w2027:bool)
        n1344 = Select(t=Socket_enum."Init socket" ("Enum"), s=w2030, f=Socket_enum."Socket not connected" ("Enum")) -> (s? t:f=w2031:T8)
      }
    }
  }
  n1345 = property on="Record Button" class="Bool (strict)"("DisabledEnum"=w5) -> ()  [unwired: 2 in, 2 out]
  n1346 = property on="Stop recording" class="Bool (strict)"("DisabledEnum"=T6."Enabled" ("Disabled")) -> ()  [unwired: 2 in, 2 out]
  n1347 = property on="Start recording" class="Bool (strict)"("DisabledEnum"=w5) -> ()  [unwired: 2 in, 2 out]
  n1348 = local write "Exit program"(FALSE ("Exit program")) -> ()
  n1349 = local write "Stop Unity"(FALSE ("Stop Unity")) -> ()
  n1350 = local write "Exit"(FALSE ("Exit")) -> ()
  n1351 = local write "Record"(FALSE ("Logg data")) -> ()
  n1352 = local write "Start recording"(FALSE ("Start recording")) -> ()
  n1353 = local write "Record Button"(FALSE ("Record Button")) -> ()
  n1354 = local write "Gain  2"(1.0 ("Gain")) -> ()
  n1355 = local read "Stim prot command"() -> (w68:u16)
  n1356 = local read "Stim prot command"() -> (w30:u16)
  n1357 = local read "protocol array"() -> (w72:string[][])
  n1358 = local read "protocol array"() -> (w27:string[][])
  n1359 = local write "Store prev encoder count"(0.0 ("Store prev encoder count")) -> ()
  n1360 = Index Array(array=w72, index (row)=w68, index (col)=0 ("index (row)")) -> (element=w65:string)
  n1361 = Index Array(array=w72, index (row)=w68, index (col)=1 ("disabled index (col)")) -> (element=w56:string)
  n1362 = Index Array(array=w72, index (row)=w68, index (col)=2 ("disabled index (col)")) -> (element=w51:string)
  n1363 = Index Array(array=w72, index (row)=w68, index (col)=3 ("disabled index (col)")) -> (element=w50:string)
  n1364 = Index Array(array=w27, index (row)=w30, index (col)=0 ("index (row)")) -> (element=w33:string)
  n1365 = Index Array(array=w27, index (row)=w30, index (col)=1 ("disabled index (col)")) -> (element=w42:string)
  n1366 = Index Array(array=w27, index (row)=w30, index (col)=2 ("disabled index (col)")) -> (element=w47:string)
  n1367 = local read "Reward given"() -> (w9:u32)
  n1368 = local write "Open valve"(FALSE ("Open valve")) -> ()
  n1369 = local read "Reward given"() -> (w10:u32)
  n1370 = local write "Reward freq. (cm)"(100.0 ("Reward freq. (cm)")) -> ()
  n1371 = local write "Timed reward (s)"(u32 0 ("Timed reward (s)")) -> ()
  n1372 = local write "random rew"(0.5 ("random rew")) -> ()
  n1373 = Match Pattern(string=w65, regular expression=w61) -> (match substring=w62:string)  [unwired: 1 in, 3 out]
  n1374 = Match Pattern(string=w65, regular expression=" Hz") -> (before substring=w66:string)  [unwired: 1 in, 3 out]
  n1375 = Match Pattern(string=w65, regular expression=w63) -> (match substring=w64:string)  [unwired: 1 in, 3 out]
  n1376 = Match Pattern(string=w56, regular expression="from ") -> (after substring=w59:string)  [unwired: 1 in, 3 out]
  n1377 = Match Pattern(string=w56, regular expression=w57) -> (match substring=w58:string)  [unwired: 1 in, 3 out]
  n1378 = Match Pattern(string=w51, regular expression="to ") -> (after substring=w53:string)  [unwired: 1 in, 3 out]
  n1379 = Match Pattern(string=w51, regular expression=w55) -> (match substring=w54:string)  [unwired: 1 in, 3 out]
  n1380 = Match Pattern(string=w50, regular expression=" %") -> (before substring=w48:string)  [unwired: 1 in, 3 out]
  n1381 = Match Pattern(string=w33, regular expression=w37) -> (match substring=w36:string)  [unwired: 1 in, 3 out]
  n1382 = Match Pattern(string=w33, regular expression=" Hz") -> (before substring=w32:string)  [unwired: 1 in, 3 out]
  n1383 = Match Pattern(string=w33, regular expression=w35) -> (match substring=w34:string)  [unwired: 1 in, 3 out]
  n1384 = Match Pattern(string=w42, regular expression="from ") -> (after substring=w39:string)  [unwired: 1 in, 3 out]
  n1385 = Match Pattern(string=w42, regular expression=w41) -> (match substring=w40:string)  [unwired: 1 in, 3 out]
  n1386 = Match Pattern(string=w47, regular expression="to ") -> (after substring=w45:string)  [unwired: 1 in, 3 out]
  n1387 = Match Pattern(string=w47, regular expression=w43) -> (match substring=w44:string)  [unwired: 1 in, 3 out]
  n1388 = local write "Water cnt. reset"(0 ("Waret received")) -> ()
  n1389 = call-poly <vilib>:"DAQmx Create Virtual Channel.vi"("lines"=tag "Dev1/port2/line6") -> ("task out"=w95:refnum<k21>)  [unwired: 13 in, 1 out]
  n1390 = call-poly <vilib>:"DAQmx Create Virtual Channel.vi"("lines"=tag "Dev1/port2/line5") -> ("task out"=w97:refnum<k21>)  [unwired: 13 in, 1 out]
  n1391 = local write "Valve open"(FALSE ("Valve open")) -> ()
  n1392 = local write "Repetition"(1 ("Repetition")) -> ()
  n1393 = local write "miss trial"(FALSE ("miss trial")) -> ()
  n1394 = Equal?(x=w9, y=u32 0) -> ()  [unwired: 1 out]
  n1395 = Equal?(x=w62, y=w61) -> ()  [unwired: 1 out]
  n1396 = Equal?(x=w64, y=w63) -> ()  [unwired: 1 out]
  n1397 = Equal?(x=w58, y=w57) -> ()  [unwired: 1 out]
  n1398 = Equal?(x=w54, y=w55) -> ()  [unwired: 1 out]
  n1399 = Equal?(x=w36, y=w37) -> ()  [unwired: 1 out]
  n1400 = Equal?(x=w34, y=w35) -> ()  [unwired: 1 out]
  n1401 = Equal?(x=w40, y=w41) -> ()  [unwired: 1 out]
  n1402 = Equal?(x=w44, y=w43) -> ()  [unwired: 1 out]
  n1403 = Decimal String To Number(string=w66) -> ()  [unwired: 2 in, 2 out]
  n1404 = Decimal String To Number(string=w59) -> ()  [unwired: 2 in, 2 out]
  n1405 = Decimal String To Number(string=w53) -> ()  [unwired: 2 in, 2 out]
  n1406 = Decimal String To Number(string=w48) -> ()  [unwired: 2 in, 2 out]
  n1407 = Decimal String To Number(string=w32) -> ()  [unwired: 2 in, 2 out]
  n1408 = Decimal String To Number(string=w39) -> ()  [unwired: 2 in, 2 out]
  n1409 = Decimal String To Number(string=w45) -> ()  [unwired: 2 in, 2 out]
  n1410 = Greater?(x=w10, y=u32 0) -> ()  [unwired: 1 out]
  n1411 = Tick Count (ms)() -> (millisecond timer value=w87:u32)
  n1412 = while {
    shift-right: [w2084] -> _
    shift-left: _ -> [w2083]
    stop <- w2085 stop-if-true
    w2059 = 100.0 ("y")
    # "Reward zone available?"
    n1413 = case shown="True" TRUE {
      tunnel: [w2163 w2236] -> w2084
      tunnel: w2083 -> [w2158 w2231]
      frame True {
        # "Clear graph history in every 3 min"
        n1414 = local read "Trials in session array"() -> (w2137:u16[][])
        n1415 = local read "Record loop state"() -> (w2132:T5)
        n1416 = local read "All trials"() -> (w2136:i32)
        n1417 = Tick Count (ms)() -> (millisecond timer value=w2162:u32)
        n1418 = local read "Stim trial"() -> (w2150:bool)
        n1419 = local read "Stim trial"() -> (w2147:bool)
        n1420 = Divide(x=w2162, y=u32 60000) -> (x/y=w2160:dbl)
        n1421 = local read "velocity (cm/s)"() -> (w2142:dbl)
        n1422 = local read "Track position"() -> (w2133:sgl)
        "?" <- w2133
        n1423 = Subtract(x=w2160, y=w2158) -> (x-y=w2159:dbl)
        n1424 = Index Array(array=w2137, index (row)=w2136, index (col)=1 ("disabled index (col)")) -> (element=w2134:u16)
        n1425 = Equal?(x=w2132, y=Record_enum."Record VR" ("Record loop state")) -> (x = y?=w2129:bool)
        n1426 = call "Is Value Changed.vim"("value"=w2129) -> ("changed or first call?"=w2130:bool)
        n1427 = Greater?(x=w2159, y=3.0) -> (0:w2126:bool)
        n1428 = Equal?(x="plot selector bool 1", y=w2150) -> (x = y?=w2152:bool)
        n1429 = Equal?(x="plot selector 1", y=w2134) -> (x = y?=w2151:bool)
        n1430 = Equal?(x=w2134, y="plot selector 2") -> (x = y?=w2153:bool)
        n1431 = Equal?(x=w2147, y="plot selector bool 2") -> (x = y?=w2154:bool)
        n1432 = And(x=w2130, y=w2129) -> (x .and. y?=w2127:bool)
        n1433 = And(x=w2152, y=w2151) -> (x .and. y?=w2144:bool)
        n1434 = And(x=w2153, y=w2154) -> (x .and. y?=w2143:bool)
        n1435 = Or(x=w2127, y=w2126) -> (x .or. y?=w2128:bool)
        n1436 = case shown="False" w2128 {
          tunnel: [w2213 w2222] -> w2163
          tunnel: w2158 -> [w2214 _]
          tunnel: ["Reset bottom plot" w2221] -> w2156
          tunnel: ["Reset top plot" w2221] -> w2155
          frame False {
            n1437 = Or(x="Reset bottom plot", y="Reset top plot") -> (x .or. y?=w2212:bool)
            n1438 = case shown="True" w2212 {
              tunnel: w2214 -> [w2217 _]
              tunnel: [w2217 w2218] -> w2213
              frame False {
              }
              frame True {
                n1439 = Tick Count (ms)() -> (millisecond timer value=w2220:u32)
                n1440 = Divide(x=w2220, y=u32 60000) -> (x/y=w2218:dbl)
              }
            }
          }
          frame True {
            w2221 = TRUE ("Reset NBC plot")
            n1441 = Tick Count (ms)() -> (millisecond timer value=w2223:u32)
            n1442 = Divide(x=w2223, y=u32 60000) -> (x/y=w2222:dbl)
          }
        }
        n1443 = call "Is New Trial - graph loop.vi"("Position data"=w2133) -> ("Boolean"=w2139:bool)  [unwired: 1 in]
        n1444 = local read "Valve open"() -> (w2172:bool)
        n1445 = local read "Valve open"() -> (w2177:bool)
        n1446 = local read "lick signal"() -> (w2187:i8[])
        n1447 = local read "lick signal"() -> (w2196:i8[])
        n1448 = call "Is Value Changed.vim"("value"=w2139) -> ("changed or first call?"=w2138:bool)
        n1449 = case shown="False" w2139 {
          tunnel: [w2208 w2210] -> w2140
          tunnel: w2142 -> [w2209 w2210]
          tunnel: w2133 -> [w2205 _]
          tunnel: [w2207 inf ("velocity (cm/s)")] -> w2141
          tunnel: w2138 -> [w2204 _]
          frame False {
            n1450 = Select(t=-inf ("velocity (cm/s)"), s=w2204, f=w2205) -> (s? t:f=w2207:dbl)
            n1451 = Select(t=-99.0, s=w2204, f=w2209) -> (s? t:f=w2208:dbl)
          }
          frame True {
          }
        }
        n1452 = Index Array(array=w2187, index=0) -> (element=w2189:i8)
        n1453 = Boolean To (0,1)(Boolean=w2172) -> (0, 1=w2170:i16)
        n1454 = Index Array(array=w2196, index=0) -> (element=w2193:i8)
        n1455 = Boolean To (0,1)(Boolean=w2177) -> (0, 1=w2175:i16)
        n1456 = Multiply(x=w2189, y=100) -> (x*y=w2164:i32)
        n1457 = Multiply(x=w2170, y=-20) -> (x*y=w2171:i32)
        n1458 = Multiply(x=w2193, y=100) -> (x*y=w2192:i32)
        n1459 = Multiply(x=w2175, y=-20) -> (x*y=w2176:i32)
        n1460 = call "Build XY Graph"("Enable"=w2144, "Reset"=w2155, "Y Input"=w2140, "X Input"=w2141) -> ("XY Graph"=w2198:cluster{"X":dbl[], "Y":dbl[]}[])  [unwired: 6 in, 1 out]
        n1461 = call "Build XY Graph4"("Enable"=w2144, "Reset"=w2155, "Y Input"=w2192, "X Input"=w2141) -> ("XY Graph"=w2201:cluster{"X":dbl[], "Y":dbl[]}[])  [unwired: 6 in, 1 out]
        n1462 = call "Build XY Graph3"("Enable"=w2144, "Reset"=w2155, "Y Input"=w2176, "X Input"=w2141) -> ("XY Graph"=w2186:cluster{"X":dbl[], "Y":dbl[]}[])  [unwired: 6 in, 1 out]
        n1463 = call "Build XY Graph2"("Enable"=w2143, "Reset"=w2156, "Y Input"=w2164, "X Input"=w2141) -> ("XY Graph"=w2178:cluster{"X":dbl[], "Y":dbl[]}[])  [unwired: 6 in, 1 out]
        n1464 = call "Build XY Graph5"("Enable"=w2143, "Reset"=w2156, "Y Input"=w2140, "X Input"=w2141) -> ("XY Graph"=w2183:cluster{"X":dbl[], "Y":dbl[]}[])  [unwired: 6 in, 1 out]
        n1465 = call "Build XY Graph6"("Enable"=w2143, "Reset"=w2156, "Y Input"=w2171, "X Input"=w2141) -> ("XY Graph"=w2181:cluster{"X":dbl[], "Y":dbl[]}[])  [unwired: 6 in, 1 out]
        n1466 = Index Array(array=w2198, index=0) -> (element=w2165:cluster{"X":dbl[], "Y":dbl[]})
        n1467 = Index Array(array=w2201, index=0) -> (element=w2197:cluster{"X":dbl[], "Y":dbl[]})
        n1468 = Index Array(array=w2186, index=0) -> (element=w2182:cluster{"X":dbl[], "Y":dbl[]})
        n1469 = Index Array(array=w2183, index=0) -> (element=w2169:cluster{"X":dbl[], "Y":dbl[]})
        n1470 = Index Array(array=w2178, index=0) -> (element=w2168:cluster{"X":dbl[], "Y":dbl[]})
        n1471 = Index Array(array=w2181, index=0) -> (element=w2167:cluster{"X":dbl[], "Y":dbl[]})
        n1472 = Build Array(w2169, w2168, w2167) -> (→"Bottom Graph":cluster{"X":dbl[], "Y":dbl[]}[])
        n1473 = Build Array(w2165, w2197, w2182) -> (→"Top Graph":cluster{"X":dbl[], "Y":dbl[]}[])
        n1474 = Wait (ms)(milliseconds to wait=u32 20) -> ()  [unwired: 1 out]
      }
      frame False {
        # "Clear graph history in every 5 min"
        n1475 = local read "Reward zone"() -> (w2226:bool)
        n1476 = Tick Count (ms)() -> (millisecond timer value=w2235:u32)
        n1477 = case shown="False" w2226 {
          tunnel: [w2258 w2260] -> w2227
          frame False {
            n1478 = local read "Distance (cm)"() -> (w2257:dbl)
            n1479 = local read "Prev. rew. pos."() -> (w2259:dbl)
            n1480 = Subtract(x=w2257, y=w2259) -> (x-y=w2258:dbl)
          }
          frame True {
            n1481 = local read "Track position"() -> (w2260:sgl)
          }
        }
        n1482 = Divide(x=w2235, y=u32 60000) -> (x/y=w2233:dbl)
        n1483 = Subtract(x=w2233, y=w2231) -> (x-y=w2232:dbl)
        n1484 = Greater?(x=w2232, y=2.0) -> (0:w2228:bool)
        n1485 = case shown="True" w2228 {
          tunnel: [w2262 w2269] -> w2236
          tunnel: w2231 -> [w2263 _]
          tunnel: ["Reset wheel pos. graph" TRUE ("Reset NBC plot")] -> w2229
          frame False {
            n1486 = case shown="False" "Reset wheel pos. graph" {
              tunnel: w2263 -> [w2264 _]
              tunnel: [w2264 w2265] -> w2262
              frame False {
              }
              frame True {
                n1487 = Tick Count (ms)() -> (millisecond timer value=w2267:u32)
                n1488 = Divide(x=w2267, y=u32 60000) -> (x/y=w2265:dbl)
              }
            }
          }
          frame True {
            n1489 = Tick Count (ms)() -> (millisecond timer value=w2270:u32)
            n1490 = Divide(x=w2270, y=u32 60000) -> (x/y=w2269:dbl)
          }
        }
        n1491 = local read "lick signal"() -> (w2250:i8[])
        n1492 = local read "Valve open"() -> (w2241:bool)
        n1493 = local read "velocity (cm/s)"() -> (w2225:dbl)
        n1494 = Index Array(array=w2250, index=0) -> (element=w2247:i8)
        n1495 = Boolean To (0,1)(Boolean=w2241) -> (0, 1=w2239:i16)
        n1496 = Multiply(x=w2247, y=100) -> (x*y=w2246:i32)
        n1497 = Multiply(x=w2239, y=-20) -> (x*y=w2240:i32)
        n1498 = call "Build XY Graph7"("Reset"=w2229, "Y Input"=w2225, "X Input"=w2227) -> ("XY Graph"=w2252:cluster{"X":dbl[], "Y":dbl[]}[])  [unwired: 7 in, 1 out]
        n1499 = call "Build XY Graph8"("Reset"=w2229, "Y Input"=w2246, "X Input"=w2227) -> ("XY Graph"=w2255:cluster{"X":dbl[], "Y":dbl[]}[])  [unwired: 7 in, 1 out]
        n1500 = call "Build XY Graph9"("Reset"=w2229, "Y Input"=w2240, "X Input"=w2227) -> ("XY Graph"=w2244:cluster{"X":dbl[], "Y":dbl[]}[])  [unwired: 7 in, 1 out]
        n1501 = Index Array(array=w2252, index=0) -> (element=w2237:cluster{"X":dbl[], "Y":dbl[]})
        n1502 = Index Array(array=w2255, index=0) -> (element=w2251:cluster{"X":dbl[], "Y":dbl[]})
        n1503 = Index Array(array=w2244, index=0) -> (element=w2242:cluster{"X":dbl[], "Y":dbl[]})
        n1504 = Build Array(w2237, w2251, w2242) -> (→"Wheel position graph":cluster{"X":dbl[], "Y":dbl[]}[])
        n1505 = Wait (ms)(milliseconds to wait=u32 20) -> ()  [unwired: 1 out]
      }
    }
    n1506 = disable-structure shown="Disabled" {
      frame Disabled {
        n1507 = local read "VR Mode"() -> ()  [unwired: 1 out]
      }
      frame Enabled {
      }
    }
    n1508 = local write "Stop recording"("Stop recording") -> ()
    n1509 = local write "Lab book notes"("Lab book notes") -> ()
    n1510 = local write "SciScan"("SciScan") -> ()
    n1511 = local write "Reward zone"("Reward zone") -> ()
    n1512 = Not(x="Reward zone") -> (.not. x?=w2075:bool)
    n1513 = property on="Reward freq. (cm)" class="DigNum (strict)"("Visible"=w2075) -> ()  [unwired: 2 in, 2 out]
    n1514 = property on="Timed reward (s)" class="DigNum (strict)"("Visible"=w2075) -> ()  [unwired: 2 in, 2 out]
    n1515 = local read "Hit trials stim."() -> (w2064:i32)
    n1516 = local read "Random reward"() -> (w2069:bool)
    n1517 = local read "Hit trials ctrl."() -> (w2066:i32)
    n1518 = local read "Reward zone"() -> (w2068:bool)
    n1519 = local read "Stim. count"() -> (w2065:i32)
    n1520 = local read "current VR context"() -> (w2056:u16)
    n1521 = local read "Ctrl. count"() -> (w2067:i32)
    n1522 = local read "Context command"() -> (w2073:u16)
    n1523 = local read "Frame signal"() -> (w2036:i8[])
    n1524 = local read "zeward zones"() -> (w2057:i16[][])
    n1525 = call "Is Value Changed.vim"("value"=w2068) -> ("changed or first call?"=w2071:bool)
    n1526 = call "Is Value Changed.vim"("value"=w2069) -> ("changed or first call?"=w2070:bool)
    n1527 = local read "Reward zone"() -> (w2048:bool)
    n1528 = local read "Active licking"() -> (w2077:bool)
    n1529 = Or(x=w2071, y=w2070) -> (x .or. y?=w2072:bool)
    n1530 = call "Is Value Changed.vim"("value"=w2048) -> ("changed or first call?"=w2047:bool)
    n1531 = Divide(x=w2064, y=w2065) -> (x/y=w2061:dbl)
    "P stim. Hit" <- w2061
    n1532 = Divide(x=w2066, y=w2067) -> (x/y=w2062:dbl)
    "P ctrl. Hit" <- w2062
    n1533 = case shown="True" w2072 {
      tunnel: w2068 -> [_ w2098]
      tunnel: w2069 -> [_ w2087]
      frame False {
      }
      frame True {
        n1534 = local read "Reward freq. (cm)"() -> (w2092:u32)
        n1535 = local read "Reward freq. (cm)"() -> (w2095:u32)
        n1536 = local read "Wheel circumference"() -> (w2097:dbl)
        n1537 = Multiply(x=w2092, y=2.0) -> (x*y=w2089:dbl)
        n1538 = Add(x=w2095, y=20.0) -> (x+y=w2088:dbl)
        n1539 = Add(x=w2089, y=20.0) -> (x+y=w2091:dbl)
        n1540 = Select(t=w2091, s=w2087, f=w2088) -> (s? t:f=w2086:dbl)
        n1541 = Select(t=w2097, s=w2098, f=w2086) -> (s? t:f=w2090:dbl)
        n1542 = property on="Wheel position graph" class="XYGraph (strict)"("XScale.Maximum"=w2090) -> ()  [unwired: 2 in, 2 out]
      }
    }
    n1543 = Add Array Elements(numeric array=w2036) -> (sum=w2035:i8)
    n1544 = Array Size(array=w2036) -> (size(s)=w2046:i32)
    n1545 = Delete From Array(array=w2057, index (row)=w2056) -> (deleted portion=w2058:i16[])  [unwired: 2 in, 1 out]
    n1546 = Decimate 1D Array(w2058) -> (w2055:i16[], w2054:i16[])
    n1547 = Add Array Elements(numeric array=w2055) -> (sum=w2053:i16)
    n1548 = Add Array Elements(numeric array=w2054) -> (sum=w2052:i16)
    n1549 = Less?(x=w2053, y=w2052) -> (x < y?=w2051:bool)
    n1550 = call "Is Value Changed.vim"("value"=w2051) -> ("changed or first call?"=w2049:bool)
    n1551 = Or(x=w2047, y=w2049) -> (x .or. y?=w2050:bool)
    n1552 = call "Is Value Changed.vim"("value"=w2073) -> ("changed or first call?"=w2074:bool)
    n1553 = Divide(x=w2035, y=w2046) -> (x/y=w2045:dbl)
    n1554 = case shown="True" w2050 {
      tunnel: w2048 -> [_ w2110]
      tunnel: w2051 -> [_ w2109]
      frame False {
      }
      frame True {
        n1555 = case shown="True" w2110 {
          tunnel: w2109 -> [_ w2115]
          frame False {
            n1556 = local write "Active licking"(FALSE ("Enable")) -> ()
            n1557 = property on="Active licking" class="Bool (strict)"("DisabledEnum"=T6."Disabled and Grayed Out" ("Disabled")) -> ()  [unwired: 2 in, 2 out]
            n1558 = property on="Random reward" class="Bool (strict)"("DisabledEnum"=T6."Enabled" ("Disabled"), "Visible"=TRUE) -> ()  [unwired: 2 in, 2 out]
          }
          frame True {
            n1559 = local write "Random reward"(FALSE ("Random reward")) -> ()
            n1560 = Select(t=TRUE ("Enable"), s=w2115, f=FALSE ("Enable")) -> (s? t:f=w2121:bool)
            n1561 = Select(t=T6."Enabled" ("Disabled"), s=w2115, f=T6."Disabled and Grayed Out" ("Disabled")) -> (s? t:f=w2120:T6)
            n1562 = local write "Active licking"(w2121) -> ()
            n1563 = property on="Random reward" class="Bool (strict)"("DisabledEnum"=T6."Disabled" ("Disabled"), "Visible"=FALSE) -> ()  [unwired: 2 in, 2 out]
            n1564 = property on="Active licking" class="Bool (strict)"("DisabledEnum"=w2120) -> ()  [unwired: 2 in, 2 out]
          }
        }
      }
    }
    n1565 = case shown="True" w2074 {
      tunnel: w2073 -> [_ w2099]
      frame False {
      }
      frame True {
        n1566 = local read "corridor lengths"() -> (w2103:i32[])
        n1567 = local read "teleports"() -> (w2104:i16[])
        n1568 = Index Array(array=w2104, index=w2099) -> (element=w2102:i16)
        n1569 = Index Array(array=w2103, index=w2099) -> (element=w2101:i32)
        n1570 = Subtract(x=w2102, y=w2101) -> (x-y=w2100:i32)
        n1571 = property on="Top Graph" class="XYGraph (strict)"("XScale.Maximum"=w2102, "XScale.Minimum"=w2100) -> ()  [unwired: 2 in, 2 out]
        n1572 = property on="Bottom Graph" class="XYGraph (strict)"("XScale.Maximum"=w2102, "XScale.Minimum"=w2100) -> ()  [unwired: 2 in, 2 out]
        n1573 = property on="Position bar" class="Slide (strict)"("Scale.Maximum"=w2102, "Scale.Minimum"=w2100) -> ()  [unwired: 2 in, 2 out]
      }
    }
    n1574 = call "Is Value Changed.vim"("value"=w2077) -> ("changed or first call?"=w2076:bool)
    n1575 = Greater?(x=w2045, y=0.1) -> (0:→"Frame signal indicator":bool)
    n1576 = case shown="True" w2076 {
      frame False {
      }
      frame True {
        n1577 = local read "Active licking"() -> (w2105:bool)
        n1578 = Select(t=T6."Enabled" ("Disabled"), s=w2105, f=T6."Disabled and Grayed Out") -> (s? t:f=w2107:T6)
        n1579 = property on="Hybrid licking" class="Bool (strict)"("DisabledEnum"=w2107) -> ()  [unwired: 2 in, 2 out]
      }
    }
    n1580 = Multiply(x=w2062, y=w2059) -> (x*y=→"Control hit trials %":dbl)
    n1581 = Multiply(x=w2059, y=w2061) -> (x*y=→"Stim. hit trials %":dbl)
    n1582 = local read "Frame signal 2"() -> (w2037:i8[])
    n1583 = Add Array Elements(numeric array=w2037) -> (sum=w2039:i8)
    n1584 = Array Size(array=w2037) -> (size(s)=w2040:i32)
    n1585 = case shown="True" "Random reward" {
      frame False {
      }
      frame True {
        n1586 = local write "Active licking"(FALSE ("Enable")) -> ()
      }
    }
    n1587 = Divide(x=w2039, y=w2040) -> (x/y=w2041:dbl)
    n1588 = Greater?(x=w2041, y=0.1) -> (0:→"Frame signal indicator 2":bool)
    n1589 = local read "Exit"() -> (w2085:bool)
  }
  n1590 = while {
    tunnel: w97 -> [w2300]
    tunnel: w95 -> [w2290]
    shift-right: [w2292] -> _
    shift-left: w87 -> [w2291]
    shift-right: [w2282] -> _
    shift-left: _ -> [w2281]
    stop <- w2306 stop-if-true
    n1591 = local read "Repetition"() -> (w2302:i32)
    n1592 = local read "Reward zone"() -> (w2294:bool)
    n1593 = case shown="True" w2294 {
      tunnel: [w2348 w2408] -> w2274
      tunnel: [w2352 w2407] -> w2295
      tunnel: w2281 -> [w2350 _]
      tunnel: [w2349 w2406] -> w2279
      tunnel: [w2347 w2405] -> w2277
      frame False {
        n1594 = local read "Random reward"() -> (w2351:bool)
        n1595 = case shown="True" w2351 {
          tunnel: [w2353 FALSE] -> w2352
          tunnel: w2350 -> [w2357 w2399]
          tunnel: [w2353 w2380] -> w2349
          tunnel: [FALSE ("Active rew within RZ") w2378] -> w2348
          tunnel: [FALSE ("Passive rew after RZ") w2375] -> w2347
          frame True {
            n1596 = local read "Reward freq. (cm)"() -> (w2371:u32)
            n1597 = local read "Timed reward (s)"() -> (w2366:u32)
            n1598 = local read "random rew"() -> (w2369:dbl)
            n1599 = local read "Prev. rew. pos."() -> (w2373:dbl)
            n1600 = local read "Distance (cm)"() -> (w2374:dbl)
            n1601 = Tick Count (ms)() -> (millisecond timer value=w2365:u32)
            n1602 = Multiply(x=w2366, y=u32 1000) -> (x*y=w2362:u32)
            n1603 = Multiply(x=w2371, y=2.0) -> (x*y=w2368:dbl)
            n1604 = Add(x=w2357, y=w2362) -> (x+y=w2364:u32)
            n1605 = Multiply(x=w2368, y=w2369) -> (x*y=w2367:dbl)
            n1606 = Greater?(x=w2362, y=u32 999) -> (0:w2361:bool)
            n1607 = Greater?(x=w2365, y=w2364) -> (0:w2363:bool)
            n1608 = Add(x=w2373, y=w2367) -> (x+y=w2372:dbl)
            n1609 = And(x=w2363, y=w2361) -> (x .and. y?=w2360:bool)
            n1610 = Greater?(x=w2374, y=w2372) -> (0:w2356:bool)
            n1611 = Or(x=w2356, y=w2360) -> (x .or. y?=w2353:bool)
          }
          frame False {
            n1612 = local read "Reward freq. (cm)"() -> (w2389:u32)
            n1613 = local read "Timed reward (s)"() -> (w2402:u32)
            n1614 = local read "Prev. rew. pos."() -> (w2392:dbl)
            n1615 = local read "Distance (cm)"() -> (w2393:dbl)
            n1616 = local read "Lick indicator"() -> (w2385:dbl)
            n1617 = Multiply(x=w2402, y=u32 1000) -> (x*y=w2396:u32)
            n1618 = Subtract(x=w2393, y=w2392) -> (x-y=w2387:dbl)
            n1619 = Greater?(x=w2385, y=0.1) -> (0:w2384:bool)
            n1620 = Add(x=w2389, y=u32 20) -> (x+y=w2390:u32)
            n1621 = Add(x=w2399, y=w2396) -> (x+y=w2398:u32)
            n1622 = Tick Count (ms)() -> (millisecond timer value=w2400:u32)
            n1623 = Build Array(w2389, w2390) -> (w2391:u32[])
            n1624 = Greater?(x=w2396, y=u32 999) -> (0:w2394:bool)
            n1625 = Greater?(x=w2400, y=w2398) -> (0:w2397:bool)
            n1626 = call "Analyze reward conditions.vi"("Lick event"=w2384, "Array"=w2391, "reward given"=u32 0, "mouse position"=w2387) -> ("Active rew within RZ"=w2379:bool, "Passive rew within RZ"=w2381:bool, "Passive rew after RZ"=w2376:bool)  [unwired: 4 in, 1 out]
            n1627 = And(x=w2397, y=w2394) -> (x .and. y?=w2377:bool)
            n1628 = Or(x=w2381, y=w2377) -> (x .or. y?=w2380:bool)
            n1629 = Or(x=w2379, y=w2377) -> (x .or. y?=w2378:bool)
            n1630 = Or(x=w2376, y=w2377) -> (x .or. y?=w2375:bool)
          }
        }
      }
      frame True {
        n1631 = local read "VR Mode"() -> (w2403:bool)
        n1632 = case shown="True" TRUE {
          tunnel: [FALSE ("Active rew within RZ") w2425] -> w2408
          tunnel: [w2411 w2423] -> w2407
          tunnel: [w2414 w2426] -> w2406
          tunnel: [FALSE ("Passive rew after RZ") w2424] -> w2405
          frame False {
            w2415 = 0 ("element")
            n1633 = local read "Track position"() -> (w2420:sgl)
            n1634 = local read "Reward given"() -> (w2418:u32)
            n1635 = local read "Lick indicator"() -> (w2417:dbl)
            n1636 = Greater?(x=w2417, y=0.1) -> (0:w2421:bool)
            n1637 = local read "Track position"() -> (w2410:sgl)
            n1638 = Build Array(w2415, w2415) -> (w2419:i32[])
            n1639 = call "Analyze reward conditions.vi"("Lick event"=w2421, "Array"=w2419, "reward given"=w2418, "mouse position"=w2420) -> ("Passive rew within RZ"=w2414:bool)  [unwired: 4 in, 3 out]
            n1640 = Greater?(x=w2410, y=sgl 100.0) -> (0:w2411:bool)
          }
          frame True {
            n1641 = local read "current VR context"() -> (w2432:u16)
            n1642 = local read "zeward zones"() -> (w2433:i16[][])
            n1643 = local read "Lick indicator"() -> (w2428:dbl)
            n1644 = local read "Track position"() -> (w2434:sgl)
            n1645 = local read "Reward given"() -> (w2430:u32)
            n1646 = Delete From Array(array=w2433, index (row)=w2432) -> (deleted portion=w2431:i16[])  [unwired: 2 in, 1 out]
            n1647 = Greater?(x=w2428, y=0.1) -> (0:w2427:bool)
            n1648 = local read "Track position"() -> (w2422:sgl)
            n1649 = call "Analyze reward conditions.vi"("Lick event"=w2427, "Array"=w2431, "reward given"=w2430, "mouse position"=w2434) -> ("Active rew within RZ"=w2425:bool, "Passive rew within RZ"=w2426:bool, "Passive rew after RZ"=w2424:bool)  [unwired: 4 in, 1 out]
            n1650 = call "Is New Trial - reward loop.vi"("Position data"=w2422) -> ("Boolean"=w2423:bool)  [unwired: 1 in]
          }
        }
        n1651 = local write "VR Mode"(w2403) -> ()
      }
    }
    n1652 = case shown="True" "Give reward" {
      tunnel: w2290 -> [_ w2438]
      tunnel: w2302 -> [_ w2437]
      frame False {
      }
      frame True {
        n1653 = flat-sequence {
          tunnel: w2438 -> [w2444]
          tunnel: w2437 -> [w2439]
          frame #0 {
            n1654 = local read "Water cnt. reset"() -> (w2442:i32)
            n1655 = for {
              N: w2439 -> [_]
              tunnel: w2444 -> [w2446]
              n1656 = local read "Valve open dur. (ms)"() -> (w2445:u32)
              n1657 = local write "Valve open"(TRUE ("Valve open")) -> ()
              n1658 = call "SendTriggerPulse.vi"("Trigger Duration (ms)"=w2445, "Refnum in"=w2446) -> ()  [unwired: 9 in, 1 out]
            }
            n1659 = local read "Water count"() -> (w2440:i32)
            n1660 = Add(x=w2439, y=w2442) -> (x+y=w2443:i32)
            n1661 = Add(x=w2439, y=w2440) -> (x+y=w2441:i32)
            n1662 = local write "Water cnt. reset"(w2443) -> ()
            n1663 = local write "Water count"(w2441) -> ()
          }
          frame #1 {
            n1664 = local write "Valve open"(FALSE ("Valve open")) -> ()
          }
        }
      }
    }
    n1665 = case shown="True" w2295 {
      frame False {
      }
      frame True {
        n1666 = local write "Reward given"(u32 0 ("Reward given")) -> ()
      }
    }
    n1667 = local read "Hybrid licking"() -> (w2278:bool)
    n1668 = local read "Active licking"() -> (w2280:bool)
    n1669 = Select(t=w2277, s=w2278, f=FALSE) -> (s? t:f=w2275:bool)
    n1670 = Or(x=w2275, y=w2274) -> (x .or. y?=w2273:bool)
    n1671 = Select(t=w2273, s=w2280, f=w2279) -> (s? t:f=w2272:bool)
    n1672 = case shown="True" w2272 {
      tunnel: w2300 -> [_ w2313]
      tunnel: w2290 -> [_ w2312]
      tunnel: [w2307 w2309] -> w2282
      tunnel: w2281 -> [w2307 _]
      tunnel: w2277 -> [_ w2308]
      frame False {
      }
      frame True {
        n1673 = flat-sequence {
          tunnel: w2313 -> [w2317]
          tunnel: w2312 -> [w2316]
          tunnel: [w2316] -> w2311
          tunnel: [w2315] -> w2310
          tunnel: w2308 -> [w2314]
          tunnel: w2311 -> [w2332]
          tunnel: w2310 -> [w2326]
          tunnel: [w2325] -> w2309
          frame #0 {
            n1674 = case shown="True" w2314 {
              tunnel: w2317 -> [_ w2321]
              tunnel: [1 ("Repetition") w2319] -> w2315
              frame True {
              }
              frame False {
                n1675 = local read "Sound duration (ms)"() -> (w2320:u32)
                n1676 = local read "Repetition"() -> (w2319:i32)
                n1677 = call "SendTriggerPulse.vi"("Trigger Duration (ms)"=w2320, "Refnum in"=w2321) -> ()  [unwired: 9 in, 1 out]
              }
            }
          }
          frame #1 {
            n1678 = Random Number (0-1)() -> (number: 0 to 1=w2327:dbl)
            n1679 = local read "Water cnt. reset"() -> (w2331:i32)
            n1680 = local read "Water count"() -> (w2328:i32)
            n1681 = local write "random rew"(w2327) -> ()
            n1682 = Add(x=w2326, y=w2331) -> (x+y=w2330:i32)
            n1683 = Add(x=w2326, y=w2328) -> (x+y=w2329:i32)
            n1684 = local read "Reward given"() -> (w2324:u32)
            n1685 = for {
              N: w2326 -> [_]
              tunnel: w2332 -> [w2333]
              n1686 = stacked-sequence {
                tunnel: w2333 -> [w2336 _]
                frame #0 {
                  n1687 = local read "Valve open dur. (ms)"() -> (w2334:u32)
                  n1688 = local write "Valve open"(TRUE ("Valve open")) -> ()
                  n1689 = call "SendTriggerPulse.vi"("Trigger Duration (ms)"=w2334, "Refnum in"=w2336) -> ()  [unwired: 9 in, 1 out]
                  n1690 = Wait (ms)(milliseconds to wait=w2334) -> ()  [unwired: 1 out]
                }
                frame #1 {
                  n1691 = local read "Distance (cm)"() -> (w2337:dbl)
                  n1692 = local write "Valve open"(FALSE ("Valve open")) -> ()
                  n1693 = local write "Prev. rew. pos."(w2337) -> ()
                  n1694 = Wait (ms)(milliseconds to wait=u32 50) -> ()  [unwired: 1 out]
                }
              }
            }
            n1695 = local write "Water count"(w2329) -> ()
            n1696 = local write "Water cnt. reset"(w2330) -> ()
            n1697 = Add(x=w2324, y=u32 1) -> (x+y=w2322:u32)
            n1698 = local write "Reward given"(w2322) -> ()
            n1699 = Tick Count (ms)() -> (millisecond timer value=w2325:u32)
          }
        }
      }
    }
    n1700 = Tick Count (ms)() -> (millisecond timer value=w2292:u32)
    n1701 = local write "Active licking"("Active licking") -> ()
    n1702 = Subtract(x=w2292, y=w2291) -> (x-y=→"Reward read loop rate":u32)
    n1703 = local read "Lick indicator"() -> (w2298:dbl)
    n1704 = call "Is Value Changed.vim"("value"="Open valve") -> ("changed or first call?"=w2284:bool)
    n1705 = case shown="True" w2284 {
      tunnel: w2290 -> [_ w2344]
      tunnel: "Open valve" -> [_ w2343]
      frame False {
      }
      frame True {
        n1706 = call <vilib>:"DAQmx Start Task.vi"("task/channels in"=w2344) -> ("task out"=w2346:refnum<k21>)  [unwired: 13 in, 1 out]
        n1707 = call-poly <vilib>:"DAQmx Write.vi"("task/channels in"=w2346, "data"=w2343) -> ("task out"=w2345:refnum<k21>)  [unwired: 11 in, 2 out]
        n1708 = call <vilib>:"DAQmx Stop Task.vi"("task/channels in"=w2345) -> ()  [unwired: 13 in, 2 out]
      }
    }
    n1709 = Greater?(x=w2298, y=i8 0) -> (0:→"Lick":bool)
    n1710 = case shown="True" "Hybrid licking" {
      frame False {
      }
      frame True {
        n1711 = local write "Active licking"(TRUE ("Active licking")) -> ()
      }
    }
    n1712 = local read "Valve open"() -> (→"Valve open":bool)
    n1713 = case shown="False" "Boolean" {
      tunnel: [w2341 w2342] -> w2287
      frame False {
        n1714 = local read "Water cnt. reset"() -> (w2341:i32)
      }
      frame True {
        n1715 = local read "Water count"() -> (w2342:i32)
      }
    }
    n1716 = local read "Reward size (ul)"() -> (w2289:dbl)
    n1717 = case shown="True" "Reset water count" {
      frame False {
      }
      frame True {
        n1718 = local write "Water cnt. reset"(0 ("Waret received")) -> ()
        n1719 = local write "Reset water count"(FALSE ("Reset water count")) -> ()
      }
    }
    n1720 = local read "Exit"() -> (w2306:bool)
    n1721 = Multiply(x=w2287, y=w2289) -> (x*y=→"Water received (ul)":dbl)
    n1722 = Wait (ms)(milliseconds to wait=u32 5) -> ()  [unwired: 1 out]
  }
  n1723 = case shown="True" w79 {
    frame False {
    }
    frame True {
      n1724 = local read "settings folder"() -> (w2452:path)
      n1725 = Build Path(base path=w2452, name or relative path="Laser stimulus calibration.txt") -> (appended path=w2450:path)
      n1726 = Open/Create/Replace File(file path (use dialog)=w2450, operation (0:open)=T10."open", access (0:read/write)=enum16{"read/write", "read-only", "write-only"}."read-only") -> (refnum out=w2465:refnum<file>)  [unwired: 3 in, 2 out]
      n1727 = Read from Text File(file (use dialog)=w2465) -> (refnum out=w2464:refnum<file>, text=w2466:string)  [unwired: 3 in, 2 out]
      "Laser stimulus calibration" <- w2466
      n1728 = Match Pattern(string=w2466, regular expression="Max output: ") -> (after substring=w2467:string)  [unwired: 1 in, 3 out]
      n1729 = Match Pattern(string=w2466, regular expression="Min output: ") -> (after substring=w2463:string)  [unwired: 1 in, 3 out]
      n1730 = Close File(refnum=w2464) -> ()  [unwired: 1 in, 2 out]
      n1731 = Match Pattern(string=w2467, regular expression=" V") -> (before substring=w2469:string)  [unwired: 1 in, 3 out]
      n1732 = Match Pattern(string=w2463, regular expression=" V") -> (before substring=w2468:string)  [unwired: 1 in, 3 out]
      n1733 = Fract/Exp String To Number(string=w2468) -> (number=w2456:dbl)  [unwired: 3 in, 1 out]
      n1734 = Fract/Exp String To Number(string=w2469) -> (number=w2455:dbl)  [unwired: 3 in, 1 out]
      n1735 = while {
        tunnel: w2455 -> [w2941]
        tunnel: w2456 -> [w2950]
        shift-right: [w2945] -> _
        shift-left: _ -> [w2944]
        shift-right: [w2937] -> _
        shift-left: _ -> [w2938]
        stop <- w2997 stop-if-true
        w2976 = "none" ("regular expression")
        w2955 = " %" ("regular expression")
        # "safety switch"
        # "Stop DAQ asistant first"
        n1736 = local read "Stim prot command"() -> (w2962:u16)
        n1737 = local read "protocol array"() -> (w2958:string[][])
        n1738 = Tick Count (ms)() -> (millisecond timer value=w2937:u32)
        n1739 = Subtract(x=w2937, y=w2938) -> (x-y=w2936:u32)
        n1740 = Divide(x=u32 1000, y=w2936) -> (x/y=→"stim loop rate":dbl)
        n1741 = Index Array(array=w2958, index (row)=w2962, index (col)=4) -> (element=w2960:string)
        n1742 = Index Array(array=w2958, index (row)=w2962, index (col)=3 ("disabled index (col)")) -> (element=w2971:string)
        n1743 = Index Array(array=w2958, index (row)=w2962, index (col)=0 ("index (row)")) -> (element=w2968:string)
        n1744 = Index Array(array=w2958, index (row)=w2962, index (col)=1 ("disabled index (col)")) -> (element=w2991:string)
        n1745 = Index Array(array=w2958, index (row)=w2962, index (col)=2 ("disabled index (col)")) -> (element=w2994:string)
        n1746 = Multiply(x="Stimulus cut off (s)", y=u32 1000) -> (x*y=w2932:u32)
        n1747 = Match Pattern(string=w2971, regular expression="int. ") -> (after substring=w2969:string)  [unwired: 1 in, 3 out]
        n1748 = local read "Track position"() -> (w2978:sgl)
        n1749 = Match Pattern(string=w2960, regular expression="duty cycle ") -> (after substring=w2956:string)  [unwired: 1 in, 3 out]
        n1750 = Match Pattern(string=w2968, regular expression="continuous") -> (match substring=w2965:string)  [unwired: 1 in, 3 out]
        n1751 = Match Pattern(string=w2968, regular expression="sinus") -> (match substring=w2964:string)  [unwired: 1 in, 3 out]
        n1752 = Match Pattern(string=w2968, regular expression="square") -> (match substring=w2963:string)  [unwired: 1 in, 3 out]
        n1753 = local read "Enable stim."() -> (w2974:bool)
        n1754 = Subtract(x=w2937, y=w2944) -> (x-y=w2943:u32)
        n1755 = Match Pattern(string=w2969, regular expression=w2955) -> (before substring=w2995:string)  [unwired: 1 in, 3 out]
        n1756 = Match Pattern(string=w2968, regular expression=" Hz") -> (before substring=w2957:string)  [unwired: 1 in, 3 out]
        n1757 = Match Pattern(string=w2968, regular expression=w2976) -> (match substring=w2975:string)  [unwired: 1 in, 3 out]
        n1758 = Match Pattern(string=w2991, regular expression="from ") -> (after substring=w2990:string)  [unwired: 1 in, 3 out]
        n1759 = Match Pattern(string=w2994, regular expression="to ") -> (after substring=w2992:string)  [unwired: 1 in, 3 out]
        n1760 = Match Pattern(string=w2956, regular expression=w2955) -> (before substring=w2954:string)  [unwired: 1 in, 3 out]
        n1761 = Concatenate Strings(w2965, w2964, w2963) -> (w2948:string)
        n1762 = Greater?(x=w2943, y=w2932) -> (0:w2942:bool)
        n1763 = Not(x=w2974) -> (.not. x?=w2973:bool)
        n1764 = Equal?(x=w2975, y=w2976) -> (x = y?=w2972:bool)
        n1765 = Decimal String To Number(string=w2995) -> (number=w2946:i32)  [unwired: 2 in, 1 out]
        n1766 = Decimal String To Number(string=w2954) -> (number=w2953:i32)  [unwired: 2 in, 1 out]
        n1767 = Decimal String To Number(string=w2957) -> (number=w2982:i32)  [unwired: 2 in, 1 out]
        n1768 = Decimal String To Number(string=w2990) -> (number=w2980:i32)  [unwired: 2 in, 1 out]
        n1769 = Decimal String To Number(string=w2992) -> (number=w2979:i32)  [unwired: 2 in, 1 out]
        n1770 = Or(x=w2973, y=w2972) -> (x .or. y?=w2977:bool)
        n1771 = case shown="False" w2977 {
          tunnel: w2980 -> [w3020 _]
          tunnel: w2978 -> [w2999 _]
          tunnel: w2979 -> [w3019 _]
          tunnel: w2978 -> [w3018 _]
          tunnel: w2948 -> [w3015 _]
          tunnel: [w3014 w3029] -> w2947
          tunnel: w2946 -> [w3012 _]
          tunnel: [w3010 w3030] -> w2940
          tunnel: w2942 -> [w3009 _]
          frame False {
            n1772 = Greater?(x=w3018, y=w3019) -> (0:w3008:bool)
            n1773 = Divide(x=w3012, y=100) -> (x/y=w3011:dbl)
            n1774 = Greater Or Equal?(x=w2999, y=w3020) -> (x >= y?=w3000:bool)
            n1775 = call "Is New Trial - stim. gen. loop.vi"("Position data"=w2999) -> ("Boolean"=w2998:bool)  [unwired: 1 in]
            n1776 = call "Is Value Changed.vim"("value"=w3000) -> ("changed or first call?"=w3003:bool)
            n1777 = call "Is Value Changed.vim"("value"=w3008) -> ("changed or first call?"=w3007:bool)
            n1778 = Compound Arithmetic op=OR(w3003, w2998) -> (w3002:bool)
            n1779 = And(x=w3008, y=w3007) -> (x .and. y?=w3006:bool)
            n1780 = Not(x=w3000) -> (.not. x?=w3001:bool)
            n1781 = Equal?(x=w3015, y="") -> (x = y?=w3017:bool)
            n1782 = Or(x=w3006, y=w3009) -> (x .or. y?=w3005:bool)
            n1783 = And(x=w3000, y=w3002) -> (x .and. y?=w3004:bool)
            n1784 = case shown="True" w3005 {
              frame False {
              }
              frame True {
                n1785 = local write "Stop light stim"(TRUE ("Stop light stim")) -> ()
              }
            }
            n1786 = case shown="True" w3001 {
              frame False {
              }
              frame True {
                n1787 = local write "Stop light stim"(TRUE ("Stop light stim")) -> ()
              }
            }
            n1788 = case shown="True" w3004 {
              frame False {
              }
              frame True {
                n1789 = local write "Start light stim"(TRUE ("Start light stim")) -> ()
                n1790 = local write "Stop light stim"(FALSE ("Stop light stim")) -> ()
              }
            }
            n1791 = case shown="False" w3017 {
              tunnel: w3015 -> [w3026 _]
              tunnel: [w3026 w3028] -> w3014
              tunnel: w3011 -> [w3025 _]
              tunnel: [w3025 w3027] -> w3010
              frame False {
                n1792 = local write "prev. max stim. V"(w3025) -> ()
                n1793 = local write "prev. stim. type"(w3026) -> ()
              }
              frame True {
                n1794 = local read "prev. stim. type"() -> (w3028:string)
                n1795 = local read "prev. max stim. V"() -> (w3027:dbl)
              }
            }
          }
          frame True {
            n1796 = local write "Stop light stim"(TRUE ("Stop light stim")) -> ()
            n1797 = local read "prev. max stim. V"() -> (w3030:dbl)
            n1798 = local read "prev. stim. type"() -> (w3029:string)
          }
        }
        n1799 = Subtract(x=w2941, y=w2950) -> (x-y=w2949:dbl)
        n1800 = local read "Start light stim"() -> (w2996:bool)
        n1801 = local read "Exit"() -> (w2952:bool)
        n1802 = Multiply(x=w2941, y=w2940) -> (x*y=w2939:dbl)
        n1803 = Multiply(x=w2949, y=w2940) -> (x*y=w2983:dbl)
        n1804 = case shown="True" w2952 {
          tunnel: [FALSE w3083] -> w2997
          frame False {
          }
          frame True {
            n1805 = flat-sequence {
              tunnel: [TRUE] -> w3083
              frame #0 {
                n1806 = Wait (ms)(milliseconds to wait=u32 100) -> ()  [unwired: 1 out]
              }
              frame #1 {
              }
            }
          }
        }
        n1807 = case shown="True" w2996 {
          selector: w2996 -> [w3032 w3040]
          tunnel: [w3035 w3050] -> w2951
          tunnel: w2983 -> [_ w3045]
          tunnel: w2950 -> [_ w3042]
          tunnel: w2982 -> [_ w3049]
          tunnel: w2947 -> [_ w3048]
          tunnel: w2953 -> [_ w3047]
          tunnel: [w3033 w3044] -> w2945
          tunnel: w2944 -> [_ w3044]
          tunnel: w2939 -> [_ w3043]
          frame False {
            n1808 = local read "Start mask stim"() -> (w3034:bool)
            n1809 = local write "stim started"(w3032) -> ()
            n1810 = case shown="False" w3034 {
              tunnel: [w3036 w3038] -> w3035
              frame True {
                n1811 = call "Simulate Signal77"("Offset"=0.0) -> ("DC"=w3036:dynamicdata)  [unwired: 13 in, 1 out]
              }
              frame False {
                n1812 = call "Simulate Signal8"("Offset"=0.0) -> ("DC"=w3038:dynamicdata)  [unwired: 13 in, 1 out]
              }
            }
            n1813 = Tick Count (ms)() -> (millisecond timer value=w3033:u32)
          }
          frame True {
            # "min V value"
            # "max V value"
            n1814 = local write "stim started"(w3040) -> ()
            n1815 = local read "Stop light stim"() -> (w3053:bool)
            n1816 = case shown="\"continuous\", Default" w3048 {
              tunnel: [w3056 w3063 w3070] -> w3046
              tunnel: w3045 -> [w3057 w3061 _]
              tunnel: w3049 -> [_ w3059 w3067]
              tunnel: w3047 -> [_ _ w3066]
              tunnel: w3043 -> [_ _ w3065]
              tunnel: w3042 -> [w3055 w3058 _]
              tunnel: [w3055 w3058 0.0] -> w3041
              frame "continuous", Default {
                n1817 = call "Simulate Signal78"("Offset"=w3057) -> ("Sine"=w3056:dynamicdata)  [unwired: 13 in, 1 out]
              }
              frame "sinus" {
                n1818 = Divide(x=w3061, y=2.0) -> (x/y=w3060:dbl)
                n1819 = call "Simulate Signal"("Offset"=w3060, "Frequency"=w3059, "Amplitude"=w3060) -> ("Sine"=w3063:dynamicdata)  [unwired: 11 in, 1 out]
              }
              frame "square" {
                n1820 = Divide(x=w3065, y=2.0) -> (x/y=w3068:dbl)
                n1821 = call "Simulate Signal10"("Offset"=w3068, "Duty Cycle (%)"=w3066, "Frequency"=w3067, "Amplitude"=w3068) -> ("Square"=w3070:dynamicdata)  [unwired: 10 in, 1 out]
              }
            }
            n1822 = call "Simulate Signal81"("Offset"=w3041) -> ("DC"=w3051:dynamicdata)  [unwired: 13 in, 1 out]
            n1823 = case shown="True" w3053 {
              tunnel: [w3074 w3081] -> w3054
              frame False {
                n1824 = local read "start with ramp"() -> (w3072:bool)
                n1825 = local read "start of stim"() -> (w3073:bool)
                n1826 = And(x=w3073, y=w3072) -> (x .and. y?=w3071:bool)
                n1827 = case shown="False" w3071 {
                  tunnel: [w3076 w3077] -> w3074
                  frame True {
                    n1828 = call "Simulate Signal12"() -> ("Triangle"=w3076:dynamicdata)  [unwired: 14 in, 1 out]
                    n1829 = local write "start of stim"(FALSE ("start of stim")) -> ()
                  }
                  frame False {
                    n1830 = call "Simulate Signal79"() -> ("DC"=w3077:dynamicdata)  [unwired: 14 in, 1 out]
                  }
                }
              }
              frame True {
                n1831 = call "Simulate Signal80"() -> ("Triangle"=w3081:dynamicdata)  [unwired: 14 in, 1 out]
                n1832 = local write "Stop light stim"(FALSE ("Stop light stim")) -> ()
                n1833 = local write "Start light stim"(FALSE ("Start light stim")) -> ()
                n1834 = local write "start of stim"(TRUE ("start of stim")) -> ()
              }
            }
            n1835 = Multiply(1:w3054, 2:w3046) -> (0:w3052:dynamicdata)  [unwired: 1 in, 1 out]
            n1836 = Add(1:w3051, 2:w3052) -> (0:w3050:dynamicdata)  [unwired: 1 in, 1 out]
          }
        }
        "Waveform Graph" <- w2951
        n1837 = call "DAQ Assistant"("data"=w2951, "stop (T)"=w2952) -> ()  [unwired: 16 in, 2 out]
      }
      n1838 = while {
        shift-right: [w2474] -> w2454
        shift-left: _ -> [w2476]
        shift-right: [w2473] -> w2453
        shift-left: _ -> [w2475]
        shift-right: [w2471] -> _
        shift-left: _ -> [w2470]
        stop <- w2472 stop-if-true
        n1839 = case shown="\"20 Hz until reward \"" w2470 {
          selector: w2470 -> [_ w2553 w2588 w2647 w2708 w2736 w2808 w2873]
          tunnel: w2476 -> [w2479 w2557 w2592 w2657 w2718 w2734 w2806 w2884]
          tunnel: w2475 -> [w2477 w2556 w2591 w2656 w2717 w2733 w2805 w2883]
          tunnel: [w2480 w2555 w2590 w2653 w2714 w2732 w2804 w2880] -> w2474
          tunnel: [w2478 w2554 w2589 w2652 w2713 w2731 w2803 w2879] -> w2473
          tunnel: [w2481 w2550 w2585 w2646 w2707 w2735 w2807 w2874] -> w2471
          frame "None", Default {
            n1840 = local read "Primary masking light"() -> (w2481:T3)
            n1841 = case shown="\"Continuous specified light off trials\"" w2481 {
              tunnel: [w2484 w2486 w2499 w2512 w2525 w2538 w2541 w2544] -> w2480
              tunnel: w2479 -> [w2484 w2488 w2501 w2514 w2527 _ _ _]
              tunnel: [w2483 w2485 w2498 w2511 w2524 w2537 w2540 w2543] -> w2478
              tunnel: w2477 -> [w2483 w2487 w2500 w2513 w2526 _ _ _]
              frame "None", Default {
              }
              frame "20 Hz until reward " {
                w2492 = 10123 items=["Finite Samples"=10178, "Continuous Samples"=10123, "Hardware Timed Single Point"=12522]  # Sample Mode
                n1842 = call <vilib>:"DAQmx Clear Task.vi"("task in"=w2488, "error in"=w2487) -> ()  [unwired: 13 in, 1 out]
                n1843 = call-poly <vilib>:"DAQmx Create Virtual Channel.vi"("frequency"=20.0, "duty cycle"=0.5 ("Duty Cycle"), "counter"=tag "Dev1/ctr3" ("Counter")) -> ("task out"=w2497:refnum<k21>, "error out"=w2496:errorcluster)  [unwired: 11 in]
                n1844 = property class="DAQmx Channel"(reference=w2497, error in=w2496, "CO.Pulse.Term"=tag "/Dev1/PFI15" ("Output Terminal")) -> (reference out=w2494:refnum<k21>, error out=w2495:errorcluster)
                n1845 = call-poly <vilib>:"DAQmx Timing.vi"("task/channels in"=w2494, "sample mode"=w2492, "error in"=w2495) -> ("task out"=w2486:refnum<k21>, "error out"=w2485:errorcluster)  [unwired: 11 in]
              }
              frame "20 Hz specified light off trials" {
                w2505 = 10123 items=["Finite Samples"=10178, "Continuous Samples"=10123, "Hardware Timed Single Point"=12522]  # Sample Mode
                n1846 = call <vilib>:"DAQmx Clear Task.vi"("task in"=w2501, "error in"=w2500) -> ()  [unwired: 13 in, 1 out]
                n1847 = call-poly <vilib>:"DAQmx Create Virtual Channel.vi"("frequency"=20.0, "duty cycle"=0.5 ("Duty Cycle"), "counter"=tag "Dev1/ctr3" ("Counter")) -> ("task out"=w2510:refnum<k21>, "error out"=w2509:errorcluster)  [unwired: 11 in]
                n1848 = property class="DAQmx Channel"(reference=w2510, error in=w2509, "CO.Pulse.Term"=tag "/Dev1/PFI15" ("Output Terminal")) -> (reference out=w2507:refnum<k21>, error out=w2508:errorcluster)
                n1849 = call-poly <vilib>:"DAQmx Timing.vi"("task/channels in"=w2507, "sample mode"=w2505, "error in"=w2508) -> ("task out"=w2499:refnum<k21>, "error out"=w2498:errorcluster)  [unwired: 11 in]
              }
              frame "20 Hz specified all trials" {
                w2518 = 10123 items=["Finite Samples"=10178, "Continuous Samples"=10123, "Hardware Timed Single Point"=12522]  # Sample Mode
                n1850 = call <vilib>:"DAQmx Clear Task.vi"("task in"=w2514, "error in"=w2513) -> ()  [unwired: 13 in, 1 out]
                n1851 = call-poly <vilib>:"DAQmx Create Virtual Channel.vi"("frequency"=20.0, "duty cycle"=0.5 ("Duty Cycle"), "counter"=tag "Dev1/ctr3" ("Counter")) -> ("task out"=w2523:refnum<k21>, "error out"=w2522:errorcluster)  [unwired: 11 in]
                n1852 = property class="DAQmx Channel"(reference=w2523, error in=w2522, "CO.Pulse.Term"=tag "/Dev1/PFI15" ("Output Terminal")) -> (reference out=w2520:refnum<k21>, error out=w2521:errorcluster)
                n1853 = call-poly <vilib>:"DAQmx Timing.vi"("task/channels in"=w2520, "sample mode"=w2518, "error in"=w2521) -> ("task out"=w2512:refnum<k21>, "error out"=w2511:errorcluster)  [unwired: 11 in]
              }
              frame "20 Hz full trial" {
                w2531 = 10123 items=["Finite Samples"=10178, "Continuous Samples"=10123, "Hardware Timed Single Point"=12522]  # Sample Mode
                n1854 = call <vilib>:"DAQmx Clear Task.vi"("task in"=w2527, "error in"=w2526) -> ()  [unwired: 13 in, 1 out]
                n1855 = call-poly <vilib>:"DAQmx Create Virtual Channel.vi"("frequency"=20.0, "duty cycle"=0.5 ("Duty Cycle"), "counter"=tag "Dev1/ctr3" ("Counter")) -> ("task out"=w2536:refnum<k21>, "error out"=w2535:errorcluster)  [unwired: 11 in]
                n1856 = property class="DAQmx Channel"(reference=w2536, error in=w2535, "CO.Pulse.Term"=tag "/Dev1/PFI15" ("Output Terminal")) -> (reference out=w2533:refnum<k21>, error out=w2534:errorcluster)
                n1857 = call-poly <vilib>:"DAQmx Timing.vi"("task/channels in"=w2533, "sample mode"=w2531, "error in"=w2534) -> ("task out"=w2525:refnum<k21>, "error out"=w2524:errorcluster)  [unwired: 11 in]
              }
              frame "Continuous specified light off trials" {
                n1858 = call-poly <vilib>:"DAQmx Create Virtual Channel.vi"("lines"=tag "Dev1/port2/line7") -> ("task out"=w2538:refnum<k21>, "error out"=w2537:errorcluster)  [unwired: 13 in]
              }
              frame "Continuous specified all trials" {
                n1859 = call-poly <vilib>:"DAQmx Create Virtual Channel.vi"("lines"=tag "Dev1/port2/line7") -> ("task out"=w2541:refnum<k21>, "error out"=w2540:errorcluster)  [unwired: 13 in]
              }
              frame "Continuous full trial" {
                n1860 = call-poly <vilib>:"DAQmx Create Virtual Channel.vi"("lines"=tag "Dev1/port2/line7") -> ("task out"=w2544:refnum<k21>, "error out"=w2543:errorcluster)  [unwired: 13 in]
              }
            }
            n1861 = Wait (ms)(milliseconds to wait=u32 20) -> ()  [unwired: 1 out]
          }
          frame "20 Hz until reward " {
            n1862 = local read "Reward given"() -> (w2548:u32)
            n1863 = Equal?(x=w2548, y=u32 0) -> (x = y?=w2546:bool)
            n1864 = case shown="True" w2546 {
              tunnel: w2557 -> [w2560 w2566]
              tunnel: w2556 -> [w2559 w2568]
              tunnel: [w2560 w2561] -> w2555
              tunnel: [w2559 w2562] -> w2554
              frame False {
                n1865 = Wait (ms)(milliseconds to wait=u32 20) -> ()  [unwired: 1 out]
              }
              frame True {
                n1866 = call <vilib>:"DAQmx Start Task.vi"("task/channels in"=w2566, "error in"=w2568) -> ("task out"=w2565:refnum<k21>, "error out"=w2567:errorcluster)  [unwired: 12 in]
                n1867 = while {
                  tunnel: w2565 -> [w2582]
                  tunnel: w2567 -> [w2581]
                  tunnel: [w2579] -> w2563
                  tunnel: [w2580] -> w2564
                  stop <- w2577 stop-if-true
                  n1868 = local read "Reward given"() -> (w2571:u32)
                  n1869 = local read "Primary masking light"() -> (w2574:T3)
                  n1870 = call <vilib>:"DAQmx Is Task Done.vi"("task/channels in"=w2582, "error in"=w2581) -> ("task out"=w2580:refnum<k21>, "error out"=w2579:errorcluster)  [unwired: 11 in, 1 out]
                  n1871 = local read "Exit"() -> (w2576:bool)
                  n1872 = Unbundle By Name(w2579) -> ("status"=w2575:bool)
                  n1873 = Greater?(x=w2571, y=u32 0) -> (0:w2569:bool)
                  n1874 = Not Equal?(x=w2574, y=T13."20 Hz until reward ") -> (x != y?=w2570:bool)
                  n1875 = Wait (ms)(milliseconds to wait=u32 20) -> ()  [unwired: 1 out]
                  n1876 = Compound Arithmetic op=OR(w2575, w2576, w2569, w2570) -> (w2577:bool)
                }
                n1877 = call <vilib>:"DAQmx Stop Task.vi"("task/channels in"=w2564, "error in"=w2563) -> ("task out"=w2561:refnum<k21>, "error out"=w2562:errorcluster)  [unwired: 12 in]
              }
            }
            n1878 = local read "Primary masking light"() -> (w2551:T3)
            n1879 = Equal?(x=w2551, y=w2553) -> (x = y?=w2552:bool)
            n1880 = Select(t=w2551, s=w2552, f=T13."None") -> (s? t:f=w2550:T3)
          }
          frame "20 Hz full trial" {
            n1881 = local read "Run experiment"() -> (w2583:bool)
            n1882 = case shown="True" w2583 {
              tunnel: w2592 -> [w2595 w2601]
              tunnel: w2591 -> [w2594 w2603]
              tunnel: [w2595 w2596] -> w2590
              tunnel: [w2594 w2597] -> w2589
              frame False {
                n1883 = Wait (ms)(milliseconds to wait=u32 20) -> ()  [unwired: 1 out]
              }
              frame True {
                n1884 = call <vilib>:"DAQmx Start Task.vi"("task/channels in"=w2601, "error in"=w2603) -> ("task out"=w2600:refnum<k21>, "error out"=w2602:errorcluster)  [unwired: 12 in]
                n1885 = while {
                  tunnel: w2600 -> [w2612]
                  tunnel: w2602 -> [w2611]
                  tunnel: [w2622] -> w2598
                  tunnel: [w2623] -> w2599
                  stop <- w2620 stop-if-true
                  n1886 = local read "stim started"() -> (w2607:bool)
                  n1887 = Equal?(x=w2607, y=TRUE) -> (x = y?=w2605:bool)
                  n1888 = call "Is Value Changed.vim"("value"=w2607) -> ("changed or first call?"=w2606:bool)
                  n1889 = And(x=w2606, y=w2605) -> (x .and. y?=w2604:bool)
                  n1890 = case shown="True" w2604 {
                    tunnel: w2612 -> [w2625 w2632]
                    tunnel: w2611 -> [w2624 w2633]
                    tunnel: [w2625 w2627] -> w2610
                    tunnel: [w2624 w2626] -> w2609
                    frame False {
                    }
                    frame True {
                      n1891 = flat-sequence {
                        tunnel: w2633 -> [w2635]
                        tunnel: w2632 -> [w2634]
                        tunnel: [w2637] -> w2631
                        tunnel: [w2636] -> w2630
                        tunnel: w2631 -> [w2640]
                        tunnel: w2630 -> [w2639]
                        tunnel: [w2640] -> w2629
                        tunnel: [w2639] -> w2628
                        tunnel: w2629 -> [w2642]
                        tunnel: w2628 -> [w2641]
                        tunnel: [w2644] -> w2627
                        tunnel: [w2643] -> w2626
                        frame #0 {
                          n1892 = call <vilib>:"DAQmx Stop Task.vi"("task/channels in"=w2634, "error in"=w2635) -> ("task out"=w2637:refnum<k21>, "error out"=w2636:errorcluster)  [unwired: 12 in]
                        }
                        frame #1 {
                          n1893 = Wait (ms)(milliseconds to wait=u32 5) -> ()  [unwired: 1 out]
                        }
                        frame #2 {
                          n1894 = call <vilib>:"DAQmx Start Task.vi"("task/channels in"=w2642, "error in"=w2641) -> ("task out"=w2644:refnum<k21>, "error out"=w2643:errorcluster)  [unwired: 12 in]
                        }
                      }
                    }
                  }
                  n1895 = local read "Primary masking light"() -> (w2616:T3)
                  n1896 = local read "Run experiment"() -> (w2615:bool)
                  n1897 = call <vilib>:"DAQmx Is Task Done.vi"("task/channels in"=w2610, "error in"=w2609) -> ("task out"=w2623:refnum<k21>, "error out"=w2622:errorcluster)  [unwired: 11 in, 1 out]
                  n1898 = local read "Exit"() -> (w2619:bool)
                  n1899 = Unbundle By Name(w2622) -> ("status"=w2618:bool)
                  n1900 = Not(x=w2615) -> (.not. x?=w2614:bool)
                  n1901 = Not Equal?(x=w2616, y=T3."20 Hz full trial") -> (x != y?=w2617:bool)
                  n1902 = Wait (ms)(milliseconds to wait=u32 2) -> ()  [unwired: 1 out]
                  n1903 = Compound Arithmetic op=OR(w2618, w2619, w2614, w2617) -> (w2620:bool)
                }
                n1904 = call <vilib>:"DAQmx Stop Task.vi"("task/channels in"=w2599, "error in"=w2598) -> ("task out"=w2596:refnum<k21>, "error out"=w2597:errorcluster)  [unwired: 12 in]
              }
            }
            n1905 = local read "Primary masking light"() -> (w2586:T3)
            n1906 = Equal?(x=w2586, y=w2588) -> (x = y?=w2587:bool)
            n1907 = Select(t=w2586, s=w2587, f=T13."None") -> (s? t:f=w2585:T3)
          }
          frame "Continuous specified light off trials" {
            n1908 = call <vilib>:"DAQmx Start Task.vi"("task/channels in"=w2657, "error in"=w2656) -> ("task out"=w2655:refnum<k21>, "error out"=w2654:errorcluster)  [unwired: 12 in]
            n1909 = disable-structure shown="Disabled" {
              disable-tunnel: w2655 -> [w2661 _]
              disable-tunnel: w2654 -> [w2660 _]
              disable-tunnel: [w2659 _] -> w2651
              disable-tunnel: [w2658 _] -> w2650
              frame Disabled {
                n1910 = while {
                  tunnel: w2661 -> [w2674]
                  tunnel: w2660 -> [w2673]
                  tunnel: [w2672] -> w2658
                  tunnel: [w2671] -> w2659
                  stop <- w2666 stop-if-true
                  n1911 = local read "VR Mode"() -> (w2668:bool)
                  n1912 = case shown="True" w2668 {
                    tunnel: [w2677 w2695] -> w2669
                    frame False {
                      n1913 = local read "prev. diode position"() -> (w2675:dbl)
                      n1914 = local read "total distance cm"() -> (w2686:sgl[])
                      n1915 = local read "total distance cm"() -> (w2687:sgl[])
                      n1916 = local read "prev. diode position"() -> (w2676:dbl)
                      n1917 = local read item#-1() -> ()  [unwired: 1 out]
                      n1918 = local read item#-1() -> ()  [unwired: 1 out]
                      n1919 = Subtract() -> (x-y=w2682:dbl)  [unwired: 2 in]
                      n1920 = Divide(x=w2682, y=2.0) -> (x/y=w2680:dbl)
                      n1921 = Absolute Value(x=w2680) -> (abs(x)=w2679:dbl)
                      n1922 = Add(y=w2679) -> (x+y=w2678:dbl)  [unwired: 1 in]
                      n1923 = Array Max & Min(array=w2686) -> (max value=w2685:sgl)  [unwired: 3 out]
                      n1924 = Array Max & Min(array=w2687) -> (max value=w2688:sgl)  [unwired: 3 out]
                      n1925 = Subtract(x=w2685, y=w2675) -> (x-y=w2684:dbl)
                      n1926 = Subtract(x=w2688, y=w2676) -> (x-y=w2689:dbl)
                      n1927 = Greater?(x=w2684) -> (0:w2683:bool)  [unwired: 1 in]
                      n1928 = case shown="True" w2683 {
                        frame False {
                        }
                        frame True {
                          n1929 = local write "Masking light"(FALSE ("Masking light")) -> ()
                        }
                      }
                      n1930 = Greater?(x=w2689) -> (0:w2691:bool)  [unwired: 1 in]
                      n1931 = Less?(x=w2689, y=w2678) -> (x < y?=w2690:bool)
                      n1932 = And(x=w2690, y=w2691) -> (x .and. y?=w2677:bool)
                    }
                    frame True {
                      n1933 = local read "Track position"() -> (w2700:sgl)
                      n1934 = local read "Track position"() -> (w2701:sgl)
                      n1935 = local read "Track position"() -> (w2697:sgl)
                      n1936 = local read item#-1() -> ()  [unwired: 1 out]
                      n1937 = local read item#-1() -> ()  [unwired: 1 out]
                      n1938 = local read item#-1() -> ()  [unwired: 1 out]
                      n1939 = Add(y=15.0) -> (x+y=w2693:dbl)  [unwired: 1 in]
                      n1940 = Less?(x=w2701, y=w2693) -> (x < y?=w2698:bool)
                      n1941 = Greater?(x=w2697) -> (0:w2696:bool)  [unwired: 1 in]
                      n1942 = Greater?(x=w2700) -> (0:w2699:bool)  [unwired: 1 in]
                      n1943 = case shown="True" w2699 {
                        frame False {
                        }
                        frame True {
                          n1944 = local write "Masking light"(FALSE ("Masking light")) -> ()
                        }
                      }
                      n1945 = And(x=w2698, y=w2696) -> (x .and. y?=w2695:bool)
                    }
                  }
                  n1946 = Wait (ms)(milliseconds to wait=u32 10) -> ()  [unwired: 1 out]
                  n1947 = local read "Primary masking light"() -> (w2664:T3)
                  n1948 = case shown="True" w2669 {
                    frame False {
                    }
                    frame True {
                      n1949 = local read "Light ON"() -> (w2704:bool)
                      n1950 = Not(x=w2704) -> (.not. x?=w2703:bool)
                      n1951 = case shown="True" w2703 {
                        frame False {
                        }
                        frame True {
                          n1952 = local write "Masking light"(TRUE ("Masking light")) -> ()
                        }
                      }
                    }
                  }
                  n1953 = local read "Masking light"() -> (w2667:bool)
                  n1954 = Not Equal?(x=w2664, y=T13."Continuous specified light off trials") -> (x != y?=w2663:bool)
                  n1955 = local read "Exit"() -> (w2665:bool)
                  n1956 = call-poly <vilib>:"DAQmx Write.vi"("task/channels in"=w2674, "data"=w2667, "error in"=w2673) -> ("task out"=w2672:refnum<k21>, "error out"=w2671:errorcluster)  [unwired: 10 in, 1 out]
                  n1957 = Compound Arithmetic op=OR(w2663, w2665) -> (w2666:bool)
                }
              }
              frame Enabled {
              }
            }
            n1958 = local read "Primary masking light"() -> (w2648:T3)
            n1959 = Equal?(x=w2648, y=w2647) -> (x = y?=w2649:bool)
            n1960 = Select(t=w2648, s=w2649, f=T13."None") -> (s? t:f=w2646:T3)
            n1961 = call <vilib>:"DAQmx Stop Task.vi"("task/channels in"=w2650, "error in"=w2651) -> ("task out"=w2653:refnum<k21>, "error out"=w2652:errorcluster)  [unwired: 12 in]
          }
          frame "Continuous full trial" {
            n1962 = call <vilib>:"DAQmx Start Task.vi"("task/channels in"=w2718, "error in"=w2717) -> ("task out"=w2716:refnum<k21>, "error out"=w2715:errorcluster)  [unwired: 12 in]
            n1963 = while {
              tunnel: w2716 -> [w2729]
              tunnel: w2715 -> [w2728]
              tunnel: [w2727] -> w2711
              tunnel: [w2726] -> w2712
              stop <- w2724 stop-if-true
              n1964 = Wait (ms)(milliseconds to wait=u32 10) -> ()  [unwired: 1 out]
              n1965 = local read "Primary masking light"() -> (w2722:T3)
              n1966 = local read "Run experiment"() -> (w2720:bool)
              n1967 = Not Equal?(x=w2722, y=T3."Continuous full trial") -> (x != y?=w2721:bool)
              n1968 = local read "Exit"() -> (w2723:bool)
              n1969 = call-poly <vilib>:"DAQmx Write.vi"("task/channels in"=w2729, "data"=w2720, "error in"=w2728) -> ("task out"=w2727:refnum<k21>, "error out"=w2726:errorcluster)  [unwired: 10 in, 1 out]
              n1970 = Compound Arithmetic op=OR(w2721, w2723) -> (w2724:bool)
            }
            n1971 = local read "Primary masking light"() -> (w2709:T3)
            n1972 = Equal?(x=w2709, y=w2708) -> (x = y?=w2710:bool)
            n1973 = Select(t=w2709, s=w2710, f=T13."None") -> (s? t:f=w2707:T3)
            n1974 = call <vilib>:"DAQmx Stop Task.vi"("task/channels in"=w2711, "error in"=w2712) -> ("task out"=w2714:refnum<k21>, "error out"=w2713:errorcluster)  [unwired: 12 in]
          }
          frame "20 Hz specified light off trials" {
            n1975 = disable-structure shown="Disabled" {
              disable-tunnel: w2734 -> [w2743 _]
              disable-tunnel: w2733 -> [w2742 _]
              disable-tunnel: [w2741 _] -> w2732
              disable-tunnel: [w2740 _] -> w2731
              frame Disabled {
                n1976 = local read "VR Mode"() -> (w2744:bool)
                n1977 = case shown="True" w2744 {
                  tunnel: [w2746 w2760] -> w2745
                  frame False {
                    n1978 = local read "total distance cm"() -> (w2752:sgl[])
                    n1979 = local read "prev. diode position"() -> (w2753:dbl)
                    n1980 = local read item#-1() -> ()  [unwired: 1 out]
                    n1981 = Subtract() -> (x-y=w2751:dbl)  [unwired: 2 in]
                    n1982 = Divide(x=w2751, y=2.0) -> (x/y=w2749:dbl)
                    n1983 = Absolute Value(x=w2749) -> (abs(x)=w2748:dbl)
                    n1984 = local read item#-1() -> ()  [unwired: 1 out]
                    n1985 = Add(y=w2748) -> (x+y=w2747:dbl)  [unwired: 1 in]
                    n1986 = Array Max & Min(array=w2752) -> (max value=w2754:sgl)  [unwired: 3 out]
                    n1987 = Subtract(x=w2754, y=w2753) -> (x-y=w2755:dbl)
                    n1988 = Greater?(x=w2755) -> (0:w2757:bool)  [unwired: 1 in]
                    n1989 = Less?(x=w2755, y=w2747) -> (x < y?=w2756:bool)
                    n1990 = And(x=w2756, y=w2757) -> (x .and. y?=w2746:bool)
                  }
                  frame True {
                    n1991 = local read "Track position"() -> (w2764:sgl)
                    n1992 = local read "Track position"() -> (w2762:sgl)
                    n1993 = local read item#-1() -> ()  [unwired: 1 out]
                    n1994 = local read item#-1() -> ()  [unwired: 1 out]
                    n1995 = Add(y=15.0) -> (x+y=w2758:dbl)  [unwired: 1 in]
                    n1996 = Less?(x=w2764, y=w2758) -> (x < y?=w2763:bool)
                    n1997 = Greater?(x=w2762) -> (0:w2761:bool)  [unwired: 1 in]
                    n1998 = And(x=w2763, y=w2761) -> (x .and. y?=w2760:bool)
                  }
                }
                n1999 = case shown="True" w2745 {
                  frame False {
                  }
                  frame True {
                    n2000 = local read "Light ON"() -> (w2766:bool)
                    n2001 = Not(x=w2766) -> (.not. x?=w2765:bool)
                    n2002 = case shown="True" w2765 {
                      frame False {
                      }
                      frame True {
                        n2003 = local write "Masking light"(TRUE ("Masking light")) -> ()
                      }
                    }
                  }
                }
                n2004 = local read "Masking light"() -> (w2739:bool)
                n2005 = case shown="True" w2739 {
                  tunnel: w2743 -> [w2770 w2776]
                  tunnel: w2742 -> [w2769 w2778]
                  tunnel: [w2770 w2771] -> w2741
                  tunnel: [w2769 w2772] -> w2740
                  frame False {
                    n2006 = Wait (ms)(milliseconds to wait=u32 20) -> ()  [unwired: 1 out]
                  }
                  frame True {
                    n2007 = call <vilib>:"DAQmx Start Task.vi"("task/channels in"=w2776, "error in"=w2778) -> ("task out"=w2775:refnum<k21>, "error out"=w2777:errorcluster)  [unwired: 12 in]
                    n2008 = while {
                      tunnel: w2775 -> [w2792]
                      tunnel: w2777 -> [w2791]
                      tunnel: [w2789] -> w2773
                      tunnel: [w2790] -> w2774
                      stop <- w2787 stop-if-true
                      n2009 = local read "VR Mode"() -> (w2779:bool)
                      n2010 = case shown="True" w2779 {
                        frame False {
                          n2011 = local read "prev. diode position"() -> (w2793:dbl)
                          n2012 = local read "total distance cm"() -> (w2797:sgl[])
                          n2013 = local read item#-1() -> ()  [unwired: 1 out]
                          n2014 = Array Max & Min(array=w2797) -> (max value=w2796:sgl)  [unwired: 3 out]
                          n2015 = Subtract(x=w2796, y=w2793) -> (x-y=w2795:dbl)
                          n2016 = Greater?(x=w2795) -> (0:w2794:bool)  [unwired: 1 in]
                          n2017 = case shown="True" w2794 {
                            frame False {
                            }
                            frame True {
                              n2018 = local write "Masking light"(FALSE ("Masking light")) -> ()
                            }
                          }
                        }
                        frame True {
                          n2019 = local read "Track position"() -> (w2800:sgl)
                          n2020 = local read item#-1() -> ()  [unwired: 1 out]
                          n2021 = Greater?(x=w2800) -> (0:w2799:bool)  [unwired: 1 in]
                          n2022 = case shown="True" w2799 {
                            frame False {
                            }
                            frame True {
                              n2023 = local write "Masking light"(FALSE ("Masking light")) -> ()
                            }
                          }
                        }
                      }
                      n2024 = local read "Primary masking light"() -> (w2783:T3)
                      n2025 = call <vilib>:"DAQmx Is Task Done.vi"("task/channels in"=w2792, "error in"=w2791) -> ("task out"=w2790:refnum<k21>, "error out"=w2789:errorcluster)  [unwired: 11 in, 1 out]
                      n2026 = local read "Masking light"() -> (w2781:bool)
                      n2027 = Unbundle By Name(w2789) -> ("status"=w2785:bool)
                      n2028 = local read "Exit"() -> (w2786:bool)
                      n2029 = Not(x=w2781) -> (.not. x?=w2780:bool)
                      n2030 = Not Equal?(x=w2783, y=T13."20 Hz specified light off trials") -> (x != y?=w2784:bool)
                      n2031 = Compound Arithmetic op=OR(w2785, w2786, w2780, w2784) -> (w2787:bool)
                      n2032 = Wait (ms)(milliseconds to wait=u32 20) -> ()  [unwired: 1 out]
                    }
                    n2033 = call <vilib>:"DAQmx Stop Task.vi"("task/channels in"=w2774, "error in"=w2773) -> ("task out"=w2771:refnum<k21>, "error out"=w2772:errorcluster)  [unwired: 12 in]
                  }
                }
              }
              frame Enabled {
              }
            }
            n2034 = local read "Primary masking light"() -> (w2737:T3)
            n2035 = Equal?(x=w2737, y=w2736) -> (x = y?=w2738:bool)
            n2036 = Select(t=w2737, s=w2738, f=T13."None") -> (s? t:f=w2735:T3)
          }
          frame "20 Hz specified all trials" {
            n2037 = disable-structure shown="Disabled" {
              disable-tunnel: w2806 -> [w2815 _]
              disable-tunnel: w2805 -> [w2814 _]
              disable-tunnel: [w2813 _] -> w2804
              disable-tunnel: [w2812 _] -> w2803
              frame Disabled {
                n2038 = local read "VR Mode"() -> (w2816:bool)
                n2039 = case shown="True" w2816 {
                  tunnel: [w2819 w2832] -> w2817
                  frame False {
                    n2040 = local read "total distance cm"() -> (w2825:sgl[])
                    n2041 = local read "prev. diode position"() -> (w2818:dbl)
                    n2042 = local read item#-1() -> ()  [unwired: 1 out]
                    n2043 = Subtract() -> (x-y=w2824:dbl)  [unwired: 2 in]
                    n2044 = Divide(x=w2824, y=2.0) -> (x/y=w2822:dbl)
                    n2045 = Absolute Value(x=w2822) -> (abs(x)=w2821:dbl)
                    n2046 = local read item#-1() -> ()  [unwired: 1 out]
                    n2047 = Add(y=w2821) -> (x+y=w2820:dbl)  [unwired: 1 in]
                    n2048 = Array Max & Min(array=w2825) -> (max value=w2826:sgl)  [unwired: 3 out]
                    n2049 = Subtract(x=w2826, y=w2818) -> (x-y=w2827:dbl)
                    n2050 = Greater?(x=w2827) -> (0:w2829:bool)  [unwired: 1 in]
                    n2051 = Less?(x=w2827, y=w2820) -> (x < y?=w2828:bool)
                    n2052 = And(x=w2828, y=w2829) -> (x .and. y?=w2819:bool)
                  }
                  frame True {
                    n2053 = local read "Track position"() -> (w2836:sgl)
                    n2054 = local read "Track position"() -> (w2834:sgl)
                    n2055 = local read item#-1() -> ()  [unwired: 1 out]
                    n2056 = local read item#-1() -> ()  [unwired: 1 out]
                    n2057 = Add(y=15.0) -> (x+y=w2830:dbl)  [unwired: 1 in]
                    n2058 = Less?(x=w2836, y=w2830) -> (x < y?=w2835:bool)
                    n2059 = Greater?(x=w2834) -> (0:w2833:bool)  [unwired: 1 in]
                    n2060 = And(x=w2835, y=w2833) -> (x .and. y?=w2832:bool)
                  }
                }
                n2061 = case shown="True" w2817 {
                  frame False {
                  }
                  frame True {
                    n2062 = local write "Masking light"(TRUE ("Masking light")) -> ()
                  }
                }
                n2063 = local read "Masking light"() -> (w2811:bool)
                n2064 = case shown="True" w2811 {
                  tunnel: w2815 -> [w2840 w2846]
                  tunnel: w2814 -> [w2839 w2848]
                  tunnel: [w2840 w2841] -> w2813
                  tunnel: [w2839 w2842] -> w2812
                  frame False {
                    n2065 = Wait (ms)(milliseconds to wait=u32 20) -> ()  [unwired: 1 out]
                  }
                  frame True {
                    n2066 = call <vilib>:"DAQmx Start Task.vi"("task/channels in"=w2846, "error in"=w2848) -> ("task out"=w2845:refnum<k21>, "error out"=w2847:errorcluster)  [unwired: 12 in]
                    n2067 = while {
                      tunnel: w2845 -> [w2862]
                      tunnel: w2847 -> [w2861]
                      tunnel: [w2859] -> w2843
                      tunnel: [w2860] -> w2844
                      stop <- w2857 stop-if-true
                      n2068 = local read "VR Mode"() -> (w2849:bool)
                      n2069 = case shown="True" w2849 {
                        frame False {
                          n2070 = local read "prev. diode position"() -> (w2863:dbl)
                          n2071 = local read "total distance cm"() -> (w2867:sgl[])
                          n2072 = local read item#-1() -> ()  [unwired: 1 out]
                          n2073 = Array Max & Min(array=w2867) -> (max value=w2866:sgl)  [unwired: 3 out]
                          n2074 = Subtract(x=w2866, y=w2863) -> (x-y=w2865:dbl)
                          n2075 = Greater?(x=w2865) -> (0:w2864:bool)  [unwired: 1 in]
                          n2076 = case shown="True" w2864 {
                            frame False {
                            }
                            frame True {
                              n2077 = local write "Masking light"(FALSE ("Masking light")) -> ()
                            }
                          }
                        }
                        frame True {
                          n2078 = local read "Track position"() -> (w2870:sgl)
                          n2079 = local read item#-1() -> ()  [unwired: 1 out]
                          n2080 = Greater?(x=w2870) -> (0:w2869:bool)  [unwired: 1 in]
                          n2081 = case shown="True" w2869 {
                            frame False {
                            }
                            frame True {
                              n2082 = local write "Masking light"(FALSE ("Masking light")) -> ()
                            }
                          }
                        }
                      }
                      n2083 = local read "Primary masking light"() -> (w2853:T3)
                      n2084 = call <vilib>:"DAQmx Is Task Done.vi"("task/channels in"=w2862, "error in"=w2861) -> ("task out"=w2860:refnum<k21>, "error out"=w2859:errorcluster)  [unwired: 11 in, 1 out]
                      n2085 = local read "Masking light"() -> (w2851:bool)
                      n2086 = Unbundle By Name(w2859) -> ("status"=w2855:bool)
                      n2087 = local read "Exit"() -> (w2856:bool)
                      n2088 = Not(x=w2851) -> (.not. x?=w2850:bool)
                      n2089 = Not Equal?(x=w2853, y=T13."20 Hz specified all trials") -> (x != y?=w2854:bool)
                      n2090 = Compound Arithmetic op=OR(w2855, w2856, w2850, w2854) -> (w2857:bool)
                      n2091 = Wait (ms)(milliseconds to wait=u32 20) -> ()  [unwired: 1 out]
                    }
                    n2092 = call <vilib>:"DAQmx Stop Task.vi"("task/channels in"=w2844, "error in"=w2843) -> ("task out"=w2841:refnum<k21>, "error out"=w2842:errorcluster)  [unwired: 12 in]
                  }
                }
              }
              frame Enabled {
              }
            }
            n2093 = local read "Primary masking light"() -> (w2809:T3)
            n2094 = Equal?(x=w2809, y=w2808) -> (x = y?=w2810:bool)
            n2095 = Select(t=w2809, s=w2810, f=T13."None") -> (s? t:f=w2807:T3)
          }
          frame "Continuous specified all trials" {
            n2096 = call <vilib>:"DAQmx Start Task.vi"("task/channels in"=w2884, "error in"=w2883) -> ("task out"=w2882:refnum<k21>, "error out"=w2881:errorcluster)  [unwired: 12 in]
            n2097 = disable-structure shown="Disabled" {
              disable-tunnel: w2882 -> [w2888 _]
              disable-tunnel: w2881 -> [w2887 _]
              disable-tunnel: [w2886 _] -> w2878
              disable-tunnel: [w2885 _] -> w2877
              frame Disabled {
                n2098 = while {
                  tunnel: w2888 -> [w2901]
                  tunnel: w2887 -> [w2900]
                  tunnel: [w2899] -> w2885
                  tunnel: [w2898] -> w2886
                  stop <- w2890 stop-if-true
                  n2099 = local read "VR Mode"() -> (w2895:bool)
                  n2100 = case shown="True" w2895 {
                    tunnel: [w2904 w2922] -> w2896
                    frame False {
                      n2101 = local read "prev. diode position"() -> (w2902:dbl)
                      n2102 = local read "total distance cm"() -> (w2913:sgl[])
                      n2103 = local read "total distance cm"() -> (w2914:sgl[])
                      n2104 = local read item#-1() -> ()  [unwired: 1 out]
                      n2105 = local read "prev. diode position"() -> (w2903:dbl)
                      n2106 = local read item#-1() -> ()  [unwired: 1 out]
                      n2107 = Subtract() -> (x-y=w2909:dbl)  [unwired: 2 in]
                      n2108 = Divide(x=w2909, y=2.0) -> (x/y=w2907:dbl)
                      n2109 = Absolute Value(x=w2907) -> (abs(x)=w2906:dbl)
                      n2110 = Add(y=w2906) -> (x+y=w2905:dbl)  [unwired: 1 in]
                      n2111 = Array Max & Min(array=w2913) -> (max value=w2912:sgl)  [unwired: 3 out]
                      n2112 = Array Max & Min(array=w2914) -> (max value=w2915:sgl)  [unwired: 3 out]
                      n2113 = Subtract(x=w2912, y=w2902) -> (x-y=w2911:dbl)
                      n2114 = Subtract(x=w2915, y=w2903) -> (x-y=w2916:dbl)
                      n2115 = Greater?(x=w2911) -> (0:w2910:bool)  [unwired: 1 in]
                      n2116 = case shown="True" w2910 {
                        frame False {
                        }
                        frame True {
                          n2117 = local write "Masking light"(FALSE ("Masking light")) -> ()
                        }
                      }
                      n2118 = Greater?(x=w2916) -> (0:w2918:bool)  [unwired: 1 in]
                      n2119 = Less?(x=w2916, y=w2905) -> (x < y?=w2917:bool)
                      n2120 = And(x=w2917, y=w2918) -> (x .and. y?=w2904:bool)
                    }
                    frame True {
                      n2121 = local read "Track position"() -> (w2927:sgl)
                      n2122 = local read "Track position"() -> (w2928:sgl)
                      n2123 = local read "Track position"() -> (w2924:sgl)
                      n2124 = local read item#-1() -> ()  [unwired: 1 out]
                      n2125 = local read item#-1() -> ()  [unwired: 1 out]
                      n2126 = local read item#-1() -> ()  [unwired: 1 out]
                      n2127 = Add(y=15.0) -> (x+y=w2920:dbl)  [unwired: 1 in]
                      n2128 = Less?(x=w2928, y=w2920) -> (x < y?=w2925:bool)
                      n2129 = Greater?(x=w2924) -> (0:w2923:bool)  [unwired: 1 in]
                      n2130 = Greater?(x=w2927) -> (0:w2926:bool)  [unwired: 1 in]
                      n2131 = case shown="True" w2926 {
                        frame False {
                        }
                        frame True {
                          n2132 = local write "Masking light"(FALSE ("Masking light")) -> ()
                        }
                      }
                      n2133 = And(x=w2925, y=w2923) -> (x .and. y?=w2922:bool)
                    }
                  }
                  n2134 = Wait (ms)(milliseconds to wait=u32 10) -> ()  [unwired: 1 out]
                  n2135 = local read "Primary masking light"() -> (w2892:T3)
                  n2136 = case shown="True" w2896 {
                    frame False {
                    }
                    frame True {
                      n2137 = local write "Masking light"(TRUE ("Masking light")) -> ()
                    }
                  }
                  n2138 = local read "Masking light"() -> (w2894:bool)
                  n2139 = Not Equal?(x=w2892, y=T13."Continuous specified all trials") -> (x != y?=w2891:bool)
                  n2140 = local read "Exit"() -> (w2893:bool)
                  n2141 = call-poly <vilib>:"DAQmx Write.vi"("task/channels in"=w2901, "data"=w2894, "error in"=w2900) -> ("task out"=w2899:refnum<k21>, "error out"=w2898:errorcluster)  [unwired: 10 in, 1 out]
                  n2142 = Compound Arithmetic op=OR(w2891, w2893) -> (w2890:bool)
                }
              }
              frame Enabled {
              }
            }
            n2143 = local read "Primary masking light"() -> (w2875:T3)
            n2144 = Equal?(x=w2875, y=w2873) -> (x = y?=w2876:bool)
            n2145 = Select(t=w2875, s=w2876, f=T13."None") -> (s? t:f=w2874:T3)
            n2146 = call <vilib>:"DAQmx Stop Task.vi"("task/channels in"=w2877, "error in"=w2878) -> ("task out"=w2880:refnum<k21>, "error out"=w2879:errorcluster)  [unwired: 12 in]
          }
        }
        n2147 = local read "Exit"() -> (w2472:bool)
      }
      n2148 = call <vilib>:"DAQmx Clear Task.vi"("task in"=w2454, "error in"=w2453) -> ()  [unwired: 13 in, 1 out]
    }
  }
  n2149 = local write "Reset bottom plot"(w80) -> ()
  n2150 = local write "Reset wheel pos. graph"(w80) -> ()
  n2151 = local write "Reset top plot"(w80) -> ()
  n2152 = local write "Random reward"(FALSE ("Random reward")) -> ()
  n2153 = local read "Run experiment"() -> (w24:bool)
  n2154 = disable-structure shown="Disabled" {
    disable-tunnel: w24 -> [w3086 _]
    frame Disabled {
      n2155 = case shown="True" w3086 {
        frame False {
        }
        frame True {
          # "Light ON/OFF  indicators"
          # "Trial type indicators"
          n2156 = local read "shuffled array"() -> (w3093:i16[])
          n2157 = local read "All trials"() -> (w3094:i32)
          n2158 = local read "shuffled array"() -> (w3146:i16[])
          n2159 = local read "shuffled array"() -> (w3101:i16[])
          n2160 = local read "Stim types"() -> (w3147:u16[])
          n2161 = local read "Stim types"() -> (w3100:u16[])
          n2162 = local read "Stim types"() -> (w3091:u16[])
          n2163 = Quotient & Remainder(x=w3094, y=5.0) -> (x-y*floor(x/y)=w3092:dbl)  [unwired: 1 out]
          n2164 = Index Array(array=w3093, index=w3092) -> (element=w3090:i16)
          n2165 = Index Array(array=w3147, index=0 ("index (row)")) -> (element=w3140:u16)
          n2166 = Index Array(array=w3100, index=1 ("index (row)")) -> (element=w3107:u16)
          n2167 = Index Array(array=w3146, index=0) -> (element=w3145:i16)
          n2168 = Index Array(array=w3146, index=1) -> (element=w3141:i16)
          n2169 = Index Array(array=w3146, index=2) -> (element=w3142:i16)
          n2170 = Index Array(array=w3146, index=3) -> (element=w3143:i16)
          n2171 = Index Array(array=w3146, index=4) -> (element=w3144:i16)
          n2172 = Index Array(array=w3101, index=0) -> (element=w3102:i16)
          n2173 = Index Array(array=w3101, index=1) -> (element=w3106:i16)
          n2174 = Index Array(array=w3101, index=2) -> (element=w3105:i16)
          n2175 = Index Array(array=w3101, index=3) -> (element=w3104:i16)
          n2176 = Index Array(array=w3101, index=4) -> (element=w3103:i16)
          n2177 = Index Array(array=w3091, index (row)=0, index (col)=w3090) -> (element=w3087:u16)
          n2178 = Index Array(array=w3140, index=w3145) -> (element=w3139)
          n2179 = Index Array(array=w3140, index=w3141) -> (element=w3138)
          n2180 = Index Array(array=w3140, index=w3142) -> (element=w3137)
          n2181 = Index Array(array=w3140, index=w3143) -> (element=w3135)
          n2182 = Index Array(array=w3140, index=w3144) -> (element=w3136)
          n2183 = Index Array(array=w3107, index=w3102) -> (element=w3108)
          n2184 = Index Array(array=w3107, index=w3106) -> (element=w3109)
          n2185 = Index Array(array=w3107, index=w3105) -> (element=w3110)
          n2186 = Index Array(array=w3107, index=w3104) -> (element=w3112)
          n2187 = Index Array(array=w3107, index=w3103) -> (element=w3111)
          n2188 = Number To Boolean Array(number=w3087) -> (Boolean array=w3155:bool[])
          n2189 = Number To Boolean Array(number=w3139) -> (Boolean array=w3148:bool[])
          n2190 = Number To Boolean Array(number=w3137) -> (Boolean array=w3151:bool[])
          n2191 = Number To Boolean Array(number=w3135) -> (Boolean array=w3150:bool[])
          n2192 = Number To Boolean Array(number=w3136) -> (Boolean array=w3152:bool[])
          n2193 = Number To Boolean Array(number=w3108) -> (Boolean array=w3099:bool[])
          n2194 = Number To Boolean Array(number=w3110) -> (Boolean array=w3096:bool[])
          n2195 = Number To Boolean Array(number=w3112) -> (Boolean array=w3097:bool[])
          n2196 = Number To Boolean Array(number=w3111) -> (Boolean array=w3095:bool[])
          n2197 = Number To Boolean Array(number=w3138) -> (Boolean array=w3149:bool[])
          n2198 = Number To Boolean Array(number=w3109) -> (Boolean array=w3098:bool[])
          n2199 = Index Array(array=w3155, index=0) -> (element=→"Next":bool)
          n2200 = Index Array(array=w3148, index=0) -> ()  [unwired: 1 out]
          n2201 = Index Array(array=w3149, index=0) -> ()  [unwired: 1 out]
          n2202 = Index Array(array=w3151, index=0) -> ()  [unwired: 1 out]
          n2203 = Index Array(array=w3150, index=0) -> ()  [unwired: 1 out]
          n2204 = Index Array(array=w3152, index=0) -> ()  [unwired: 1 out]
          n2205 = Index Array(array=w3099, index=0) -> ()  [unwired: 1 out]
          n2206 = Index Array(array=w3098, index=0) -> ()  [unwired: 1 out]
          n2207 = Index Array(array=w3096, index=0) -> ()  [unwired: 1 out]
          n2208 = Index Array(array=w3097, index=0) -> ()  [unwired: 1 out]
          n2209 = Index Array(array=w3095, index=0) -> ()  [unwired: 1 out]
          n2210 = local read item#-1() -> ()  [unwired: 1 in]
          n2211 = local read item#-1() -> ()  [unwired: 1 in]
          n2212 = local read item#-1() -> ()  [unwired: 1 in]
          n2213 = local read item#-1() -> ()  [unwired: 1 in]
          n2214 = local read item#-1() -> ()  [unwired: 1 in]
          n2215 = local read item#-1() -> ()  [unwired: 1 in]
          n2216 = local read item#-1() -> ()  [unwired: 1 in]
          n2217 = local read item#-1() -> ()  [unwired: 1 in]
          n2218 = local read item#-1() -> ()  [unwired: 1 in]
          n2219 = local read item#-1() -> ()  [unwired: 1 in]
        }
      }
    }
    frame Enabled {
    }
  }
  "Tab Control hidden Variables" <- enum32{"Test charts", "Variables"}."Test charts" ("Tab Control 5")
